vi "設定項目.vi"() -> (15 "品番・品名クラスタ_設定 _表示器":T3)   [LabVIEW 2021]
uses:
  <vilib>/Utility/config.llb/Read Key (String).vi
  <vilib>/Utility/config.llb/Read Key (U32).vi
  <vilib>/Utility/config.llb/Read Key (I32).vi
  <vilib>/Utility/config.llb/Read Key (Boolean).vi
  <vilib>/Utility/config.llb/Read Key (Path).vi
  <vilib>/Utility/config.llb/Write Key (String).vi
  <vilib>/Utility/config.llb/Write Key (Double).vi
  <vilib>/Utility/config.llb/Write Key (U32).vi
  <vilib>/Utility/config.llb/Write Key (Boolean).vi
  <vilib>/Utility/config.llb/Write Key (Path).vi
  <vilib>/Utility/config.llb/NI_LVConfig.lvlib
panel:
  out "ゲージ確認ボタンBOOL":bool
  in  "書込周期/ms":dbl
  in  "CSV項目名_リセット用":T1
  in  "CSV保存名_リセット用":string
  in  "② CSV保存名":string
  out "値転記用配列":T2[](array[typedef]) {"測定モード" items=["単発測定モード", "連続測定モード", "多点測定モード"]}
  out "G_メイン測定キャンセルボタン":bool
  in  "ゲージ確認ボタン":bool
  in  "測定ゲージ数":dbl
  in  "測定周期/ms":dbl
  in  "iniRエラーin 2":errorcluster caption="エラー入力（エラーなし）"
  out "iniエラーout":errorcluster caption="エラー入力（エラーなし）"
  in  "error in (no error)":errorcluster caption="エラー入力（エラーなし）"
  out "iniフォルダパス取得":path
  out "キューのエラー":errorcluster caption="エラー出力"
  in  "設定クラスタ_リセット":T4 {"測定モード" items=["単発測定モード", "連続測定モード"]}
  in  "CSV保存先フォルダ_リセット用":path
  in  "CSV保存先フォルダ":path
  in  "品番・品名_リセット用":T3
  in  "品番・品名クラスタ_設定":T3
  in  "使用ON/OFFボタン_リセット用":T5
  in  "初期化ボタン":bool
  in  "キャンセルして戻るボタン":bool
  in  "登録ボタン":bool
  out "iniRエラーout 2":errorcluster caption="エラー入力（エラーなし）"
  in  "CSV項目名 12":T1
  in  "CSV項目名 11":T1
  in  "CSV項目名 10":T1
  in  "CSV項目名 9":T1
  in  "CSV項目名 8":T1
  in  "CSV項目名 7":T1
  in  "CSV項目名 6":T1
  in  "CSV項目名 5":T1
  in  "CSV項目名 4":T1
  in  "CSV項目名 3":T1
  in  "CSV項目名 2":T1
  in  "CSV項目名 1":T1
  in  "設定クラスタ_設定 12":T2 {"測定モード" items=["単発測定モード", "連続測定モード", "多点測定モード"]}
  in  "使用ON/OFFボタン_設定 12":T5
  in  "キャンセルボタン 12":T6
  in  "No設定クラスタ_設定 12":T7
  in  "設定クラスタ_設定 11":T2 {"測定モード" items=["単発測定モード", "連続測定モード", "多点測定モード"]}
  in  "使用ON/OFFボタン_設定 11":T5
  in  "キャンセルボタン 11":T6
  in  "No設定クラスタ_設定 11":T7
  in  "設定クラスタ_設定 10":T2 {"測定モード" items=["単発測定モード", "連続測定モード", "多点測定モード"]}
  in  "使用ON/OFFボタン_設定 10":T5
  in  "キャンセルボタン 10":T6
  in  "No設定クラスタ_設定 10":T7
  in  "設定クラスタ_設定 9":T2 {"測定モード" items=["単発測定モード", "連続測定モード", "多点測定モード"]}
  in  "使用ON/OFFボタン_設定 9":T5
  in  "キャンセルボタン 9":T6
  in  "No設定クラスタ_設定 9":T7
  in  "設定クラスタ_設定 8":T2 {"測定モード" items=["単発測定モード", "連続測定モード", "多点測定モード"]}
  in  "使用ON/OFFボタン_設定 8":T5
  in  "キャンセルボタン 8":T6
  in  "No設定クラスタ_設定 8":T7
  in  "設定クラスタ_設定 7":T2 {"測定モード" items=["単発測定モード", "連続測定モード", "多点測定モード"]}
  in  "使用ON/OFFボタン_設定 7":T5
  in  "キャンセルボタン 7":T6
  in  "No設定クラスタ_設定 7":T7
  in  "設定クラスタ_設定 6":T2 {"測定モード" items=["単発測定モード", "連続測定モード", "多点測定モード"]}
  in  "使用ON/OFFボタン_設定 6":T5
  in  "キャンセルボタン 6":T6
  in  "No設定クラスタ_設定 6":T7
  in  "設定クラスタ_設定 5":T2 {"測定モード" items=["単発測定モード", "連続測定モード", "多点測定モード"]}
  in  "使用ON/OFFボタン_設定 5":T5
  in  "キャンセルボタン 5":T6
  in  "No設定クラスタ_設定 5":T7
  in  "設定クラスタ_設定 4":T2 {"測定モード" items=["単発測定モード", "連続測定モード", "多点測定モード"]}
  in  "使用ON/OFFボタン_設定 4":T5
  in  "キャンセルボタン 4":T6
  in  "No設定クラスタ_設定 4":T7
  in  "設定クラスタ_設定 3":T2 {"測定モード" items=["単発測定モード", "連続測定モード", "多点測定モード"]}
  in  "使用ON/OFFボタン_設定 3":T5
  in  "キャンセルボタン 3":T6
  in  "No設定クラスタ_設定 3":T7
  in  "設定クラスタ_設定 2":T2 {"測定モード" items=["単発測定モード", "連続測定モード", "多点測定モード"]}
  in  "使用ON/OFFボタン_設定 2":T5
  in  "キャンセルボタン 2":T6
  in  "No設定クラスタ_設定 2":T7
  in  "設定クラスタ_設定1":T2 {"測定モード" items=["単発測定モード", "連続測定モード", "多点測定モード"]}
  in  "キャンセルボタン1":T6
  in  "使用ON/OFFボタン_設定1":T5
  in  "No設定クラスタ_設定1":T7
  # "設定項目画面"
  # "データ収集タイミング"
  # "※全入力クリアボタンでリセットしない仕様です。"
  # "①"
  # "⑬\n測定画面\nON/OFF"
  # "⑦規格"
  # "⑨上限"
  # "⑪同時測定\nゲージNO."
  # "⑭ゲージ\nポートNo."
  # "入力\nクリア"
  # "⑮測定\nON/OFF"
  # "⑯CSVヘッダー名"
  # "⑤No."
  # "⑥品質チェック項目"
  # "⑫測定モード"
  # "値"
  # "⑧単位"
  # "⑩下限"
  # "-"
  # "品番"
  # "品名"
  # "-"
  # "品番"
  # "品名"
  # "-"
  # "品番"
  # "品名"
  # "③"
  # "④"
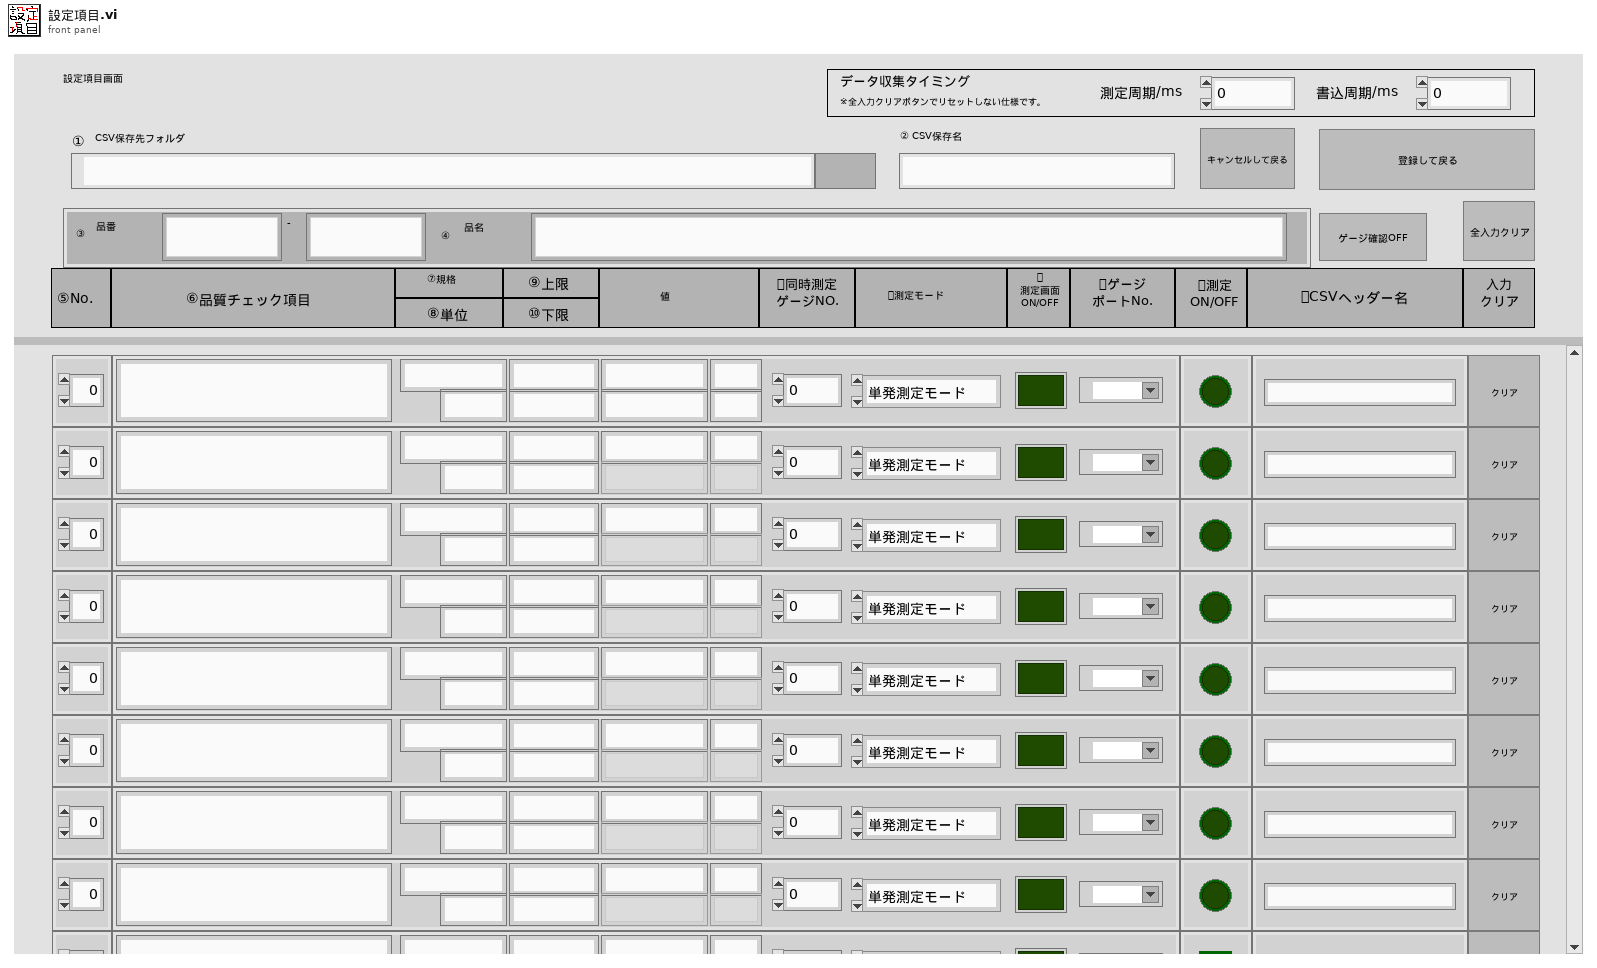
[diagram p1: front panel]
types:
  T1 = typedef "CSV項目名入力.ctl" = cluster{"CSV項目名":string}
  T2 = typedef "設定全項目制御器.ctl" = cluster{"規格":string, "規格上限":string, "規格下限":string, "ポートNo.":dbl, "測定モード":u16, "規格単位":string, "品質チェック項目":string, "測定周期":dbl, "実測値MAX":string, "実測値MIN":string, "実測値(MAX)":string, "実測値(MIN)":string, "測定画面表示ボタン":bool, "ゲージポートNo":refnum<visa-resource-name>}
  T3 = typedef "品番・品名選択用.ctl" = cluster{"品名":string, "品番前":string, "品番後":string}
  T4 = cluster{"規格":string, "規格上限":string, "規格下限":string, "ポートNo.":dbl, "測定モード":u16, "規格単位":string, "品質チェック項目":string, "測定周期":dbl, "実測値MAX":string, "実測値MIN":string, "実測値(MAX)":string, "実測値(MIN)":string, "測定画面表示ボタン":bool, "ゲージポートNo":refnum<visa-resource-name>}
  T5 = typedef "ONOFFボタン制御器.ctl" = cluster{"使用ON/OFF":bool}
  T6 = typedef "キャンセルボタン制御器.ctl" = bool
  T7 = typedef "CH設定表示器.ctl" = cluster{"No. ":dbl}
  T8 = enum8{"Enabled", "Disabled", "Disabled and Grayed Out"}
  T9 = typedef "NI_LVConfig.lvlib/Config Data RefNum.ctl" = refnum<k1>
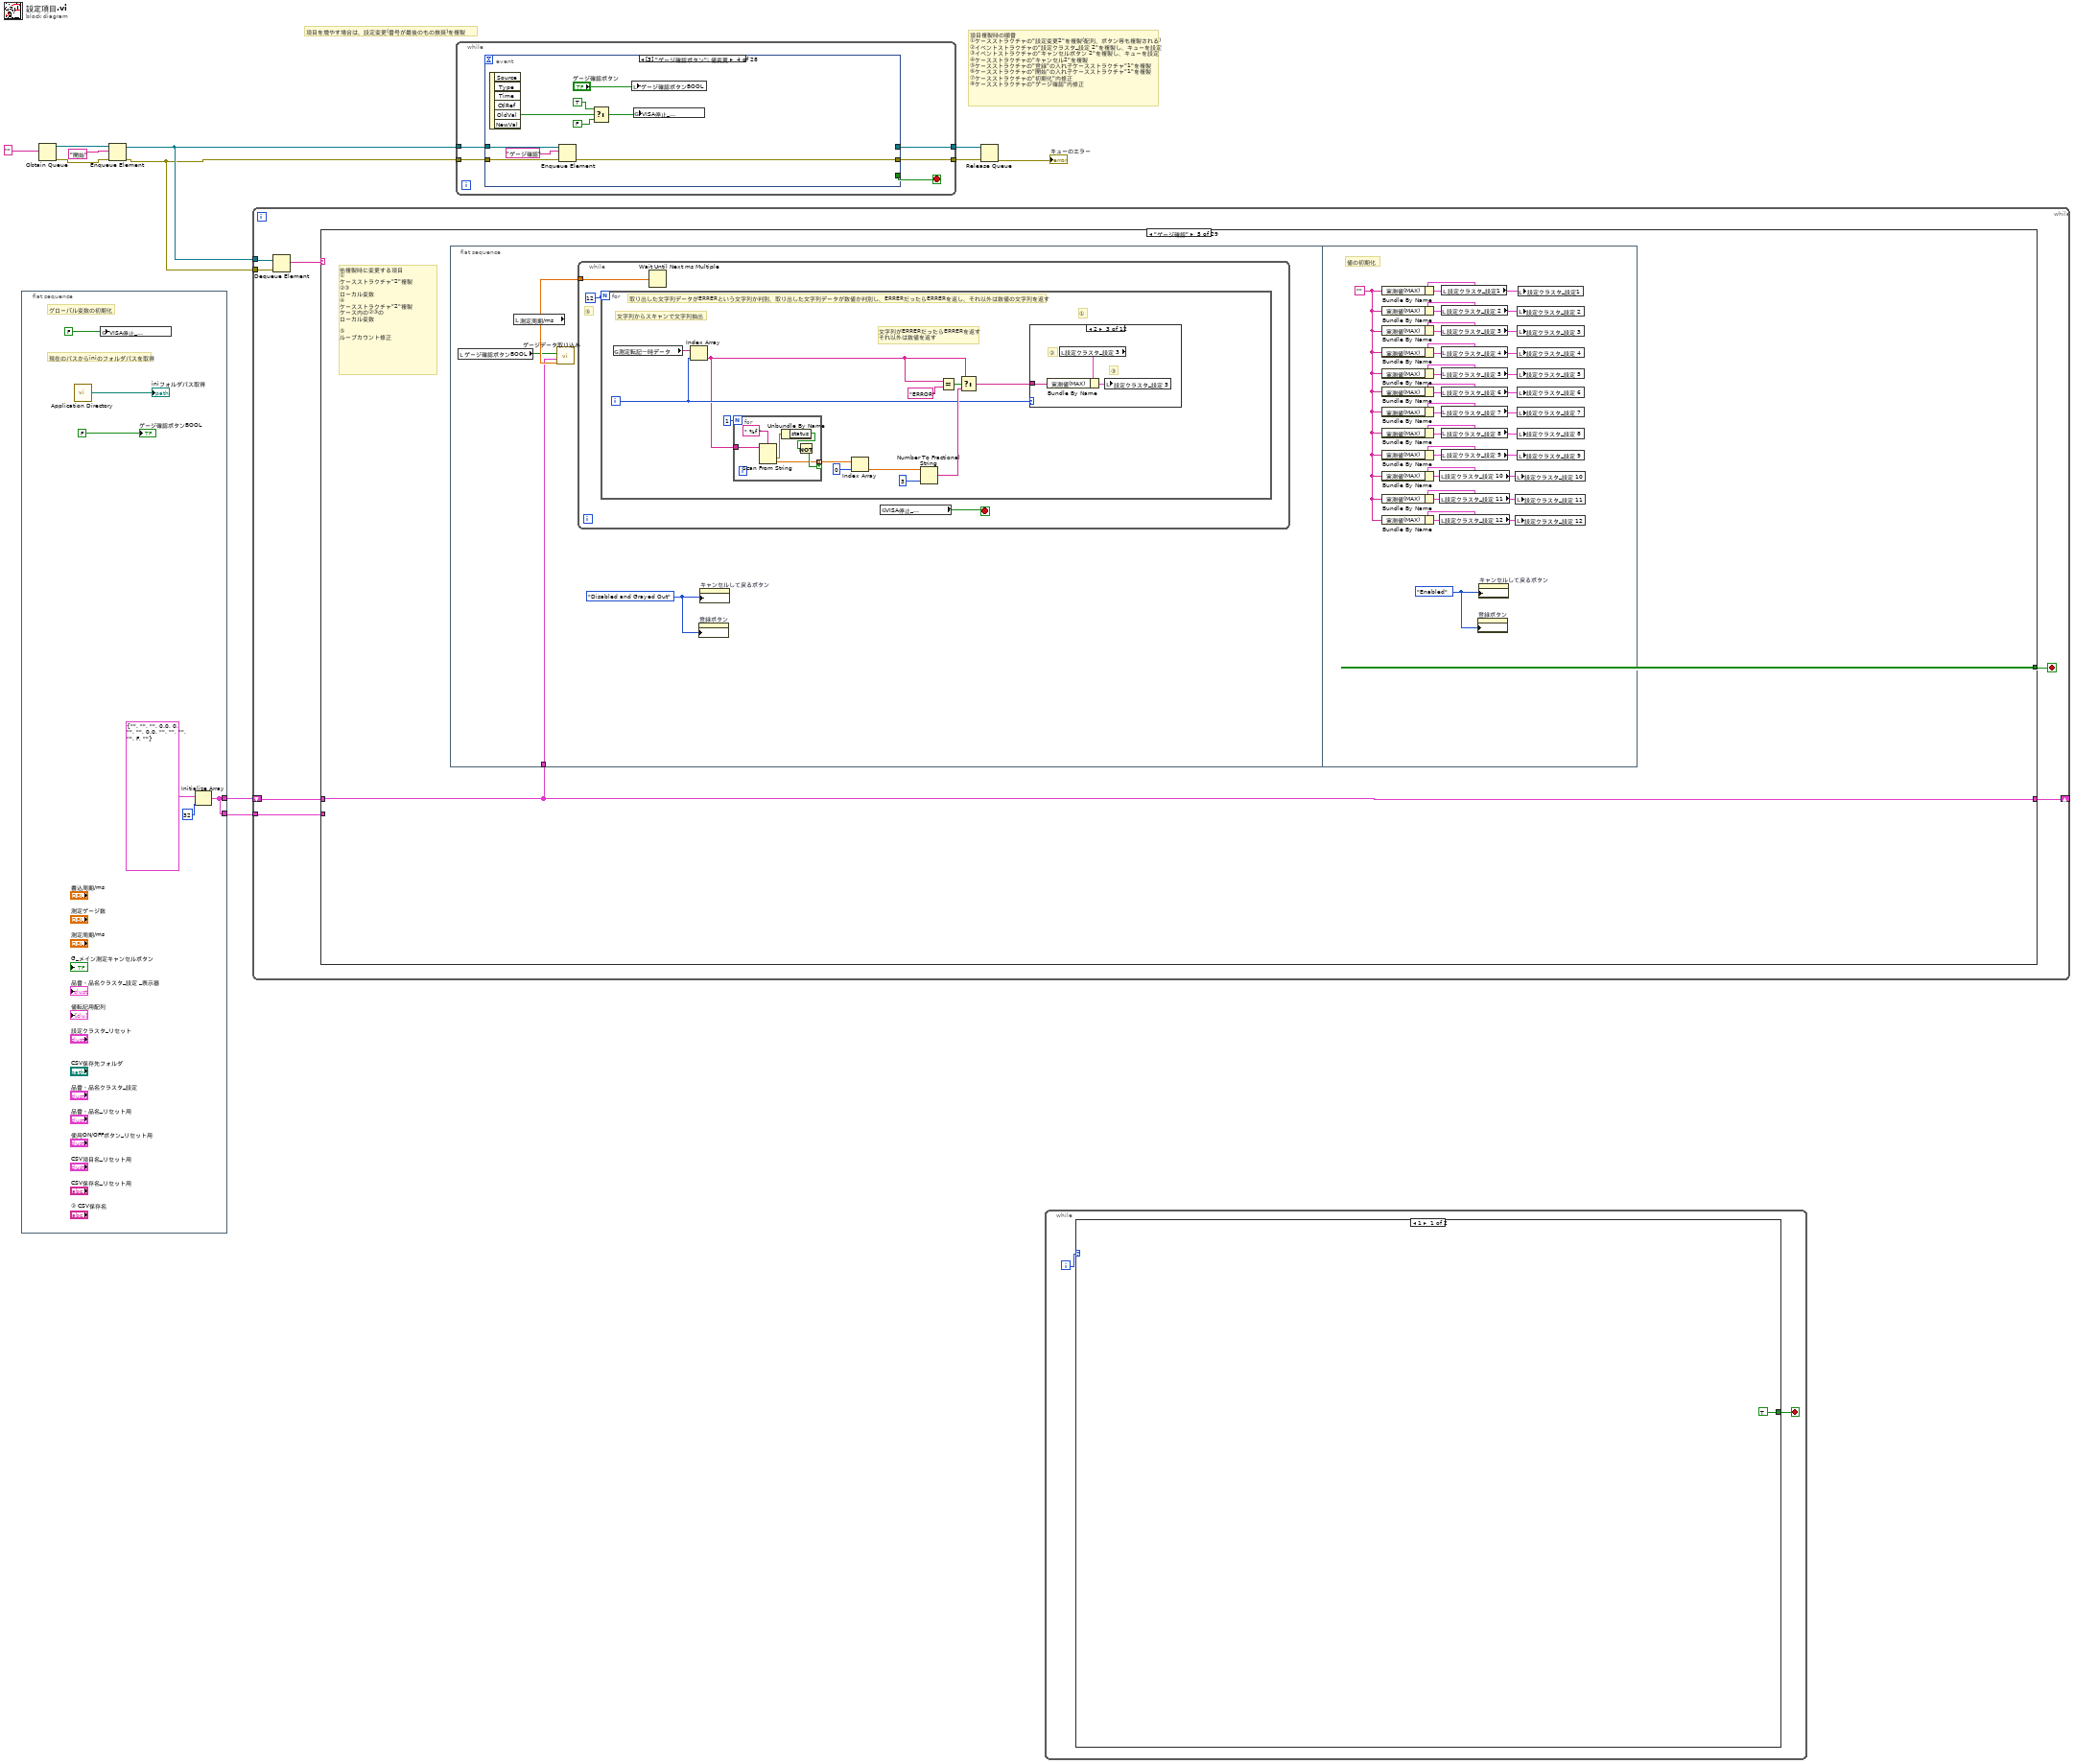
[diagram p0: block diagram]
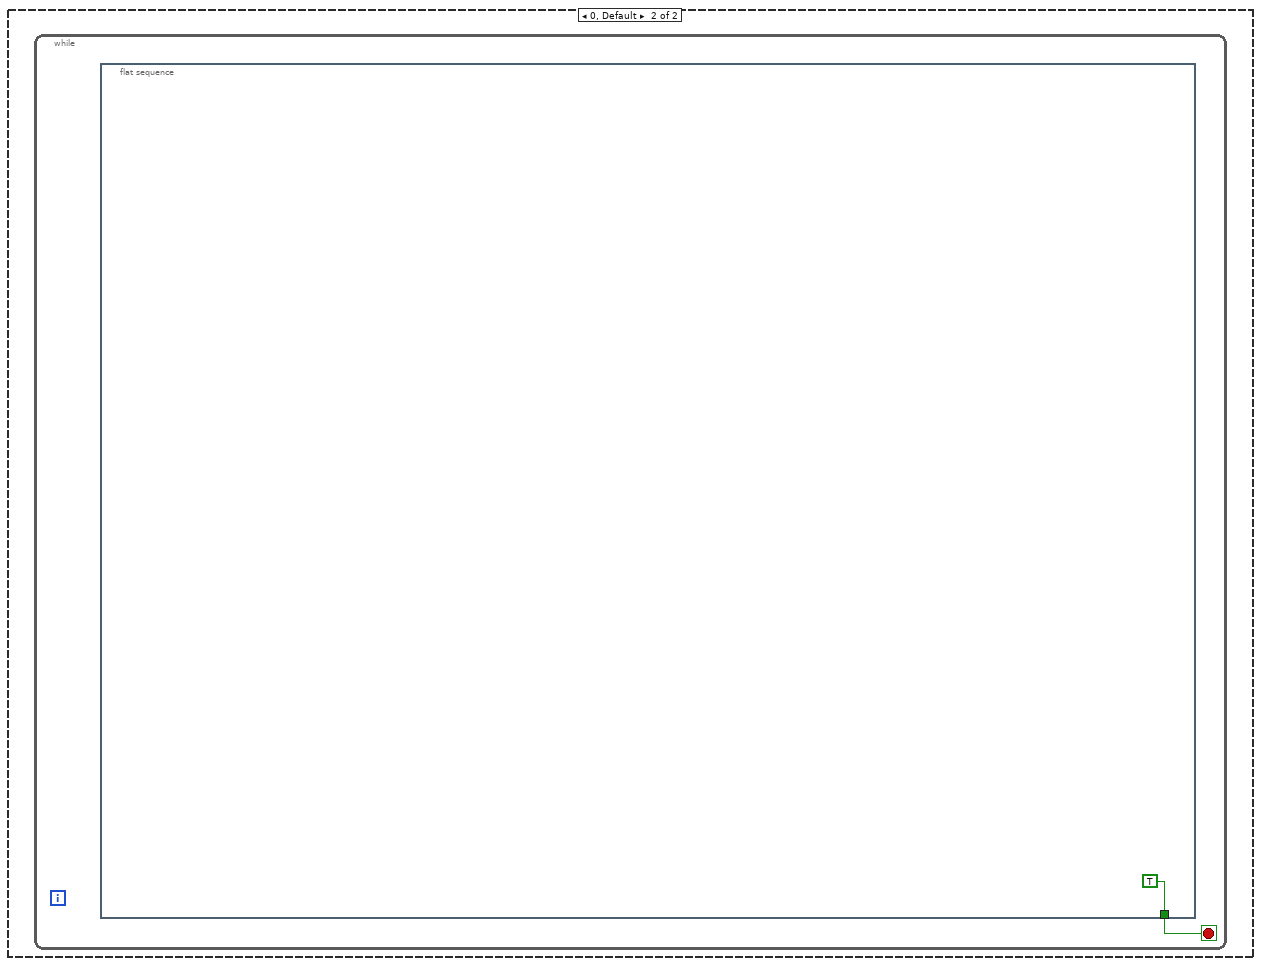
[diagram p2: hidden frame]
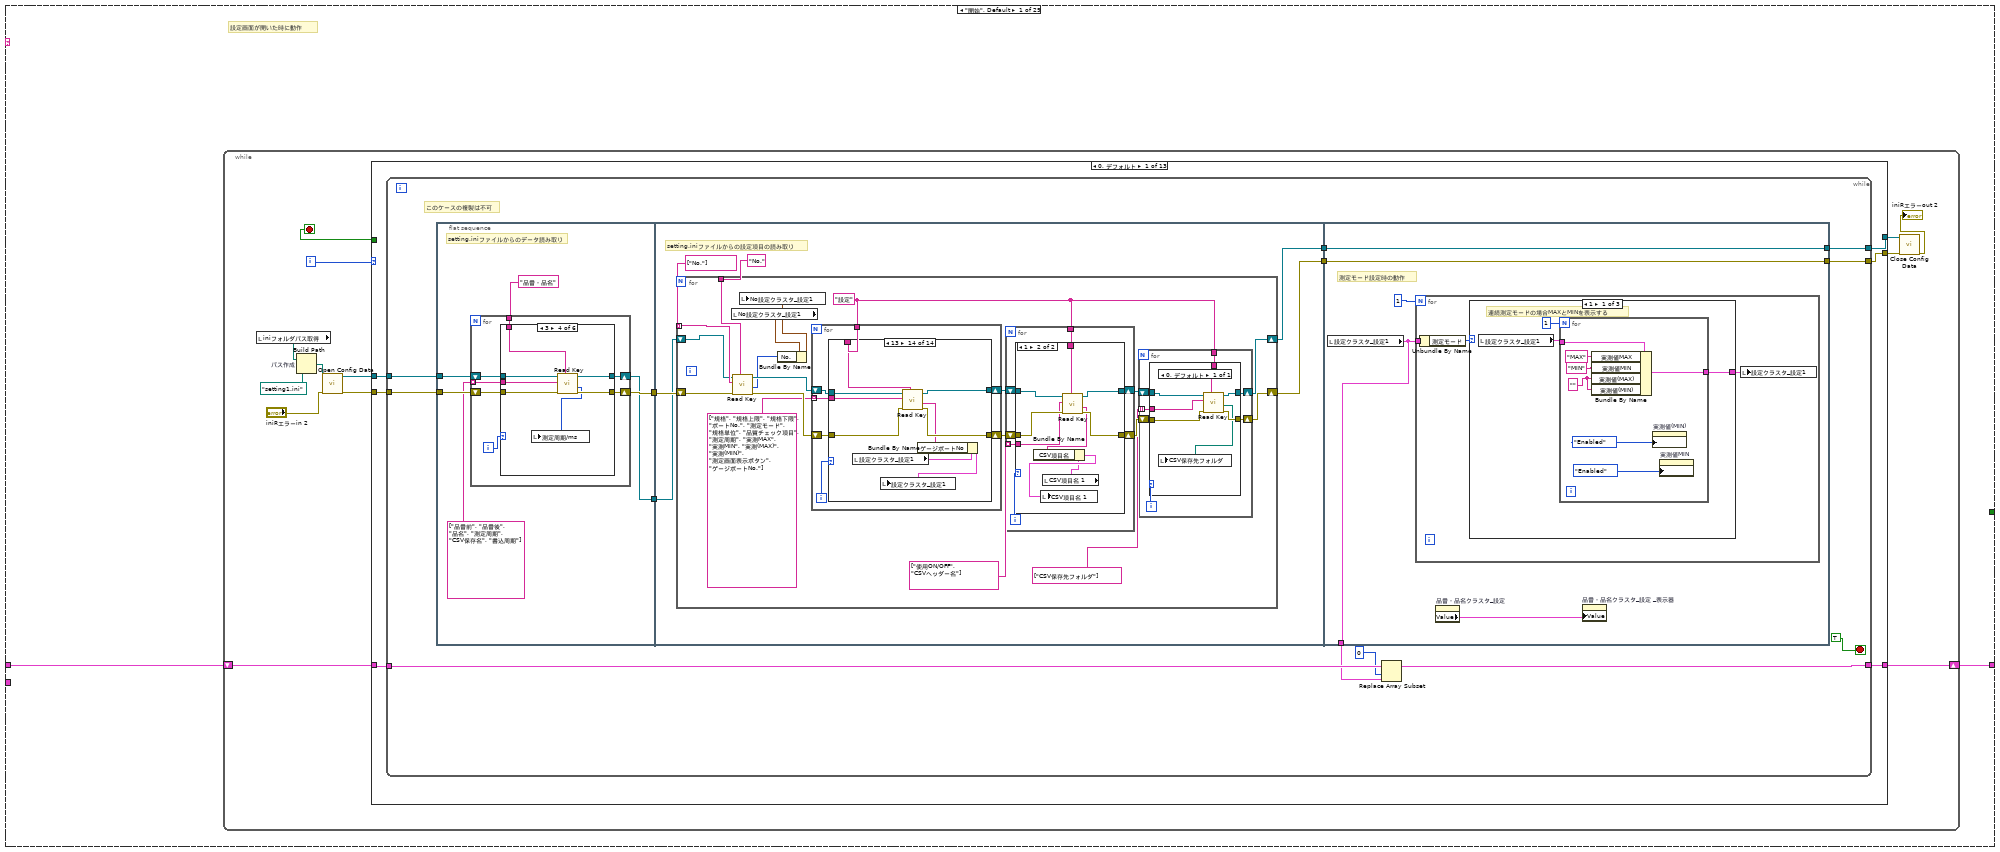
[diagram p3: hidden frame]
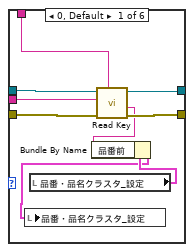
[diagram p4: hidden frame]
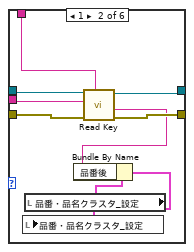
[diagram p5: hidden frame]
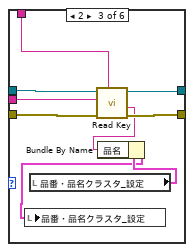
[diagram p6: hidden frame]
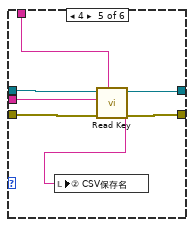
[diagram p7: hidden frame]
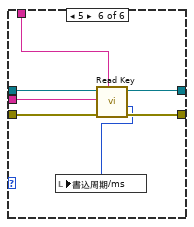
[diagram p8: hidden frame]
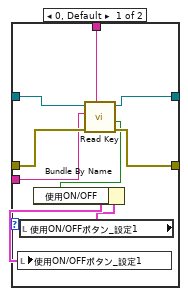
[diagram p9: hidden frame]
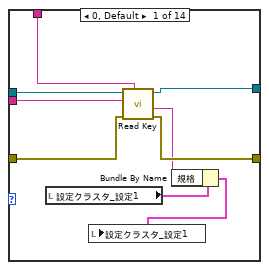
[diagram p10: hidden frame]
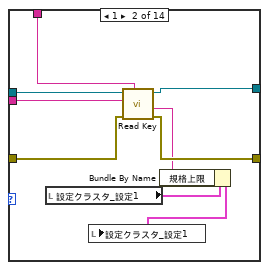
[diagram p11: hidden frame]
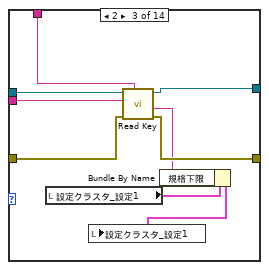
[diagram p12: hidden frame]
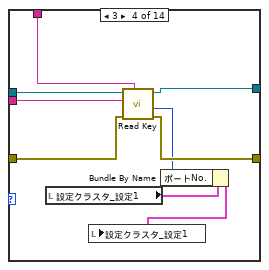
[diagram p13: hidden frame]
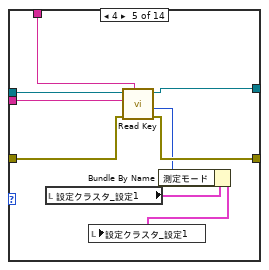
[diagram p14: hidden frame]
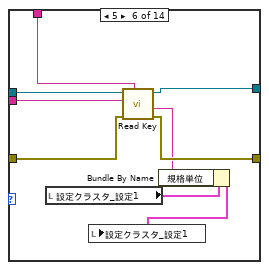
[diagram p15: hidden frame]
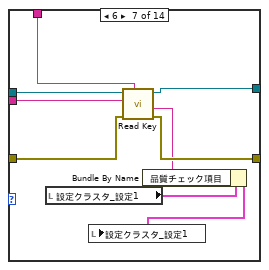
[diagram p16: hidden frame]
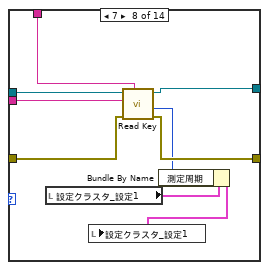
[diagram p17: hidden frame]
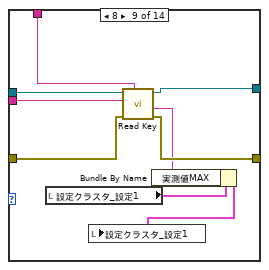
[diagram p18: hidden frame]
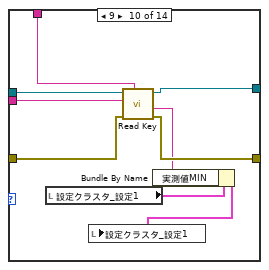
[diagram p19: hidden frame]
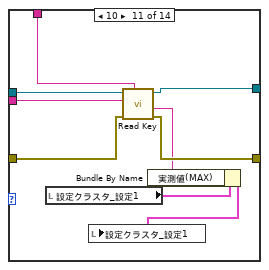
[diagram p20: hidden frame]
diagram:
  # "項目複製時の順番\n①ケースストラクチャの\"設定変更2\"を複製(配列、ボタン等も複製される)\n②イベントストラクチャの\"設定クラスタ_設定 2\"を複製し、キューを設定\n③イベントストラクチャの\"キャンセルボタン 2\"を複製し、キューを設定\n④ケースストラクチャの\"キャンセル2\"を複製\n⑤ケースストラクチャの\"登録\"の入れ子ケースストラクチャ\"1\"を複製\n⑥ケースストラクチャの\"開始\"の入れ子ケースストラクチャ\"1\"を複製\n⑦ケースストラクチャの\"初期化\"内修正\n⑧ケースストラクチャの\"ゲージ確認\"内修正"
  # "項目を増やす場合は、設定変更(番号が最後のもの推奨)を複製"
  n1 = flat-sequence {
    tunnel: [w14] -> w8
    tunnel: [w14] -> w7
    frame #0 {
      # "グローバル変数の初期化"
      # "現在のパスからiniのフォルダパスを取得"
      n2 = call <vilib>:"Application Directory.vi"() -> ("Application Directory"=→"iniフォルダパス取得":path)
      n3 = global write "VISA停止_G.vi" "VISA停止_\nグローバル"(FALSE) -> ()
      n4 = Initialize Array(T2 {"規格"="", "規格上限"="", "規格下限"="", "ポートNo."=0.0, "測定モード"=0, "規格単位"="", "品質チェック項目"="", "測定周期"=0.0, "実測値MAX"="", "実測値MIN"="", "実測値(MAX)"="", "実測値(MIN)"="", "測定画面表示ボタン"=FALSE, "ゲージポートNo"=""} ("メイン設定_設定"), 32) -> (w14:T2[])
      "ゲージ確認ボタンBOOL" <- FALSE
    }
  }
  n5 = Obtain Queue(element data type="") -> (queue out=w3:refnum<queue>, error out=w1:errorcluster)  [unwired: 4 in, 1 out]
  n6 = Enqueue Element(queue=w3, element="開始", error in (no error)=w1) -> (queue out=w6:refnum<queue>, error out=w5:errorcluster)  [unwired: 1 in, 1 out]
  n7 = while {
    tunnel: w6 -> [w23]
    tunnel: w5 -> [w21]
    shift-right: [w19] -> _
    shift-left: w8 -> [w20]
    tunnel: w7 -> [w18]
    stop <- w22 stop-if-true
    n8 = Dequeue Element(queue=w23, error in (no error)=w21) -> (element=w24:string)  [unwired: 1 in, 3 out]
    n9 = case shown="\"ゲージ確認\"" w24 {
      tunnel: [_ TRUE TRUE _ _ _ _ _ _ _ _ _ _ _ _ _ _ _ _ _ _ _ _ _ _ _ _ _ _] -> w22
      tunnel: w20 -> [w26 w2548 _ _ w3041 w3133 w3139 w3145 w3151 w3157 w3163 w3169 w3175 w3181 w3187 w3193 w3199 w3204 w3245 w3285 w3325 w3365 w3405 w3445 w3485 w3525 w3565 w3605 w3645]
      tunnel: [w25 w2547 _ w3038 w3041 w3132 w3138 w3144 w3150 w3156 w3162 w3168 w3174 w3180 w3186 w3192 w3198 w3201 w3242 w3282 w3322 w3362 w3402 w3442 w3482 w3522 w3562 w3602 w3642] -> w19
      tunnel: w18 -> [_ _ _ w3038 _ _ _ _ _ _ _ _ _ _ _ _ _ _ _ _ _ _ _ _ _ _ _ _ _]
      frame "開始", Default {
        # "設定画面が開いた時に動作"
        n10 = while {
          shift-right: [w28] -> w25
          shift-left: w26 -> [w29]
          i -> [w39]
          stop <- w27 stop-if-true
          n11 = local read "iniフォルダパス取得"() -> (w38:path)
          n12 = Build Path "パス作成"(base path=w38, name or relative path=path "setting1.ini") -> (appended path=w37:path)
          n13 = call <vilib>:"Open Config Data.vi"("error in (no error)"="iniRエラーin 2", "configuration file path"=w37) -> ("error out"=w34:errorcluster, "refnum"=w33:T9)  [unwired: 1 in, 7 out]
          n14 = case shown="0, デフォルト" w39 {
            tunnel: w34 -> [w42 w365 w564 w763 w962 w1161 w1360 w1559 w1758 w1957 w2156 w2355 _]
            tunnel: w33 -> [w43 w364 w563 w762 w961 w1160 w1359 w1558 w1757 w1956 w2155 w2354 _]
            tunnel: [w44 w363 w562 w761 w960 w1159 w1358 w1557 w1756 w1955 w2154 w2353 _] -> w32
            tunnel: [w45 w362 w561 w760 w959 w1158 w1357 w1556 w1755 w1954 w2153 w2352 _] -> w31
            tunnel: w29 -> [w40 w360 w559 w758 w957 w1156 w1355 w1554 w1753 w1952 w2151 w2350 w2545]
            tunnel: [w41 w361 w560 w759 w958 w1157 w1356 w1555 w1754 w1953 w2152 w2351 w2545] -> w28
            tunnel: [_ _ _ _ _ _ _ _ _ _ _ _ TRUE] -> w27
            frame 0, Default {
              n15 = while {
                tunnel: [w57] -> w45
                tunnel: [w56] -> w44
                tunnel: w43 -> [w55]
                tunnel: w42 -> [w54]
                tunnel: [w53] -> w41
                tunnel: w40 -> [w52]
                stop <- TRUE stop-if-true
                # "このケースの複製は不可"
                n16 = flat-sequence {
                  tunnel: [w63] -> w51
                  tunnel: [w62] -> w50
                  tunnel: w55 -> [w61]
                  tunnel: w54 -> [w60]
                  tunnel: w51 -> [w123]
                  tunnel: w50 -> [w122]
                  tunnel: [w121] -> w49
                  tunnel: [w120] -> w48
                  tunnel: w49 -> [w320]
                  tunnel: [w320] -> w57
                  tunnel: w48 -> [w319]
                  tunnel: [w319] -> w56
                  tunnel: [w317] -> w47
                  frame #0 {
                    # "setting.iniファイルからのデータ読み取り"
                    n17 = for {
                      tunnel: string[] ["品番前", "品番後", "品名", "測定周期", "CSV保存名", "書込周期"] -> [w70] mode=indexing
                      shift-right: [w69] -> w62
                      shift-left: w61 -> [w68]
                      tunnel: "品番・品名" -> [w67]
                      shift-right: [w65] -> w63
                      shift-left: w60 -> [w66]
                      i -> [w71]
                      n18 = case shown="3" w71 {
                        tunnel: w70 -> [w80 w89 w98 w105 w112 w119]
                        tunnel: [w79 w87 w97 w104 w111 w118] -> w69
                        tunnel: w68 -> [w78 w88 w96 w103 w110 w117]
                        tunnel: w67 -> [w77 w86 w95 w102 w109 w116]
                        tunnel: w66 -> [w76 w85 w94 w101 w108 w115]
                        tunnel: [w75 w84 w93 w100 w107 w114] -> w65
                        frame 0, Default {
                          n19 = local read "品番・品名クラスタ_設定"() -> (w73:T3)
                          n20 = call-poly <vilib>:"Read Key.vi"("section"=w77, "error in (no error)"=w76, "key"=w80, "refnum"=w78) -> ("error out"=w75:errorcluster, "value"=w74:string, "refnum out"=w79:T9)  [unwired: 4 in, 1 out]
                          n21 = Bundle By Name(cluster=w73, "品番前"=w74) -> (w72:T3)
                          n22 = local write "品番・品名クラスタ_設定"(w72) -> ()
                        }
                        frame 1 {
                          n23 = local read "品番・品名クラスタ_設定"() -> (w82:T3)
                          n24 = call-poly <vilib>:"Read Key.vi"("section"=w86, "error in (no error)"=w85, "key"=w89, "refnum"=w88) -> ("error out"=w84:errorcluster, "value"=w83:string, "refnum out"=w87:T9)  [unwired: 4 in, 1 out]
                          n25 = Bundle By Name(cluster=w82, "品番後"=w83) -> (w81:T3)
                          n26 = local write "品番・品名クラスタ_設定"(w81) -> ()
                        }
                        frame 2 {
                          n27 = local read "品番・品名クラスタ_設定"() -> (w91:T3)
                          n28 = call-poly <vilib>:"Read Key.vi"("section"=w95, "error in (no error)"=w94, "key"=w98, "refnum"=w96) -> ("error out"=w93:errorcluster, "value"=w92:string, "refnum out"=w97:T9)  [unwired: 4 in, 1 out]
                          n29 = Bundle By Name(cluster=w91, "品名"=w92) -> (w90:T3)
                          n30 = local write "品番・品名クラスタ_設定"(w90) -> ()
                        }
                        frame 3 {
                          n31 = call-poly <vilib>:"Read Key.vi"("section"=w102, "error in (no error)"=w101, "key"=w105, "refnum"=w103) -> ("error out"=w100:errorcluster, "value"=w99:u32, "refnum out"=w104:T9)  [unwired: 4 in, 1 out]
                          n32 = local write "測定周期/ms"(w99) -> ()
                        }
                        frame 4 {
                          n33 = call-poly <vilib>:"Read Key.vi"("section"=w109, "error in (no error)"=w108, "key"=w112, "refnum"=w110) -> ("error out"=w107:errorcluster, "value"=w106:string, "refnum out"=w111:T9)  [unwired: 4 in, 1 out]
                          n34 = local write "② CSV保存名"(w106) -> ()
                        }
                        frame 5 {
                          n35 = call-poly <vilib>:"Read Key.vi"("section"=w116, "error in (no error)"=w115, "key"=w119, "refnum"=w117) -> ("error out"=w114:errorcluster, "value"=w113:u32, "refnum out"=w118:T9)  [unwired: 4 in, 1 out]
                          n36 = local write "書込周期/ms"(w113) -> ()
                        }
                      }
                    }
                  }
                  frame #1 {
                    # "setting.iniファイルからの設定項目の読み取り"
                    n37 = for {
                      shift-right: [w141] -> w121
                      shift-left: w122 -> [w142]
                      tunnel: string[] ["No."] -> [w144] mode=indexing
                      tunnel: "No." -> [w143]
                      shift-right: [w139] -> w120
                      shift-left: w123 -> [w140]
                      w128 = "設定"
                      n38 = local read "No設定クラスタ_設定1"() -> (w132:T7)
                      n39 = call-poly <vilib>:"Read Key.vi"("section"=w143, "error in (no error)"=w140, "key"=w144, "refnum"=w142) -> ("error out"=w136:errorcluster, "value"=w133:i32, "refnum out"=w138:T9)  [unwired: 4 in, 1 out]
                      n40 = Bundle By Name(cluster=w132, "No."=w133) -> (w134:T7)
                      n41 = local write "No設定クラスタ_設定1"(w134) -> ()
                      n42 = for {
                        shift-right: [w188] -> w137
                        shift-left: w138 -> [w190]
                        tunnel: w128 -> [w189]
                        shift-right: [w185] -> w135
                        shift-left: w136 -> [w186]
                        tunnel: string[] ["規格", "規格上限", "規格下限", "ポートNo.", "測定モード", "規格単位", "品質チェック項目", "測定周期", "実測MAX", "実測MIN", "実測(MAX)", "実測(MIN)", "測定画面表示ボタン", "ゲージポートNo."] -> [w184] mode=indexing
                        i -> [w187]
                        n43 = case shown="13" w187 {
                          tunnel: w190 -> [w199 w208 w217 w226 w235 w244 w253 w262 w271 w280 w289 w298 w307 w316]
                          tunnel: [w198 w207 w216 w225 w234 w243 w252 w261 w270 w279 w288 w297 w306 w315] -> w188
                          tunnel: w189 -> [w197 w206 w215 w224 w233 w242 w251 w260 w269 w278 w287 w296 w305 w314]
                          tunnel: w186 -> [w196 w205 w214 w223 w232 w241 w250 w259 w268 w277 w286 w295 w304 w313]
                          tunnel: [w195 w204 w213 w222 w231 w240 w249 w258 w267 w276 w285 w294 w303 w312] -> w185
                          tunnel: w184 -> [w191 w200 w209 w218 w227 w236 w245 w254 w263 w272 w281 w290 w299 w308]
                          frame 0, Default {
                            n44 = local read "設定クラスタ_設定1"() -> (w193:T2)
                            n45 = call-poly <vilib>:"Read Key.vi"("section"=w197, "error in (no error)"=w196, "key"=w191, "refnum"=w199) -> ("error out"=w195:errorcluster, "value"=w194:string, "refnum out"=w198:T9)  [unwired: 4 in, 1 out]
                            n46 = Bundle By Name(cluster=w193, "規格"=w194) -> (w192:T2)
                            n47 = local write "設定クラスタ_設定1"(w192) -> ()
                          }
                          frame 1 {
                            n48 = local read "設定クラスタ_設定1"() -> (w202:T2)
                            n49 = call-poly <vilib>:"Read Key.vi"("section"=w206, "error in (no error)"=w205, "key"=w200, "refnum"=w208) -> ("error out"=w204:errorcluster, "value"=w203:string, "refnum out"=w207:T9)  [unwired: 4 in, 1 out]
                            n50 = Bundle By Name(cluster=w202, "規格上限"=w203) -> (w201:T2)
                            n51 = local write "設定クラスタ_設定1"(w201) -> ()
                          }
                          frame 2 {
                            n52 = local read "設定クラスタ_設定1"() -> (w211:T2)
                            n53 = call-poly <vilib>:"Read Key.vi"("section"=w215, "error in (no error)"=w214, "key"=w209, "refnum"=w217) -> ("error out"=w213:errorcluster, "value"=w212:string, "refnum out"=w216:T9)  [unwired: 4 in, 1 out]
                            n54 = Bundle By Name(cluster=w211, "規格下限"=w212) -> (w210:T2)
                            n55 = local write "設定クラスタ_設定1"(w210) -> ()
                          }
                          frame 3 {
                            n56 = local read "設定クラスタ_設定1"() -> (w220:T2)
                            n57 = call-poly <vilib>:"Read Key.vi"("section"=w224, "error in (no error)"=w223, "key"=w218, "refnum"=w226) -> ("error out"=w222:errorcluster, "value"=w221:i32, "refnum out"=w225:T9)  [unwired: 4 in, 1 out]
                            n58 = Bundle By Name(cluster=w220, "ポートNo."=w221) -> (w219:T2)
                            n59 = local write "設定クラスタ_設定1"(w219) -> ()
                          }
                          frame 4 {
                            n60 = local read "設定クラスタ_設定1"() -> (w229:T2)
                            n61 = call-poly <vilib>:"Read Key.vi"("section"=w233, "error in (no error)"=w232, "key"=w227, "refnum"=w235) -> ("error out"=w231:errorcluster, "value"=w230:i32, "refnum out"=w234:T9)  [unwired: 4 in, 1 out]
                            n62 = Bundle By Name(cluster=w229, "測定モード"=w230) -> (w228:T2)
                            n63 = local write "設定クラスタ_設定1"(w228) -> ()
                          }
                          frame 5 {
                            n64 = local read "設定クラスタ_設定1"() -> (w238:T2)
                            n65 = call-poly <vilib>:"Read Key.vi"("section"=w242, "error in (no error)"=w241, "key"=w236, "refnum"=w244) -> ("error out"=w240:errorcluster, "value"=w239:string, "refnum out"=w243:T9)  [unwired: 4 in, 1 out]
                            n66 = Bundle By Name(cluster=w238, "規格単位"=w239) -> (w237:T2)
                            n67 = local write "設定クラスタ_設定1"(w237) -> ()
                          }
                          frame 6 {
                            n68 = local read "設定クラスタ_設定1"() -> (w247:T2)
                            n69 = call-poly <vilib>:"Read Key.vi"("section"=w251, "error in (no error)"=w250, "key"=w245, "refnum"=w253) -> ("error out"=w249:errorcluster, "value"=w248:string, "refnum out"=w252:T9)  [unwired: 4 in, 1 out]
                            n70 = Bundle By Name(cluster=w247, "品質チェック項目"=w248) -> (w246:T2)
                            n71 = local write "設定クラスタ_設定1"(w246) -> ()
                          }
                          frame 7 {
                            n72 = local read "設定クラスタ_設定1"() -> (w256:T2)
                            n73 = call-poly <vilib>:"Read Key.vi"("section"=w260, "error in (no error)"=w259, "key"=w254, "refnum"=w262) -> ("error out"=w258:errorcluster, "value"=w257:i32, "refnum out"=w261:T9)  [unwired: 4 in, 1 out]
                            n74 = Bundle By Name(cluster=w256, "測定周期"=w257) -> (w255:T2)
                            n75 = local write "設定クラスタ_設定1"(w255) -> ()
                          }
                          frame 8 {
                            n76 = local read "設定クラスタ_設定1"() -> (w265:T2)
                            n77 = call-poly <vilib>:"Read Key.vi"("section"=w269, "error in (no error)"=w268, "key"=w263, "refnum"=w271) -> ("error out"=w267:errorcluster, "value"=w266:string, "refnum out"=w270:T9)  [unwired: 4 in, 1 out]
                            n78 = Bundle By Name(cluster=w265, "実測値MAX"=w266) -> (w264:T2)
                            n79 = local write "設定クラスタ_設定1"(w264) -> ()
                          }
                          frame 9 {
                            n80 = local read "設定クラスタ_設定1"() -> (w274:T2)
                            n81 = call-poly <vilib>:"Read Key.vi"("section"=w278, "error in (no error)"=w277, "key"=w272, "refnum"=w280) -> ("error out"=w276:errorcluster, "value"=w275:string, "refnum out"=w279:T9)  [unwired: 4 in, 1 out]
                            n82 = Bundle By Name(cluster=w274, "実測値MIN"=w275) -> (w273:T2)
                            n83 = local write "設定クラスタ_設定1"(w273) -> ()
                          }
                          frame 10 {
                            n84 = local read "設定クラスタ_設定1"() -> (w283:T2)
                            n85 = call-poly <vilib>:"Read Key.vi"("section"=w287, "error in (no error)"=w286, "key"=w281, "refnum"=w289) -> ("error out"=w285:errorcluster, "value"=w284:string, "refnum out"=w288:T9)  [unwired: 4 in, 1 out]
                            n86 = Bundle By Name(cluster=w283, "実測値(MAX)"=w284) -> (w282:T2)
                            n87 = local write "設定クラスタ_設定1"(w282) -> ()
                          }
                          frame 11 {
                            n88 = local read "設定クラスタ_設定1"() -> (w292:T2)
                            n89 = call-poly <vilib>:"Read Key.vi"("section"=w296, "error in (no error)"=w295, "key"=w290, "refnum"=w298) -> ("error out"=w294:errorcluster, "value"=w293:string, "refnum out"=w297:T9)  [unwired: 4 in, 1 out]
                            n90 = Bundle By Name(cluster=w292, "実測値(MIN)"=w293) -> (w291:T2)
                            n91 = local write "設定クラスタ_設定1"(w291) -> ()
                          }
                          frame 12 {
                            n92 = local read "設定クラスタ_設定1"() -> (w301:T2)
                            n93 = call-poly <vilib>:"Read Key.vi"("section"=w305, "error in (no error)"=w304, "key"=w299, "refnum"=w307) -> ("error out"=w303:errorcluster, "value"=w302:bool, "refnum out"=w306:T9)  [unwired: 4 in, 1 out]
                            n94 = Bundle By Name(cluster=w301, "測定画面表示ボタン"=w302) -> (w300:T2)
                            n95 = local write "設定クラスタ_設定1"(w300) -> ()
                          }
                          frame 13 {
                            n96 = local read "設定クラスタ_設定1"() -> (w310:T2)
                            n97 = call-poly <vilib>:"Read Key.vi"("section"=w314, "error in (no error)"=w313, "key"=w308, "refnum"=w316) -> ("error out"=w312:errorcluster, "value"=w311:string, "refnum out"=w315:T9)  [unwired: 4 in, 1 out]
                            n98 = Bundle By Name(cluster=w310, "ゲージポートNo"=w311) -> (w309:T2)
                            n99 = local write "設定クラスタ_設定1"(w309) -> ()
                          }
                        }
                      }
                      n100 = for {
                        shift-right: [w165] -> w130
                        shift-left: w137 -> [w163]
                        tunnel: w128 -> [w162]
                        shift-right: [w160] -> w129
                        shift-left: w135 -> [w161]
                        tunnel: string[] ["使用ON/OFF", "CSVヘッダー名"] -> [w159] mode=indexing
                        i -> [w164]
                        n101 = case shown="1" w164 {
                          tunnel: [w174 w183] -> w165
                          tunnel: w163 -> [w173 w182]
                          tunnel: w162 -> [w172 w181]
                          tunnel: w161 -> [w171 w180]
                          tunnel: [w170 w179] -> w160
                          tunnel: w159 -> [w166 w175]
                          frame 0, Default {
                            n102 = local read "使用ON/OFFボタン_設定1"() -> (w167:T5)
                            n103 = call-poly <vilib>:"Read Key.vi"("section"=w172, "error in (no error)"=w171, "key"=w166, "refnum"=w173) -> ("error out"=w170:errorcluster, "value"=w169:bool, "refnum out"=w174:T9)  [unwired: 4 in, 1 out]
                            n104 = Bundle By Name(cluster=w167, "使用ON/OFF"=w169) -> (w168:T5)
                            n105 = local write "使用ON/OFFボタン_設定1"(w168) -> ()
                          }
                          frame 1 {
                            n106 = local read "CSV項目名 1"() -> (w176:T1)
                            n107 = call-poly <vilib>:"Read Key.vi"("section"=w181, "error in (no error)"=w180, "key"=w175, "refnum"=w182) -> ("error out"=w179:errorcluster, "value"=w178:string, "refnum out"=w183:T9)  [unwired: 4 in, 1 out]
                            n108 = Bundle By Name(cluster=w176, "CSV項目名"=w178) -> (w177:T1)
                            n109 = local write "CSV項目名 1"(w177) -> ()
                          }
                        }
                      }
                      n110 = for {
                        tunnel: string[] ["CSV保存先フォルダ"] -> [w150] mode=indexing
                        shift-right: [w147] -> w141
                        shift-left: w130 -> [w148]
                        tunnel: w128 -> [w149]
                        shift-right: [w146] -> w139
                        shift-left: w129 -> [w145]
                        i -> [w151]
                        n111 = case shown="0, デフォルト" w151 {
                          tunnel: w150 -> [w154]
                          tunnel: w149 -> [w158]
                          tunnel: w148 -> [w155]
                          tunnel: [w157] -> w147
                          tunnel: [w156] -> w146
                          tunnel: w145 -> [w153]
                          frame 0, Default {
                            n112 = call-poly <vilib>:"Read Key.vi"("section"=w158, "error in (no error)"=w153, "key"=w154, "refnum"=w155) -> ("error out"=w156:errorcluster, "value"=w152:path, "refnum out"=w157:T9)  [unwired: 4 in, 1 out]
                            n113 = local write "CSV保存先フォルダ"(w152) -> ()
                          }
                        }
                      }
                    }
                  }
                  frame #2 {
                    # "測定モード設定時の動作"
                    n114 = local read "設定クラスタ_設定1"() -> (w317:T2)
                    n115 = for {
                      N: 1 -> [_]
                      tunnel: w317 -> [w324]
                      n116 = Unbundle By Name(w324) -> ("測定モード"=w323:u16)
                      n117 = case shown="1" w323 {
                        tunnel: [w325 w335 w345] -> w322
                        frame 1 {
                          # "連続測定モードの場合MAXとMINを表示する"
                          n118 = local read "設定クラスタ_設定1"() -> (w327:T2)
                          n119 = for {
                            N: 1 -> [_]
                            tunnel: w327 -> [w334]
                            tunnel: [w328] -> w325
                            w331 = ""
                            n120 = Bundle By Name(cluster=w334, "実測値MAX"="MAX", "実測値MIN"="MIN", "実測値(MAX)"=w331, "実測値(MIN)"=w331) -> (w328:T2)
                            n121 = property on="実測値(MIN)" class="Str"("DisabledEnum"=T8."Enabled" ("無効")) -> ()  [unwired: 2 in, 2 out]
                            n122 = property on="実測値MIN" class="Str"("DisabledEnum"=T8."Enabled" ("無効")) -> ()  [unwired: 2 in, 2 out]
                          }
                        }
                        frame 2 {
                          # "多点測定モードの場合MAXとMINを表示する"
                          n123 = local read "設定クラスタ_設定1"() -> (w337:T2)
                          n124 = for {
                            N: 1 -> [_]
                            tunnel: w337 -> [w344]
                            tunnel: [w338] -> w335
                            w341 = ""
                            n125 = Bundle By Name(cluster=w344, "実測値MAX"="MAX", "実測値MIN"="MIN", "実測値(MAX)"=w341, "実測値(MIN)"=w341) -> (w338:T2)
                            n126 = property on="実測値(MIN)" class="Str"("DisabledEnum"=T8."Enabled" ("無効")) -> ()  [unwired: 2 in, 2 out]
                            n127 = property on="実測値MIN" class="Str"("DisabledEnum"=T8."Enabled" ("無効")) -> ()  [unwired: 2 in, 2 out]
                          }
                        }
                        frame 0, Default {
                          n128 = local read "設定クラスタ_設定1"() -> (w347:T2)
                          n129 = for {
                            N: 1 -> [_]
                            tunnel: w347 -> [w355]
                            tunnel: [w348] -> w345
                            n130 = Bundle By Name(cluster=w355, "実測値(MAX)"="", "実測値MAX"="値", "実測値(MIN)"="", "実測値MIN"="") -> (w348:T2)
                            n131 = property on="実測値(MIN)" class="Str"("DisabledEnum"=T8."Disabled and Grayed Out" ("無効")) -> ()  [unwired: 2 in, 2 out]
                            n132 = property on="実測値MIN" class="Str"("DisabledEnum"=T8."Disabled and Grayed Out" ("無効")) -> ()  [unwired: 2 in, 2 out]
                          }
                        }
                      }
                      n133 = local write "設定クラスタ_設定1"(w322) -> ()
                    }
                    n134 = property on="品番・品名クラスタ_設定" class="Clust (指定)"() -> ("Value"=w318:T3)  [unwired: 2 in, 2 out]
                    n135 = property on="品番・品名クラスタ_設定 _表示器" class="Clust (指定)"("Value"=w318) -> ()  [unwired: 2 in, 2 out]
                  }
                }
                n136 = Replace Array Subset(array=w52, new element=w47, index=0) -> (w53:T2[])
              }
            }
            frame 1 {
              # "⑯"
              # "⑪"
              n137 = flat-sequence {
                tunnel: w365 -> [w381]
                tunnel: w364 -> [w382]
                tunnel: [w367] -> w359
                tunnel: [w368] -> w358
                tunnel: [w532] -> w363
                tunnel: [w531] -> w362
                tunnel: [w530] -> w357
                tunnel: w359 -> [w531]
                tunnel: w358 -> [w532]
                frame #0 {
                  w366 = "設定2"
                  # "⑧"
                  # "⑦"
                  # "⑬"
                  # "⑫"
                  # "⑥"
                  # "⑤"
                  # "②"
                  # "①"
                  # "複製した時に変更する項目\n①②③④⑤⑥⑦⑧⑨⑩\nローカル変数\n⑪\n指標値\n⑫⑬\nセレクション\n⑭⑮\nプロパティノード設定直し\n⑯\n複製したケースのTrue定数を削除"
                  # "setting.iniファイルからの設定項目の読み取り"
                  n138 = local read "No設定クラスタ_設定 2"() -> (w384:T7)
                  n139 = call-poly <vilib>:"Read Key.vi"("section"="No2.", "error in (no error)"=w381, "key"="No.", "refnum"=w382) -> ("error out"=w388:errorcluster, "value"=w380:i32, "refnum out"=w390:T9)  [unwired: 4 in, 1 out]
                  n140 = Bundle By Name(cluster=w384, "No."=w380) -> (w383:T7)
                  n141 = local write "No設定クラスタ_設定 2"(w383) -> ()
                  n142 = for {
                    shift-right: [w398] -> w389
                    shift-left: w390 -> [w399]
                    shift-right: [w395] -> w387
                    shift-left: w388 -> [w396]
                    tunnel: string[] ["規格", "規格上限", "規格下限", "ポートNo.", "測定モード", "規格単位", "品質チェック項目", "測定周期", "実測MAX", "実測MIN", "実測(MAX)", "実測(MIN)", "測定画面表示ボタン", "ゲージポートNo."] -> [w394] mode=indexing
                    tunnel: w366 -> [w393]
                    i -> [w397]
                    # "④"
                    # "③"
                    n143 = local read "設定クラスタ_設定 2"() -> (w392:T2)
                    n144 = case shown="0, デフォルト" w397 {
                      tunnel: w399 -> [w408 w417 w426 w435 w444 w453 w462 w471 w480 w489 w498 w507 w516 w525]
                      tunnel: [w407 w416 w425 w434 w443 w452 w461 w470 w479 w488 w497 w506 w515 w524] -> w398
                      tunnel: w393 -> [w406 w415 w424 w433 w442 w451 w460 w469 w478 w487 w496 w505 w514 w523]
                      tunnel: w396 -> [w405 w414 w423 w432 w441 w450 w459 w468 w477 w486 w495 w504 w513 w522]
                      tunnel: [w404 w413 w422 w431 w440 w449 w458 w467 w476 w485 w494 w503 w512 w521] -> w395
                      tunnel: w394 -> [w402 w411 w420 w429 w438 w447 w456 w465 w474 w483 w492 w501 w510 w519]
                      tunnel: [w401 w409 w418 w427 w436 w445 w454 w463 w472 w481 w490 w499 w508 w517] -> w391
                      tunnel: w392 -> [w400 w410 w419 w428 w437 w446 w455 w464 w473 w482 w491 w500 w509 w518]
                      frame 0, Default {
                        n145 = call-poly <vilib>:"Read Key.vi"("section"=w406, "error in (no error)"=w405, "key"=w402, "refnum"=w408) -> ("error out"=w404:errorcluster, "value"=w403:string, "refnum out"=w407:T9)  [unwired: 4 in, 1 out]
                        n146 = Bundle By Name(cluster=w400, "規格"=w403) -> (w401:T2)
                      }
                      frame 1 {
                        n147 = call-poly <vilib>:"Read Key.vi"("section"=w415, "error in (no error)"=w414, "key"=w411, "refnum"=w417) -> ("error out"=w413:errorcluster, "value"=w412:string, "refnum out"=w416:T9)  [unwired: 4 in, 1 out]
                        n148 = Bundle By Name(cluster=w410, "規格上限"=w412) -> (w409:T2)
                      }
                      frame 2 {
                        n149 = call-poly <vilib>:"Read Key.vi"("section"=w424, "error in (no error)"=w423, "key"=w420, "refnum"=w426) -> ("error out"=w422:errorcluster, "value"=w421:string, "refnum out"=w425:T9)  [unwired: 4 in, 1 out]
                        n150 = Bundle By Name(cluster=w419, "規格下限"=w421) -> (w418:T2)
                      }
                      frame 3 {
                        n151 = call-poly <vilib>:"Read Key.vi"("section"=w433, "error in (no error)"=w432, "key"=w429, "refnum"=w435) -> ("error out"=w431:errorcluster, "value"=w430:i32, "refnum out"=w434:T9)  [unwired: 4 in, 1 out]
                        n152 = Bundle By Name(cluster=w428, "ポートNo."=w430) -> (w427:T2)
                      }
                      frame 4 {
                        n153 = call-poly <vilib>:"Read Key.vi"("section"=w442, "error in (no error)"=w441, "key"=w438, "refnum"=w444) -> ("error out"=w440:errorcluster, "value"=w439:i32, "refnum out"=w443:T9)  [unwired: 4 in, 1 out]
                        n154 = Bundle By Name(cluster=w437, "測定モード"=w439) -> (w436:T2)
                      }
                      frame 5 {
                        n155 = call-poly <vilib>:"Read Key.vi"("section"=w451, "error in (no error)"=w450, "key"=w447, "refnum"=w453) -> ("error out"=w449:errorcluster, "value"=w448:string, "refnum out"=w452:T9)  [unwired: 4 in, 1 out]
                        n156 = Bundle By Name(cluster=w446, "規格単位"=w448) -> (w445:T2)
                      }
                      frame 6 {
                        n157 = call-poly <vilib>:"Read Key.vi"("section"=w460, "error in (no error)"=w459, "key"=w456, "refnum"=w462) -> ("error out"=w458:errorcluster, "value"=w457:string, "refnum out"=w461:T9)  [unwired: 4 in, 1 out]
                        n158 = Bundle By Name(cluster=w455, "品質チェック項目"=w457) -> (w454:T2)
                      }
                      frame 7 {
                        n159 = call-poly <vilib>:"Read Key.vi"("section"=w469, "error in (no error)"=w468, "key"=w465, "refnum"=w471) -> ("error out"=w467:errorcluster, "value"=w466:i32, "refnum out"=w470:T9)  [unwired: 4 in, 1 out]
                        n160 = Bundle By Name(cluster=w464, "測定周期"=w466) -> (w463:T2)
                      }
                      frame 8 {
                        n161 = call-poly <vilib>:"Read Key.vi"("section"=w478, "error in (no error)"=w477, "key"=w474, "refnum"=w480) -> ("error out"=w476:errorcluster, "value"=w475:string, "refnum out"=w479:T9)  [unwired: 4 in, 1 out]
                        n162 = Bundle By Name(cluster=w473, "実測値MAX"=w475) -> (w472:T2)
                      }
                      frame 9 {
                        n163 = call-poly <vilib>:"Read Key.vi"("section"=w487, "error in (no error)"=w486, "key"=w483, "refnum"=w489) -> ("error out"=w485:errorcluster, "value"=w484:string, "refnum out"=w488:T9)  [unwired: 4 in, 1 out]
                        n164 = Bundle By Name(cluster=w482, "実測値MIN"=w484) -> (w481:T2)
                      }
                      frame 10 {
                        n165 = call-poly <vilib>:"Read Key.vi"("section"=w496, "error in (no error)"=w495, "key"=w492, "refnum"=w498) -> ("error out"=w494:errorcluster, "value"=w493:string, "refnum out"=w497:T9)  [unwired: 4 in, 1 out]
                        n166 = Bundle By Name(cluster=w491, "実測値(MAX)"=w493) -> (w490:T2)
                      }
                      frame 11 {
                        n167 = call-poly <vilib>:"Read Key.vi"("section"=w505, "error in (no error)"=w504, "key"=w501, "refnum"=w507) -> ("error out"=w503:errorcluster, "value"=w502:string, "refnum out"=w506:T9)  [unwired: 4 in, 1 out]
                        n168 = Bundle By Name(cluster=w500, "実測値(MIN)"=w502) -> (w499:T2)
                      }
                      frame 12 {
                        n169 = call-poly <vilib>:"Read Key.vi"("section"=w514, "error in (no error)"=w513, "key"=w510, "refnum"=w516) -> ("error out"=w512:errorcluster, "value"=w511:bool, "refnum out"=w515:T9)  [unwired: 4 in, 1 out]
                        n170 = Bundle By Name(cluster=w509, "測定画面表示ボタン"=w511) -> (w508:T2)
                      }
                      frame 13 {
                        n171 = call-poly <vilib>:"Read Key.vi"("section"=w523, "error in (no error)"=w522, "key"=w519, "refnum"=w525) -> ("error out"=w521:errorcluster, "value"=w520:string, "refnum out"=w524:T9)  [unwired: 4 in, 1 out]
                        n172 = Bundle By Name(cluster=w518, "ゲージポートNo"=w520) -> (w517:T2)
                      }
                    }
                    n173 = local write "設定クラスタ_設定 2"(w391) -> ()
                  }
                  n174 = local read "使用ON/OFFボタン_設定 2"() -> (w376:T5)
                  n175 = call-poly <vilib>:"Read Key.vi"("section"=w366, "error in (no error)"=w387, "key"="使用ON/OFF", "refnum"=w389) -> ("error out"=w369:errorcluster, "value"=w378:bool, "refnum out"=w370:T9)  [unwired: 4 in, 1 out]
                  n176 = Bundle By Name(cluster=w376, "使用ON/OFF"=w378) -> (w375:T5)
                  n177 = local write "使用ON/OFFボタン_設定 2"(w375) -> ()
                  n178 = local read "CSV項目名 2"() -> (w373:T1)
                  n179 = call-poly <vilib>:"Read Key.vi"("section"=w366, "error in (no error)"=w369, "key"="CSVヘッダー名", "refnum"=w370) -> ("error out"=w368:errorcluster, "value"=w371:string, "refnum out"=w367:T9)  [unwired: 4 in, 1 out]
                  n180 = Bundle By Name(cluster=w373, "CSV項目名"=w371) -> (w374:T1)
                  n181 = local write "CSV項目名 2"(w374) -> ()
                }
                frame #1 {
                  # "⑮"
                  # "⑭"
                  # "⑩"
                  # "⑨"
                  # "測定モード設定時の動作"
                  n182 = local read "設定クラスタ_設定 2"() -> (w530:T2)
                  n183 = Unbundle By Name(w530) -> ("測定モード"=w529:u16)
                  n184 = case shown="0, デフォルト" w529 {
                    tunnel: w530 -> [w539 w546 w554]
                    tunnel: [w538 w545 w553] -> w528
                    tunnel: [T8."Enabled" ("無効") T8."Enabled" ("無効") T8."Disabled and Grayed Out" ("無効")] -> w527
                    tunnel: [T8."Enabled" ("無効") T8."Enabled" ("無効") T8."Disabled and Grayed Out" ("無効")] -> w526
                    frame 1 {
                      w535 = ""
                      # "連続測定モードの場合MAXとMINを表示する"
                      n185 = Bundle By Name(cluster=w539, "実測値MAX"="MAX", "実測値MIN"="MIN", "実測値(MAX)"=w535, "実測値(MIN)"=w535) -> (w538:T2)
                    }
                    frame 2 {
                      w542 = ""
                      # "多点測定モードの場合MAXとMINを表示する"
                      n186 = Bundle By Name(cluster=w546, "実測値MAX"="MAX", "実測値MIN"="MIN", "実測値(MAX)"=w542, "実測値(MIN)"=w542) -> (w545:T2)
                    }
                    frame 0, Default {
                      n187 = Bundle By Name(cluster=w554, "実測値(MAX)"="", "実測値MAX"="値", "実測値(MIN)"="", "実測値MIN"="") -> (w553:T2)
                    }
                  }
                  n188 = local write "設定クラスタ_設定 2"(w528) -> ()
                  n189 = property on="実測値MIN" class="Str"("DisabledEnum"=w527) -> ()  [unwired: 2 in, 2 out]
                  n190 = property on="実測値(MIN)" class="Str"("DisabledEnum"=w526) -> ()  [unwired: 2 in, 2 out]
                }
              }
              n191 = Replace Array Subset(array=w360, new element=w357, index=1) -> (w361:T2[])
            }
            frame 2 {
              # "⑯"
              # "⑪"
              n192 = flat-sequence {
                tunnel: w564 -> [w580]
                tunnel: w563 -> [w581]
                tunnel: [w566] -> w558
                tunnel: [w567] -> w557
                tunnel: [w731] -> w562
                tunnel: [w730] -> w561
                tunnel: [w729] -> w556
                tunnel: w558 -> [w730]
                tunnel: w557 -> [w731]
                frame #0 {
                  w565 = "設定3"
                  # "⑧"
                  # "⑦"
                  # "⑬"
                  # "⑫"
                  # "⑥"
                  # "⑤"
                  # "②"
                  # "①"
                  # "複製した時に変更する項目\n①②③④⑤⑥⑦⑧⑨⑩\nローカル変数\n⑪\n指標値\n⑫⑬\nセレクション\n⑭⑮\nプロパティノード設定直し\n⑯\n複製したケースのTrue定数を削除"
                  # "setting.iniファイルからの設定項目の読み取り"
                  n193 = local read "No設定クラスタ_設定 3"() -> (w583:T7)
                  n194 = call-poly <vilib>:"Read Key.vi"("section"="No3.", "error in (no error)"=w580, "key"="No.", "refnum"=w581) -> ("error out"=w587:errorcluster, "value"=w579:i32, "refnum out"=w589:T9)  [unwired: 4 in, 1 out]
                  n195 = Bundle By Name(cluster=w583, "No."=w579) -> (w582:T7)
                  n196 = local write "No設定クラスタ_設定 3"(w582) -> ()
                  n197 = for {
                    shift-right: [w597] -> w588
                    shift-left: w589 -> [w598]
                    shift-right: [w594] -> w586
                    shift-left: w587 -> [w595]
                    tunnel: string[] ["規格", "規格上限", "規格下限", "ポートNo.", "測定モード", "規格単位", "品質チェック項目", "測定周期", "実測MAX", "実測MIN", "実測(MAX)", "実測(MIN)", "測定画面表示ボタン", "ゲージポートNo."] -> [w593] mode=indexing
                    tunnel: w565 -> [w592]
                    i -> [w596]
                    # "④"
                    # "③"
                    n198 = local read "設定クラスタ_設定 3"() -> (w591:T2)
                    n199 = case shown="0, デフォルト" w596 {
                      tunnel: w598 -> [w607 w616 w625 w634 w643 w652 w661 w670 w679 w688 w697 w706 w715 w724]
                      tunnel: [w606 w615 w624 w633 w642 w651 w660 w669 w678 w687 w696 w705 w714 w723] -> w597
                      tunnel: w592 -> [w605 w614 w623 w632 w641 w650 w659 w668 w677 w686 w695 w704 w713 w722]
                      tunnel: w595 -> [w604 w613 w622 w631 w640 w649 w658 w667 w676 w685 w694 w703 w712 w721]
                      tunnel: [w603 w612 w621 w630 w639 w648 w657 w666 w675 w684 w693 w702 w711 w720] -> w594
                      tunnel: w593 -> [w601 w610 w619 w628 w637 w646 w655 w664 w673 w682 w691 w700 w709 w718]
                      tunnel: [w600 w608 w617 w626 w635 w644 w653 w662 w671 w680 w689 w698 w707 w716] -> w590
                      tunnel: w591 -> [w599 w609 w618 w627 w636 w645 w654 w663 w672 w681 w690 w699 w708 w717]
                      frame 0, Default {
                        n200 = call-poly <vilib>:"Read Key.vi"("section"=w605, "error in (no error)"=w604, "key"=w601, "refnum"=w607) -> ("error out"=w603:errorcluster, "value"=w602:string, "refnum out"=w606:T9)  [unwired: 4 in, 1 out]
                        n201 = Bundle By Name(cluster=w599, "規格"=w602) -> (w600:T2)
                      }
                      frame 1 {
                        n202 = call-poly <vilib>:"Read Key.vi"("section"=w614, "error in (no error)"=w613, "key"=w610, "refnum"=w616) -> ("error out"=w612:errorcluster, "value"=w611:string, "refnum out"=w615:T9)  [unwired: 4 in, 1 out]
                        n203 = Bundle By Name(cluster=w609, "規格上限"=w611) -> (w608:T2)
                      }
                      frame 2 {
                        n204 = call-poly <vilib>:"Read Key.vi"("section"=w623, "error in (no error)"=w622, "key"=w619, "refnum"=w625) -> ("error out"=w621:errorcluster, "value"=w620:string, "refnum out"=w624:T9)  [unwired: 4 in, 1 out]
                        n205 = Bundle By Name(cluster=w618, "規格下限"=w620) -> (w617:T2)
                      }
                      frame 3 {
                        n206 = call-poly <vilib>:"Read Key.vi"("section"=w632, "error in (no error)"=w631, "key"=w628, "refnum"=w634) -> ("error out"=w630:errorcluster, "value"=w629:i32, "refnum out"=w633:T9)  [unwired: 4 in, 1 out]
                        n207 = Bundle By Name(cluster=w627, "ポートNo."=w629) -> (w626:T2)
                      }
                      frame 4 {
                        n208 = call-poly <vilib>:"Read Key.vi"("section"=w641, "error in (no error)"=w640, "key"=w637, "refnum"=w643) -> ("error out"=w639:errorcluster, "value"=w638:i32, "refnum out"=w642:T9)  [unwired: 4 in, 1 out]
                        n209 = Bundle By Name(cluster=w636, "測定モード"=w638) -> (w635:T2)
                      }
                      frame 5 {
                        n210 = call-poly <vilib>:"Read Key.vi"("section"=w650, "error in (no error)"=w649, "key"=w646, "refnum"=w652) -> ("error out"=w648:errorcluster, "value"=w647:string, "refnum out"=w651:T9)  [unwired: 4 in, 1 out]
                        n211 = Bundle By Name(cluster=w645, "規格単位"=w647) -> (w644:T2)
                      }
                      frame 6 {
                        n212 = call-poly <vilib>:"Read Key.vi"("section"=w659, "error in (no error)"=w658, "key"=w655, "refnum"=w661) -> ("error out"=w657:errorcluster, "value"=w656:string, "refnum out"=w660:T9)  [unwired: 4 in, 1 out]
                        n213 = Bundle By Name(cluster=w654, "品質チェック項目"=w656) -> (w653:T2)
                      }
                      frame 7 {
                        n214 = call-poly <vilib>:"Read Key.vi"("section"=w668, "error in (no error)"=w667, "key"=w664, "refnum"=w670) -> ("error out"=w666:errorcluster, "value"=w665:i32, "refnum out"=w669:T9)  [unwired: 4 in, 1 out]
                        n215 = Bundle By Name(cluster=w663, "測定周期"=w665) -> (w662:T2)
                      }
                      frame 8 {
                        n216 = call-poly <vilib>:"Read Key.vi"("section"=w677, "error in (no error)"=w676, "key"=w673, "refnum"=w679) -> ("error out"=w675:errorcluster, "value"=w674:string, "refnum out"=w678:T9)  [unwired: 4 in, 1 out]
                        n217 = Bundle By Name(cluster=w672, "実測値MAX"=w674) -> (w671:T2)
                      }
                      frame 9 {
                        n218 = call-poly <vilib>:"Read Key.vi"("section"=w686, "error in (no error)"=w685, "key"=w682, "refnum"=w688) -> ("error out"=w684:errorcluster, "value"=w683:string, "refnum out"=w687:T9)  [unwired: 4 in, 1 out]
                        n219 = Bundle By Name(cluster=w681, "実測値MIN"=w683) -> (w680:T2)
                      }
                      frame 10 {
                        n220 = call-poly <vilib>:"Read Key.vi"("section"=w695, "error in (no error)"=w694, "key"=w691, "refnum"=w697) -> ("error out"=w693:errorcluster, "value"=w692:string, "refnum out"=w696:T9)  [unwired: 4 in, 1 out]
                        n221 = Bundle By Name(cluster=w690, "実測値(MAX)"=w692) -> (w689:T2)
                      }
                      frame 11 {
                        n222 = call-poly <vilib>:"Read Key.vi"("section"=w704, "error in (no error)"=w703, "key"=w700, "refnum"=w706) -> ("error out"=w702:errorcluster, "value"=w701:string, "refnum out"=w705:T9)  [unwired: 4 in, 1 out]
                        n223 = Bundle By Name(cluster=w699, "実測値(MIN)"=w701) -> (w698:T2)
                      }
                      frame 12 {
                        n224 = call-poly <vilib>:"Read Key.vi"("section"=w713, "error in (no error)"=w712, "key"=w709, "refnum"=w715) -> ("error out"=w711:errorcluster, "value"=w710:bool, "refnum out"=w714:T9)  [unwired: 4 in, 1 out]
                        n225 = Bundle By Name(cluster=w708, "測定画面表示ボタン"=w710) -> (w707:T2)
                      }
                      frame 13 {
                        n226 = call-poly <vilib>:"Read Key.vi"("section"=w722, "error in (no error)"=w721, "key"=w718, "refnum"=w724) -> ("error out"=w720:errorcluster, "value"=w719:string, "refnum out"=w723:T9)  [unwired: 4 in, 1 out]
                        n227 = Bundle By Name(cluster=w717, "ゲージポートNo"=w719) -> (w716:T2)
                      }
                    }
                    n228 = local write "設定クラスタ_設定 3"(w590) -> ()
                  }
                  n229 = local read "使用ON/OFFボタン_設定 3"() -> (w575:T5)
                  n230 = call-poly <vilib>:"Read Key.vi"("section"=w565, "error in (no error)"=w586, "key"="使用ON/OFF", "refnum"=w588) -> ("error out"=w568:errorcluster, "value"=w577:bool, "refnum out"=w569:T9)  [unwired: 4 in, 1 out]
                  n231 = Bundle By Name(cluster=w575, "使用ON/OFF"=w577) -> (w574:T5)
                  n232 = local write "使用ON/OFFボタン_設定 3"(w574) -> ()
                  n233 = local read "CSV項目名 3"() -> (w572:T1)
                  n234 = call-poly <vilib>:"Read Key.vi"("section"=w565, "error in (no error)"=w568, "key"="CSVヘッダー名", "refnum"=w569) -> ("error out"=w567:errorcluster, "value"=w570:string, "refnum out"=w566:T9)  [unwired: 4 in, 1 out]
                  n235 = Bundle By Name(cluster=w572, "CSV項目名"=w570) -> (w573:T1)
                  n236 = local write "CSV項目名 3"(w573) -> ()
                }
                frame #1 {
                  # "⑮"
                  # "⑭"
                  # "⑩"
                  # "⑨"
                  # "測定モード設定時の動作"
                  n237 = local read "設定クラスタ_設定 3"() -> (w729:T2)
                  n238 = Unbundle By Name(w729) -> ("測定モード"=w728:u16)
                  n239 = case shown="0, デフォルト" w728 {
                    tunnel: w729 -> [w738 w745 w753]
                    tunnel: [w737 w744 w752] -> w727
                    tunnel: [T8."Enabled" ("無効") T8."Enabled" ("無効") T8."Disabled and Grayed Out" ("無効")] -> w726
                    tunnel: [T8."Enabled" ("無効") T8."Enabled" ("無効") T8."Disabled and Grayed Out" ("無効")] -> w725
                    frame 1 {
                      w734 = ""
                      # "連続測定モードの場合MAXとMINを表示する"
                      n240 = Bundle By Name(cluster=w738, "実測値MAX"="MAX", "実測値MIN"="MIN", "実測値(MAX)"=w734, "実測値(MIN)"=w734) -> (w737:T2)
                    }
                    frame 2 {
                      w741 = ""
                      # "多点測定モードの場合MAXとMINを表示する"
                      n241 = Bundle By Name(cluster=w745, "実測値MAX"="MAX", "実測値MIN"="MIN", "実測値(MAX)"=w741, "実測値(MIN)"=w741) -> (w744:T2)
                    }
                    frame 0, Default {
                      n242 = Bundle By Name(cluster=w753, "実測値(MAX)"="", "実測値MAX"="値", "実測値(MIN)"="", "実測値MIN"="") -> (w752:T2)
                    }
                  }
                  n243 = local write "設定クラスタ_設定 3"(w727) -> ()
                  n244 = property on="実測値MIN" class="Str"("DisabledEnum"=w726) -> ()  [unwired: 2 in, 2 out]
                  n245 = property on="実測値(MIN)" class="Str"("DisabledEnum"=w725) -> ()  [unwired: 2 in, 2 out]
                }
              }
              n246 = Replace Array Subset(array=w559, new element=w556, index=2) -> (w560:T2[])
            }
            frame 3 {
              # "⑯"
              # "⑪"
              n247 = flat-sequence {
                tunnel: w763 -> [w779]
                tunnel: w762 -> [w780]
                tunnel: [w765] -> w757
                tunnel: [w766] -> w756
                tunnel: [w930] -> w761
                tunnel: [w929] -> w760
                tunnel: [w928] -> w755
                tunnel: w757 -> [w929]
                tunnel: w756 -> [w930]
                frame #0 {
                  w764 = "設定4"
                  # "⑧"
                  # "⑦"
                  # "⑬"
                  # "⑫"
                  # "⑥"
                  # "⑤"
                  # "②"
                  # "①"
                  # "複製した時に変更する項目\n①②③④⑤⑥⑦⑧⑨⑩\nローカル変数\n⑪\n指標値\n⑫⑬\nセレクション\n⑭⑮\nプロパティノード設定直し\n⑯\n複製したケースのTrue定数を削除"
                  # "setting.iniファイルからの設定項目の読み取り"
                  n248 = local read "No設定クラスタ_設定 4"() -> (w782:T7)
                  n249 = call-poly <vilib>:"Read Key.vi"("section"="No4.", "error in (no error)"=w779, "key"="No.", "refnum"=w780) -> ("error out"=w786:errorcluster, "value"=w778:i32, "refnum out"=w788:T9)  [unwired: 4 in, 1 out]
                  n250 = Bundle By Name(cluster=w782, "No."=w778) -> (w781:T7)
                  n251 = local write "No設定クラスタ_設定 4"(w781) -> ()
                  n252 = for {
                    shift-right: [w796] -> w787
                    shift-left: w788 -> [w797]
                    shift-right: [w793] -> w785
                    shift-left: w786 -> [w794]
                    tunnel: string[] ["規格", "規格上限", "規格下限", "ポートNo.", "測定モード", "規格単位", "品質チェック項目", "測定周期", "実測MAX", "実測MIN", "実測(MAX)", "実測(MIN)", "測定画面表示ボタン", "ゲージポートNo."] -> [w792] mode=indexing
                    tunnel: w764 -> [w791]
                    i -> [w795]
                    # "④"
                    # "③"
                    n253 = local read "設定クラスタ_設定 4"() -> (w790:T2)
                    n254 = case shown="0, デフォルト" w795 {
                      tunnel: w797 -> [w806 w815 w824 w833 w842 w851 w860 w869 w878 w887 w896 w905 w914 w923]
                      tunnel: [w805 w814 w823 w832 w841 w850 w859 w868 w877 w886 w895 w904 w913 w922] -> w796
                      tunnel: w791 -> [w804 w813 w822 w831 w840 w849 w858 w867 w876 w885 w894 w903 w912 w921]
                      tunnel: w794 -> [w803 w812 w821 w830 w839 w848 w857 w866 w875 w884 w893 w902 w911 w920]
                      tunnel: [w802 w811 w820 w829 w838 w847 w856 w865 w874 w883 w892 w901 w910 w919] -> w793
                      tunnel: w792 -> [w800 w809 w818 w827 w836 w845 w854 w863 w872 w881 w890 w899 w908 w917]
                      tunnel: [w799 w807 w816 w825 w834 w843 w852 w861 w870 w879 w888 w897 w906 w915] -> w789
                      tunnel: w790 -> [w798 w808 w817 w826 w835 w844 w853 w862 w871 w880 w889 w898 w907 w916]
                      frame 0, Default {
                        n255 = call-poly <vilib>:"Read Key.vi"("section"=w804, "error in (no error)"=w803, "key"=w800, "refnum"=w806) -> ("error out"=w802:errorcluster, "value"=w801:string, "refnum out"=w805:T9)  [unwired: 4 in, 1 out]
                        n256 = Bundle By Name(cluster=w798, "規格"=w801) -> (w799:T2)
                      }
                      frame 1 {
                        n257 = call-poly <vilib>:"Read Key.vi"("section"=w813, "error in (no error)"=w812, "key"=w809, "refnum"=w815) -> ("error out"=w811:errorcluster, "value"=w810:string, "refnum out"=w814:T9)  [unwired: 4 in, 1 out]
                        n258 = Bundle By Name(cluster=w808, "規格上限"=w810) -> (w807:T2)
                      }
                      frame 2 {
                        n259 = call-poly <vilib>:"Read Key.vi"("section"=w822, "error in (no error)"=w821, "key"=w818, "refnum"=w824) -> ("error out"=w820:errorcluster, "value"=w819:string, "refnum out"=w823:T9)  [unwired: 4 in, 1 out]
                        n260 = Bundle By Name(cluster=w817, "規格下限"=w819) -> (w816:T2)
                      }
                      frame 3 {
                        n261 = call-poly <vilib>:"Read Key.vi"("section"=w831, "error in (no error)"=w830, "key"=w827, "refnum"=w833) -> ("error out"=w829:errorcluster, "value"=w828:i32, "refnum out"=w832:T9)  [unwired: 4 in, 1 out]
                        n262 = Bundle By Name(cluster=w826, "ポートNo."=w828) -> (w825:T2)
                      }
                      frame 4 {
                        n263 = call-poly <vilib>:"Read Key.vi"("section"=w840, "error in (no error)"=w839, "key"=w836, "refnum"=w842) -> ("error out"=w838:errorcluster, "value"=w837:i32, "refnum out"=w841:T9)  [unwired: 4 in, 1 out]
                        n264 = Bundle By Name(cluster=w835, "測定モード"=w837) -> (w834:T2)
                      }
                      frame 5 {
                        n265 = call-poly <vilib>:"Read Key.vi"("section"=w849, "error in (no error)"=w848, "key"=w845, "refnum"=w851) -> ("error out"=w847:errorcluster, "value"=w846:string, "refnum out"=w850:T9)  [unwired: 4 in, 1 out]
                        n266 = Bundle By Name(cluster=w844, "規格単位"=w846) -> (w843:T2)
                      }
                      frame 6 {
                        n267 = call-poly <vilib>:"Read Key.vi"("section"=w858, "error in (no error)"=w857, "key"=w854, "refnum"=w860) -> ("error out"=w856:errorcluster, "value"=w855:string, "refnum out"=w859:T9)  [unwired: 4 in, 1 out]
                        n268 = Bundle By Name(cluster=w853, "品質チェック項目"=w855) -> (w852:T2)
                      }
                      frame 7 {
                        n269 = call-poly <vilib>:"Read Key.vi"("section"=w867, "error in (no error)"=w866, "key"=w863, "refnum"=w869) -> ("error out"=w865:errorcluster, "value"=w864:i32, "refnum out"=w868:T9)  [unwired: 4 in, 1 out]
                        n270 = Bundle By Name(cluster=w862, "測定周期"=w864) -> (w861:T2)
                      }
                      frame 8 {
                        n271 = call-poly <vilib>:"Read Key.vi"("section"=w876, "error in (no error)"=w875, "key"=w872, "refnum"=w878) -> ("error out"=w874:errorcluster, "value"=w873:string, "refnum out"=w877:T9)  [unwired: 4 in, 1 out]
                        n272 = Bundle By Name(cluster=w871, "実測値MAX"=w873) -> (w870:T2)
                      }
                      frame 9 {
                        n273 = call-poly <vilib>:"Read Key.vi"("section"=w885, "error in (no error)"=w884, "key"=w881, "refnum"=w887) -> ("error out"=w883:errorcluster, "value"=w882:string, "refnum out"=w886:T9)  [unwired: 4 in, 1 out]
                        n274 = Bundle By Name(cluster=w880, "実測値MIN"=w882) -> (w879:T2)
                      }
                      frame 10 {
                        n275 = call-poly <vilib>:"Read Key.vi"("section"=w894, "error in (no error)"=w893, "key"=w890, "refnum"=w896) -> ("error out"=w892:errorcluster, "value"=w891:string, "refnum out"=w895:T9)  [unwired: 4 in, 1 out]
                        n276 = Bundle By Name(cluster=w889, "実測値(MAX)"=w891) -> (w888:T2)
                      }
                      frame 11 {
                        n277 = call-poly <vilib>:"Read Key.vi"("section"=w903, "error in (no error)"=w902, "key"=w899, "refnum"=w905) -> ("error out"=w901:errorcluster, "value"=w900:string, "refnum out"=w904:T9)  [unwired: 4 in, 1 out]
                        n278 = Bundle By Name(cluster=w898, "実測値(MIN)"=w900) -> (w897:T2)
                      }
                      frame 12 {
                        n279 = call-poly <vilib>:"Read Key.vi"("section"=w912, "error in (no error)"=w911, "key"=w908, "refnum"=w914) -> ("error out"=w910:errorcluster, "value"=w909:bool, "refnum out"=w913:T9)  [unwired: 4 in, 1 out]
                        n280 = Bundle By Name(cluster=w907, "測定画面表示ボタン"=w909) -> (w906:T2)
                      }
                      frame 13 {
                        n281 = call-poly <vilib>:"Read Key.vi"("section"=w921, "error in (no error)"=w920, "key"=w917, "refnum"=w923) -> ("error out"=w919:errorcluster, "value"=w918:string, "refnum out"=w922:T9)  [unwired: 4 in, 1 out]
                        n282 = Bundle By Name(cluster=w916, "ゲージポートNo"=w918) -> (w915:T2)
                      }
                    }
                    n283 = local write "設定クラスタ_設定 4"(w789) -> ()
                  }
                  n284 = local read "使用ON/OFFボタン_設定 4"() -> (w774:T5)
                  n285 = call-poly <vilib>:"Read Key.vi"("section"=w764, "error in (no error)"=w785, "key"="使用ON/OFF", "refnum"=w787) -> ("error out"=w767:errorcluster, "value"=w776:bool, "refnum out"=w768:T9)  [unwired: 4 in, 1 out]
                  n286 = Bundle By Name(cluster=w774, "使用ON/OFF"=w776) -> (w773:T5)
                  n287 = local write "使用ON/OFFボタン_設定 4"(w773) -> ()
                  n288 = local read "CSV項目名 4"() -> (w771:T1)
                  n289 = call-poly <vilib>:"Read Key.vi"("section"=w764, "error in (no error)"=w767, "key"="CSVヘッダー名", "refnum"=w768) -> ("error out"=w766:errorcluster, "value"=w769:string, "refnum out"=w765:T9)  [unwired: 4 in, 1 out]
                  n290 = Bundle By Name(cluster=w771, "CSV項目名"=w769) -> (w772:T1)
                  n291 = local write "CSV項目名 4"(w772) -> ()
                }
                frame #1 {
                  # "⑮"
                  # "⑭"
                  # "⑩"
                  # "⑨"
                  # "測定モード設定時の動作"
                  n292 = local read "設定クラスタ_設定 4"() -> (w928:T2)
                  n293 = Unbundle By Name(w928) -> ("測定モード"=w927:u16)
                  n294 = case shown="0, デフォルト" w927 {
                    tunnel: w928 -> [w937 w944 w952]
                    tunnel: [w936 w943 w951] -> w926
                    tunnel: [T8."Enabled" ("無効") T8."Enabled" ("無効") T8."Disabled and Grayed Out" ("無効")] -> w925
                    tunnel: [T8."Enabled" ("無効") T8."Enabled" ("無効") T8."Disabled and Grayed Out" ("無効")] -> w924
                    frame 1 {
                      w933 = ""
                      # "連続測定モードの場合MAXとMINを表示する"
                      n295 = Bundle By Name(cluster=w937, "実測値MAX"="MAX", "実測値MIN"="MIN", "実測値(MAX)"=w933, "実測値(MIN)"=w933) -> (w936:T2)
                    }
                    frame 2 {
                      w940 = ""
                      # "多点測定モードの場合MAXとMINを表示する"
                      n296 = Bundle By Name(cluster=w944, "実測値MAX"="MAX", "実測値MIN"="MIN", "実測値(MAX)"=w940, "実測値(MIN)"=w940) -> (w943:T2)
                    }
                    frame 0, Default {
                      n297 = Bundle By Name(cluster=w952, "実測値(MAX)"="", "実測値MAX"="値", "実測値(MIN)"="", "実測値MIN"="") -> (w951:T2)
                    }
                  }
                  n298 = local write "設定クラスタ_設定 4"(w926) -> ()
                  n299 = property on="実測値MIN" class="Str"("DisabledEnum"=w925) -> ()  [unwired: 2 in, 2 out]
                  n300 = property on="実測値(MIN)" class="Str"("DisabledEnum"=w924) -> ()  [unwired: 2 in, 2 out]
                }
              }
              n301 = Replace Array Subset(array=w758, new element=w755, index=3) -> (w759:T2[])
            }
            frame 4 {
              # "⑯"
              # "⑪"
              n302 = flat-sequence {
                tunnel: w962 -> [w978]
                tunnel: w961 -> [w979]
                tunnel: [w964] -> w956
                tunnel: [w965] -> w955
                tunnel: [w1129] -> w960
                tunnel: [w1128] -> w959
                tunnel: [w1127] -> w954
                tunnel: w956 -> [w1128]
                tunnel: w955 -> [w1129]
                frame #0 {
                  w963 = "設定5"
                  # "⑧"
                  # "⑦"
                  # "⑬"
                  # "⑫"
                  # "⑥"
                  # "⑤"
                  # "②"
                  # "①"
                  # "複製した時に変更する項目\n①②③④⑤⑥⑦⑧⑨⑩\nローカル変数\n⑪\n指標値\n⑫⑬\nセレクション\n⑭⑮\nプロパティノード設定直し\n⑯\n複製したケースのTrue定数を削除"
                  # "setting.iniファイルからの設定項目の読み取り"
                  n303 = local read "No設定クラスタ_設定 5"() -> (w981:T7)
                  n304 = call-poly <vilib>:"Read Key.vi"("section"="No5.", "error in (no error)"=w978, "key"="No.", "refnum"=w979) -> ("error out"=w985:errorcluster, "value"=w977:i32, "refnum out"=w987:T9)  [unwired: 4 in, 1 out]
                  n305 = Bundle By Name(cluster=w981, "No."=w977) -> (w980:T7)
                  n306 = local write "No設定クラスタ_設定 5"(w980) -> ()
                  n307 = for {
                    shift-right: [w995] -> w986
                    shift-left: w987 -> [w996]
                    shift-right: [w992] -> w984
                    shift-left: w985 -> [w993]
                    tunnel: string[] ["規格", "規格上限", "規格下限", "ポートNo.", "測定モード", "規格単位", "品質チェック項目", "測定周期", "実測MAX", "実測MIN", "実測(MAX)", "実測(MIN)", "測定画面表示ボタン", "ゲージポートNo."] -> [w991] mode=indexing
                    tunnel: w963 -> [w990]
                    i -> [w994]
                    # "④"
                    # "③"
                    n308 = local read "設定クラスタ_設定 5"() -> (w989:T2)
                    n309 = case shown="0, デフォルト" w994 {
                      tunnel: w996 -> [w1005 w1014 w1023 w1032 w1041 w1050 w1059 w1068 w1077 w1086 w1095 w1104 w1113 w1122]
                      tunnel: [w1004 w1013 w1022 w1031 w1040 w1049 w1058 w1067 w1076 w1085 w1094 w1103 w1112 w1121] -> w995
                      tunnel: w990 -> [w1003 w1012 w1021 w1030 w1039 w1048 w1057 w1066 w1075 w1084 w1093 w1102 w1111 w1120]
                      tunnel: w993 -> [w1002 w1011 w1020 w1029 w1038 w1047 w1056 w1065 w1074 w1083 w1092 w1101 w1110 w1119]
                      tunnel: [w1001 w1010 w1019 w1028 w1037 w1046 w1055 w1064 w1073 w1082 w1091 w1100 w1109 w1118] -> w992
                      tunnel: w991 -> [w999 w1008 w1017 w1026 w1035 w1044 w1053 w1062 w1071 w1080 w1089 w1098 w1107 w1116]
                      tunnel: [w998 w1006 w1015 w1024 w1033 w1042 w1051 w1060 w1069 w1078 w1087 w1096 w1105 w1114] -> w988
                      tunnel: w989 -> [w997 w1007 w1016 w1025 w1034 w1043 w1052 w1061 w1070 w1079 w1088 w1097 w1106 w1115]
                      frame 0, Default {
                        n310 = call-poly <vilib>:"Read Key.vi"("section"=w1003, "error in (no error)"=w1002, "key"=w999, "refnum"=w1005) -> ("error out"=w1001:errorcluster, "value"=w1000:string, "refnum out"=w1004:T9)  [unwired: 4 in, 1 out]
                        n311 = Bundle By Name(cluster=w997, "規格"=w1000) -> (w998:T2)
                      }
                      frame 1 {
                        n312 = call-poly <vilib>:"Read Key.vi"("section"=w1012, "error in (no error)"=w1011, "key"=w1008, "refnum"=w1014) -> ("error out"=w1010:errorcluster, "value"=w1009:string, "refnum out"=w1013:T9)  [unwired: 4 in, 1 out]
                        n313 = Bundle By Name(cluster=w1007, "規格上限"=w1009) -> (w1006:T2)
                      }
                      frame 2 {
                        n314 = call-poly <vilib>:"Read Key.vi"("section"=w1021, "error in (no error)"=w1020, "key"=w1017, "refnum"=w1023) -> ("error out"=w1019:errorcluster, "value"=w1018:string, "refnum out"=w1022:T9)  [unwired: 4 in, 1 out]
                        n315 = Bundle By Name(cluster=w1016, "規格下限"=w1018) -> (w1015:T2)
                      }
                      frame 3 {
                        n316 = call-poly <vilib>:"Read Key.vi"("section"=w1030, "error in (no error)"=w1029, "key"=w1026, "refnum"=w1032) -> ("error out"=w1028:errorcluster, "value"=w1027:i32, "refnum out"=w1031:T9)  [unwired: 4 in, 1 out]
                        n317 = Bundle By Name(cluster=w1025, "ポートNo."=w1027) -> (w1024:T2)
                      }
                      frame 4 {
                        n318 = call-poly <vilib>:"Read Key.vi"("section"=w1039, "error in (no error)"=w1038, "key"=w1035, "refnum"=w1041) -> ("error out"=w1037:errorcluster, "value"=w1036:i32, "refnum out"=w1040:T9)  [unwired: 4 in, 1 out]
                        n319 = Bundle By Name(cluster=w1034, "測定モード"=w1036) -> (w1033:T2)
                      }
                      frame 5 {
                        n320 = call-poly <vilib>:"Read Key.vi"("section"=w1048, "error in (no error)"=w1047, "key"=w1044, "refnum"=w1050) -> ("error out"=w1046:errorcluster, "value"=w1045:string, "refnum out"=w1049:T9)  [unwired: 4 in, 1 out]
                        n321 = Bundle By Name(cluster=w1043, "規格単位"=w1045) -> (w1042:T2)
                      }
                      frame 6 {
                        n322 = call-poly <vilib>:"Read Key.vi"("section"=w1057, "error in (no error)"=w1056, "key"=w1053, "refnum"=w1059) -> ("error out"=w1055:errorcluster, "value"=w1054:string, "refnum out"=w1058:T9)  [unwired: 4 in, 1 out]
                        n323 = Bundle By Name(cluster=w1052, "品質チェック項目"=w1054) -> (w1051:T2)
                      }
                      frame 7 {
                        n324 = call-poly <vilib>:"Read Key.vi"("section"=w1066, "error in (no error)"=w1065, "key"=w1062, "refnum"=w1068) -> ("error out"=w1064:errorcluster, "value"=w1063:i32, "refnum out"=w1067:T9)  [unwired: 4 in, 1 out]
                        n325 = Bundle By Name(cluster=w1061, "測定周期"=w1063) -> (w1060:T2)
                      }
                      frame 8 {
                        n326 = call-poly <vilib>:"Read Key.vi"("section"=w1075, "error in (no error)"=w1074, "key"=w1071, "refnum"=w1077) -> ("error out"=w1073:errorcluster, "value"=w1072:string, "refnum out"=w1076:T9)  [unwired: 4 in, 1 out]
                        n327 = Bundle By Name(cluster=w1070, "実測値MAX"=w1072) -> (w1069:T2)
                      }
                      frame 9 {
                        n328 = call-poly <vilib>:"Read Key.vi"("section"=w1084, "error in (no error)"=w1083, "key"=w1080, "refnum"=w1086) -> ("error out"=w1082:errorcluster, "value"=w1081:string, "refnum out"=w1085:T9)  [unwired: 4 in, 1 out]
                        n329 = Bundle By Name(cluster=w1079, "実測値MIN"=w1081) -> (w1078:T2)
                      }
                      frame 10 {
                        n330 = call-poly <vilib>:"Read Key.vi"("section"=w1093, "error in (no error)"=w1092, "key"=w1089, "refnum"=w1095) -> ("error out"=w1091:errorcluster, "value"=w1090:string, "refnum out"=w1094:T9)  [unwired: 4 in, 1 out]
                        n331 = Bundle By Name(cluster=w1088, "実測値(MAX)"=w1090) -> (w1087:T2)
                      }
                      frame 11 {
                        n332 = call-poly <vilib>:"Read Key.vi"("section"=w1102, "error in (no error)"=w1101, "key"=w1098, "refnum"=w1104) -> ("error out"=w1100:errorcluster, "value"=w1099:string, "refnum out"=w1103:T9)  [unwired: 4 in, 1 out]
                        n333 = Bundle By Name(cluster=w1097, "実測値(MIN)"=w1099) -> (w1096:T2)
                      }
                      frame 12 {
                        n334 = call-poly <vilib>:"Read Key.vi"("section"=w1111, "error in (no error)"=w1110, "key"=w1107, "refnum"=w1113) -> ("error out"=w1109:errorcluster, "value"=w1108:bool, "refnum out"=w1112:T9)  [unwired: 4 in, 1 out]
                        n335 = Bundle By Name(cluster=w1106, "測定画面表示ボタン"=w1108) -> (w1105:T2)
                      }
                      frame 13 {
                        n336 = call-poly <vilib>:"Read Key.vi"("section"=w1120, "error in (no error)"=w1119, "key"=w1116, "refnum"=w1122) -> ("error out"=w1118:errorcluster, "value"=w1117:string, "refnum out"=w1121:T9)  [unwired: 4 in, 1 out]
                        n337 = Bundle By Name(cluster=w1115, "ゲージポートNo"=w1117) -> (w1114:T2)
                      }
                    }
                    n338 = local write "設定クラスタ_設定 5"(w988) -> ()
                  }
                  n339 = local read "使用ON/OFFボタン_設定 5"() -> (w973:T5)
                  n340 = call-poly <vilib>:"Read Key.vi"("section"=w963, "error in (no error)"=w984, "key"="使用ON/OFF", "refnum"=w986) -> ("error out"=w966:errorcluster, "value"=w975:bool, "refnum out"=w967:T9)  [unwired: 4 in, 1 out]
                  n341 = Bundle By Name(cluster=w973, "使用ON/OFF"=w975) -> (w972:T5)
                  n342 = local write "使用ON/OFFボタン_設定 5"(w972) -> ()
                  n343 = local read "CSV項目名 5"() -> (w970:T1)
                  n344 = call-poly <vilib>:"Read Key.vi"("section"=w963, "error in (no error)"=w966, "key"="CSVヘッダー名", "refnum"=w967) -> ("error out"=w965:errorcluster, "value"=w968:string, "refnum out"=w964:T9)  [unwired: 4 in, 1 out]
                  n345 = Bundle By Name(cluster=w970, "CSV項目名"=w968) -> (w971:T1)
                  n346 = local write "CSV項目名 5"(w971) -> ()
                }
                frame #1 {
                  # "⑮"
                  # "⑭"
                  # "⑩"
                  # "⑨"
                  # "測定モード設定時の動作"
                  n347 = local read "設定クラスタ_設定 5"() -> (w1127:T2)
                  n348 = Unbundle By Name(w1127) -> ("測定モード"=w1126:u16)
                  n349 = case shown="0, デフォルト" w1126 {
                    tunnel: w1127 -> [w1136 w1143 w1151]
                    tunnel: [w1135 w1142 w1150] -> w1125
                    tunnel: [T8."Enabled" ("無効") T8."Enabled" ("無効") T8."Disabled and Grayed Out" ("無効")] -> w1124
                    tunnel: [T8."Enabled" ("無効") T8."Enabled" ("無効") T8."Disabled and Grayed Out" ("無効")] -> w1123
                    frame 1 {
                      w1132 = ""
                      # "連続測定モードの場合MAXとMINを表示する"
                      n350 = Bundle By Name(cluster=w1136, "実測値MAX"="MAX", "実測値MIN"="MIN", "実測値(MAX)"=w1132, "実測値(MIN)"=w1132) -> (w1135:T2)
                    }
                    frame 2 {
                      w1139 = ""
                      # "多点測定モードの場合MAXとMINを表示する"
                      n351 = Bundle By Name(cluster=w1143, "実測値MAX"="MAX", "実測値MIN"="MIN", "実測値(MAX)"=w1139, "実測値(MIN)"=w1139) -> (w1142:T2)
                    }
                    frame 0, Default {
                      n352 = Bundle By Name(cluster=w1151, "実測値(MAX)"="", "実測値MAX"="値", "実測値(MIN)"="", "実測値MIN"="") -> (w1150:T2)
                    }
                  }
                  n353 = local write "設定クラスタ_設定 5"(w1125) -> ()
                  n354 = property on="実測値MIN" class="Str"("DisabledEnum"=w1124) -> ()  [unwired: 2 in, 2 out]
                  n355 = property on="実測値(MIN)" class="Str"("DisabledEnum"=w1123) -> ()  [unwired: 2 in, 2 out]
                }
              }
              n356 = Replace Array Subset(array=w957, new element=w954, index=4) -> (w958:T2[])
            }
            frame 5 {
              # "⑯"
              # "⑪"
              n357 = flat-sequence {
                tunnel: w1161 -> [w1177]
                tunnel: w1160 -> [w1178]
                tunnel: [w1163] -> w1155
                tunnel: [w1164] -> w1154
                tunnel: [w1328] -> w1159
                tunnel: [w1327] -> w1158
                tunnel: [w1326] -> w1153
                tunnel: w1155 -> [w1327]
                tunnel: w1154 -> [w1328]
                frame #0 {
                  w1162 = "設定6"
                  # "⑧"
                  # "⑦"
                  # "⑬"
                  # "⑫"
                  # "⑥"
                  # "⑤"
                  # "②"
                  # "①"
                  # "複製した時に変更する項目\n①②③④⑤⑥⑦⑧⑨⑩\nローカル変数\n⑪\n指標値\n⑫⑬\nセレクション\n⑭⑮\nプロパティノード設定直し\n⑯\n複製したケースのTrue定数を削除"
                  # "setting.iniファイルからの設定項目の読み取り"
                  n358 = local read "No設定クラスタ_設定 6"() -> (w1180:T7)
                  n359 = call-poly <vilib>:"Read Key.vi"("section"="No6.", "error in (no error)"=w1177, "key"="No.", "refnum"=w1178) -> ("error out"=w1184:errorcluster, "value"=w1176:i32, "refnum out"=w1186:T9)  [unwired: 4 in, 1 out]
                  n360 = Bundle By Name(cluster=w1180, "No."=w1176) -> (w1179:T7)
                  n361 = local write "No設定クラスタ_設定 6"(w1179) -> ()
                  n362 = for {
                    shift-right: [w1194] -> w1185
                    shift-left: w1186 -> [w1195]
                    shift-right: [w1191] -> w1183
                    shift-left: w1184 -> [w1192]
                    tunnel: string[] ["規格", "規格上限", "規格下限", "ポートNo.", "測定モード", "規格単位", "品質チェック項目", "測定周期", "実測MAX", "実測MIN", "実測(MAX)", "実測(MIN)", "測定画面表示ボタン", "ゲージポートNo."] -> [w1190] mode=indexing
                    tunnel: w1162 -> [w1189]
                    i -> [w1193]
                    # "④"
                    # "③"
                    n363 = local read "設定クラスタ_設定 6"() -> (w1188:T2)
                    n364 = case shown="0, デフォルト" w1193 {
                      tunnel: w1195 -> [w1204 w1213 w1222 w1231 w1240 w1249 w1258 w1267 w1276 w1285 w1294 w1303 w1312 w1321]
                      tunnel: [w1203 w1212 w1221 w1230 w1239 w1248 w1257 w1266 w1275 w1284 w1293 w1302 w1311 w1320] -> w1194
                      tunnel: w1189 -> [w1202 w1211 w1220 w1229 w1238 w1247 w1256 w1265 w1274 w1283 w1292 w1301 w1310 w1319]
                      tunnel: w1192 -> [w1201 w1210 w1219 w1228 w1237 w1246 w1255 w1264 w1273 w1282 w1291 w1300 w1309 w1318]
                      tunnel: [w1200 w1209 w1218 w1227 w1236 w1245 w1254 w1263 w1272 w1281 w1290 w1299 w1308 w1317] -> w1191
                      tunnel: w1190 -> [w1198 w1207 w1216 w1225 w1234 w1243 w1252 w1261 w1270 w1279 w1288 w1297 w1306 w1315]
                      tunnel: [w1197 w1205 w1214 w1223 w1232 w1241 w1250 w1259 w1268 w1277 w1286 w1295 w1304 w1313] -> w1187
                      tunnel: w1188 -> [w1196 w1206 w1215 w1224 w1233 w1242 w1251 w1260 w1269 w1278 w1287 w1296 w1305 w1314]
                      frame 0, Default {
                        n365 = call-poly <vilib>:"Read Key.vi"("section"=w1202, "error in (no error)"=w1201, "key"=w1198, "refnum"=w1204) -> ("error out"=w1200:errorcluster, "value"=w1199:string, "refnum out"=w1203:T9)  [unwired: 4 in, 1 out]
                        n366 = Bundle By Name(cluster=w1196, "規格"=w1199) -> (w1197:T2)
                      }
                      frame 1 {
                        n367 = call-poly <vilib>:"Read Key.vi"("section"=w1211, "error in (no error)"=w1210, "key"=w1207, "refnum"=w1213) -> ("error out"=w1209:errorcluster, "value"=w1208:string, "refnum out"=w1212:T9)  [unwired: 4 in, 1 out]
                        n368 = Bundle By Name(cluster=w1206, "規格上限"=w1208) -> (w1205:T2)
                      }
                      frame 2 {
                        n369 = call-poly <vilib>:"Read Key.vi"("section"=w1220, "error in (no error)"=w1219, "key"=w1216, "refnum"=w1222) -> ("error out"=w1218:errorcluster, "value"=w1217:string, "refnum out"=w1221:T9)  [unwired: 4 in, 1 out]
                        n370 = Bundle By Name(cluster=w1215, "規格下限"=w1217) -> (w1214:T2)
                      }
                      frame 3 {
                        n371 = call-poly <vilib>:"Read Key.vi"("section"=w1229, "error in (no error)"=w1228, "key"=w1225, "refnum"=w1231) -> ("error out"=w1227:errorcluster, "value"=w1226:i32, "refnum out"=w1230:T9)  [unwired: 4 in, 1 out]
                        n372 = Bundle By Name(cluster=w1224, "ポートNo."=w1226) -> (w1223:T2)
                      }
                      frame 4 {
                        n373 = call-poly <vilib>:"Read Key.vi"("section"=w1238, "error in (no error)"=w1237, "key"=w1234, "refnum"=w1240) -> ("error out"=w1236:errorcluster, "value"=w1235:i32, "refnum out"=w1239:T9)  [unwired: 4 in, 1 out]
                        n374 = Bundle By Name(cluster=w1233, "測定モード"=w1235) -> (w1232:T2)
                      }
                      frame 5 {
                        n375 = call-poly <vilib>:"Read Key.vi"("section"=w1247, "error in (no error)"=w1246, "key"=w1243, "refnum"=w1249) -> ("error out"=w1245:errorcluster, "value"=w1244:string, "refnum out"=w1248:T9)  [unwired: 4 in, 1 out]
                        n376 = Bundle By Name(cluster=w1242, "規格単位"=w1244) -> (w1241:T2)
                      }
                      frame 6 {
                        n377 = call-poly <vilib>:"Read Key.vi"("section"=w1256, "error in (no error)"=w1255, "key"=w1252, "refnum"=w1258) -> ("error out"=w1254:errorcluster, "value"=w1253:string, "refnum out"=w1257:T9)  [unwired: 4 in, 1 out]
                        n378 = Bundle By Name(cluster=w1251, "品質チェック項目"=w1253) -> (w1250:T2)
                      }
                      frame 7 {
                        n379 = call-poly <vilib>:"Read Key.vi"("section"=w1265, "error in (no error)"=w1264, "key"=w1261, "refnum"=w1267) -> ("error out"=w1263:errorcluster, "value"=w1262:i32, "refnum out"=w1266:T9)  [unwired: 4 in, 1 out]
                        n380 = Bundle By Name(cluster=w1260, "測定周期"=w1262) -> (w1259:T2)
                      }
                      frame 8 {
                        n381 = call-poly <vilib>:"Read Key.vi"("section"=w1274, "error in (no error)"=w1273, "key"=w1270, "refnum"=w1276) -> ("error out"=w1272:errorcluster, "value"=w1271:string, "refnum out"=w1275:T9)  [unwired: 4 in, 1 out]
                        n382 = Bundle By Name(cluster=w1269, "実測値MAX"=w1271) -> (w1268:T2)
                      }
                      frame 9 {
                        n383 = call-poly <vilib>:"Read Key.vi"("section"=w1283, "error in (no error)"=w1282, "key"=w1279, "refnum"=w1285) -> ("error out"=w1281:errorcluster, "value"=w1280:string, "refnum out"=w1284:T9)  [unwired: 4 in, 1 out]
                        n384 = Bundle By Name(cluster=w1278, "実測値MIN"=w1280) -> (w1277:T2)
                      }
                      frame 10 {
                        n385 = call-poly <vilib>:"Read Key.vi"("section"=w1292, "error in (no error)"=w1291, "key"=w1288, "refnum"=w1294) -> ("error out"=w1290:errorcluster, "value"=w1289:string, "refnum out"=w1293:T9)  [unwired: 4 in, 1 out]
                        n386 = Bundle By Name(cluster=w1287, "実測値(MAX)"=w1289) -> (w1286:T2)
                      }
                      frame 11 {
                        n387 = call-poly <vilib>:"Read Key.vi"("section"=w1301, "error in (no error)"=w1300, "key"=w1297, "refnum"=w1303) -> ("error out"=w1299:errorcluster, "value"=w1298:string, "refnum out"=w1302:T9)  [unwired: 4 in, 1 out]
                        n388 = Bundle By Name(cluster=w1296, "実測値(MIN)"=w1298) -> (w1295:T2)
                      }
                      frame 12 {
                        n389 = call-poly <vilib>:"Read Key.vi"("section"=w1310, "error in (no error)"=w1309, "key"=w1306, "refnum"=w1312) -> ("error out"=w1308:errorcluster, "value"=w1307:bool, "refnum out"=w1311:T9)  [unwired: 4 in, 1 out]
                        n390 = Bundle By Name(cluster=w1305, "測定画面表示ボタン"=w1307) -> (w1304:T2)
                      }
                      frame 13 {
                        n391 = call-poly <vilib>:"Read Key.vi"("section"=w1319, "error in (no error)"=w1318, "key"=w1315, "refnum"=w1321) -> ("error out"=w1317:errorcluster, "value"=w1316:string, "refnum out"=w1320:T9)  [unwired: 4 in, 1 out]
                        n392 = Bundle By Name(cluster=w1314, "ゲージポートNo"=w1316) -> (w1313:T2)
                      }
                    }
                    n393 = local write "設定クラスタ_設定 6"(w1187) -> ()
                  }
                  n394 = local read "使用ON/OFFボタン_設定 6"() -> (w1172:T5)
                  n395 = call-poly <vilib>:"Read Key.vi"("section"=w1162, "error in (no error)"=w1183, "key"="使用ON/OFF", "refnum"=w1185) -> ("error out"=w1165:errorcluster, "value"=w1174:bool, "refnum out"=w1166:T9)  [unwired: 4 in, 1 out]
                  n396 = Bundle By Name(cluster=w1172, "使用ON/OFF"=w1174) -> (w1171:T5)
                  n397 = local write "使用ON/OFFボタン_設定 6"(w1171) -> ()
                  n398 = local read "CSV項目名 6"() -> (w1169:T1)
                  n399 = call-poly <vilib>:"Read Key.vi"("section"=w1162, "error in (no error)"=w1165, "key"="CSVヘッダー名", "refnum"=w1166) -> ("error out"=w1164:errorcluster, "value"=w1167:string, "refnum out"=w1163:T9)  [unwired: 4 in, 1 out]
                  n400 = Bundle By Name(cluster=w1169, "CSV項目名"=w1167) -> (w1170:T1)
                  n401 = local write "CSV項目名 6"(w1170) -> ()
                }
                frame #1 {
                  # "⑮"
                  # "⑭"
                  # "⑩"
                  # "⑨"
                  # "測定モード設定時の動作"
                  n402 = local read "設定クラスタ_設定 6"() -> (w1326:T2)
                  n403 = Unbundle By Name(w1326) -> ("測定モード"=w1325:u16)
                  n404 = case shown="0, デフォルト" w1325 {
                    tunnel: w1326 -> [w1335 w1342 w1350]
                    tunnel: [w1334 w1341 w1349] -> w1324
                    tunnel: [T8."Enabled" ("無効") T8."Enabled" ("無効") T8."Disabled and Grayed Out" ("無効")] -> w1323
                    tunnel: [T8."Enabled" ("無効") T8."Enabled" ("無効") T8."Disabled and Grayed Out" ("無効")] -> w1322
                    frame 1 {
                      w1331 = ""
                      # "連続測定モードの場合MAXとMINを表示する"
                      n405 = Bundle By Name(cluster=w1335, "実測値MAX"="MAX", "実測値MIN"="MIN", "実測値(MAX)"=w1331, "実測値(MIN)"=w1331) -> (w1334:T2)
                    }
                    frame 2 {
                      w1338 = ""
                      # "多点測定モードの場合MAXとMINを表示する"
                      n406 = Bundle By Name(cluster=w1342, "実測値MAX"="MAX", "実測値MIN"="MIN", "実測値(MAX)"=w1338, "実測値(MIN)"=w1338) -> (w1341:T2)
                    }
                    frame 0, Default {
                      n407 = Bundle By Name(cluster=w1350, "実測値(MAX)"="", "実測値MAX"="値", "実測値(MIN)"="", "実測値MIN"="") -> (w1349:T2)
                    }
                  }
                  n408 = local write "設定クラスタ_設定 6"(w1324) -> ()
                  n409 = property on="実測値MIN" class="Str"("DisabledEnum"=w1323) -> ()  [unwired: 2 in, 2 out]
                  n410 = property on="実測値(MIN)" class="Str"("DisabledEnum"=w1322) -> ()  [unwired: 2 in, 2 out]
                }
              }
              n411 = Replace Array Subset(array=w1156, new element=w1153, index=5) -> (w1157:T2[])
            }
            frame 6 {
              # "⑯"
              # "⑪"
              n412 = flat-sequence {
                tunnel: w1360 -> [w1376]
                tunnel: w1359 -> [w1377]
                tunnel: [w1362] -> w1354
                tunnel: [w1363] -> w1353
                tunnel: [w1527] -> w1358
                tunnel: [w1526] -> w1357
                tunnel: [w1525] -> w1352
                tunnel: w1354 -> [w1526]
                tunnel: w1353 -> [w1527]
                frame #0 {
                  w1361 = "設定7"
                  # "⑧"
                  # "⑦"
                  # "⑬"
                  # "⑫"
                  # "⑥"
                  # "⑤"
                  # "②"
                  # "①"
                  # "複製した時に変更する項目\n①②③④⑤⑥⑦⑧⑨⑩\nローカル変数\n⑪\n指標値\n⑫⑬\nセレクション\n⑭⑮\nプロパティノード設定直し\n⑯\n複製したケースのTrue定数を削除"
                  # "setting.iniファイルからの設定項目の読み取り"
                  n413 = local read "No設定クラスタ_設定 7"() -> (w1379:T7)
                  n414 = call-poly <vilib>:"Read Key.vi"("section"="No7.", "error in (no error)"=w1376, "key"="No.", "refnum"=w1377) -> ("error out"=w1383:errorcluster, "value"=w1375:i32, "refnum out"=w1385:T9)  [unwired: 4 in, 1 out]
                  n415 = Bundle By Name(cluster=w1379, "No."=w1375) -> (w1378:T7)
                  n416 = local write "No設定クラスタ_設定 7"(w1378) -> ()
                  n417 = for {
                    shift-right: [w1393] -> w1384
                    shift-left: w1385 -> [w1394]
                    shift-right: [w1390] -> w1382
                    shift-left: w1383 -> [w1391]
                    tunnel: string[] ["規格", "規格上限", "規格下限", "ポートNo.", "測定モード", "規格単位", "品質チェック項目", "測定周期", "実測MAX", "実測MIN", "実測(MAX)", "実測(MIN)", "測定画面表示ボタン", "ゲージポートNo."] -> [w1389] mode=indexing
                    tunnel: w1361 -> [w1388]
                    i -> [w1392]
                    # "④"
                    # "③"
                    n418 = local read "設定クラスタ_設定 7"() -> (w1387:T2)
                    n419 = case shown="0, デフォルト" w1392 {
                      tunnel: w1394 -> [w1403 w1412 w1421 w1430 w1439 w1448 w1457 w1466 w1475 w1484 w1493 w1502 w1511 w1520]
                      tunnel: [w1402 w1411 w1420 w1429 w1438 w1447 w1456 w1465 w1474 w1483 w1492 w1501 w1510 w1519] -> w1393
                      tunnel: w1388 -> [w1401 w1410 w1419 w1428 w1437 w1446 w1455 w1464 w1473 w1482 w1491 w1500 w1509 w1518]
                      tunnel: w1391 -> [w1400 w1409 w1418 w1427 w1436 w1445 w1454 w1463 w1472 w1481 w1490 w1499 w1508 w1517]
                      tunnel: [w1399 w1408 w1417 w1426 w1435 w1444 w1453 w1462 w1471 w1480 w1489 w1498 w1507 w1516] -> w1390
                      tunnel: w1389 -> [w1397 w1406 w1415 w1424 w1433 w1442 w1451 w1460 w1469 w1478 w1487 w1496 w1505 w1514]
                      tunnel: [w1396 w1404 w1413 w1422 w1431 w1440 w1449 w1458 w1467 w1476 w1485 w1494 w1503 w1512] -> w1386
                      tunnel: w1387 -> [w1395 w1405 w1414 w1423 w1432 w1441 w1450 w1459 w1468 w1477 w1486 w1495 w1504 w1513]
                      frame 0, Default {
                        n420 = call-poly <vilib>:"Read Key.vi"("section"=w1401, "error in (no error)"=w1400, "key"=w1397, "refnum"=w1403) -> ("error out"=w1399:errorcluster, "value"=w1398:string, "refnum out"=w1402:T9)  [unwired: 4 in, 1 out]
                        n421 = Bundle By Name(cluster=w1395, "規格"=w1398) -> (w1396:T2)
                      }
                      frame 1 {
                        n422 = call-poly <vilib>:"Read Key.vi"("section"=w1410, "error in (no error)"=w1409, "key"=w1406, "refnum"=w1412) -> ("error out"=w1408:errorcluster, "value"=w1407:string, "refnum out"=w1411:T9)  [unwired: 4 in, 1 out]
                        n423 = Bundle By Name(cluster=w1405, "規格上限"=w1407) -> (w1404:T2)
                      }
                      frame 2 {
                        n424 = call-poly <vilib>:"Read Key.vi"("section"=w1419, "error in (no error)"=w1418, "key"=w1415, "refnum"=w1421) -> ("error out"=w1417:errorcluster, "value"=w1416:string, "refnum out"=w1420:T9)  [unwired: 4 in, 1 out]
                        n425 = Bundle By Name(cluster=w1414, "規格下限"=w1416) -> (w1413:T2)
                      }
                      frame 3 {
                        n426 = call-poly <vilib>:"Read Key.vi"("section"=w1428, "error in (no error)"=w1427, "key"=w1424, "refnum"=w1430) -> ("error out"=w1426:errorcluster, "value"=w1425:i32, "refnum out"=w1429:T9)  [unwired: 4 in, 1 out]
                        n427 = Bundle By Name(cluster=w1423, "ポートNo."=w1425) -> (w1422:T2)
                      }
                      frame 4 {
                        n428 = call-poly <vilib>:"Read Key.vi"("section"=w1437, "error in (no error)"=w1436, "key"=w1433, "refnum"=w1439) -> ("error out"=w1435:errorcluster, "value"=w1434:i32, "refnum out"=w1438:T9)  [unwired: 4 in, 1 out]
                        n429 = Bundle By Name(cluster=w1432, "測定モード"=w1434) -> (w1431:T2)
                      }
                      frame 5 {
                        n430 = call-poly <vilib>:"Read Key.vi"("section"=w1446, "error in (no error)"=w1445, "key"=w1442, "refnum"=w1448) -> ("error out"=w1444:errorcluster, "value"=w1443:string, "refnum out"=w1447:T9)  [unwired: 4 in, 1 out]
                        n431 = Bundle By Name(cluster=w1441, "規格単位"=w1443) -> (w1440:T2)
                      }
                      frame 6 {
                        n432 = call-poly <vilib>:"Read Key.vi"("section"=w1455, "error in (no error)"=w1454, "key"=w1451, "refnum"=w1457) -> ("error out"=w1453:errorcluster, "value"=w1452:string, "refnum out"=w1456:T9)  [unwired: 4 in, 1 out]
                        n433 = Bundle By Name(cluster=w1450, "品質チェック項目"=w1452) -> (w1449:T2)
                      }
                      frame 7 {
                        n434 = call-poly <vilib>:"Read Key.vi"("section"=w1464, "error in (no error)"=w1463, "key"=w1460, "refnum"=w1466) -> ("error out"=w1462:errorcluster, "value"=w1461:i32, "refnum out"=w1465:T9)  [unwired: 4 in, 1 out]
                        n435 = Bundle By Name(cluster=w1459, "測定周期"=w1461) -> (w1458:T2)
                      }
                      frame 8 {
                        n436 = call-poly <vilib>:"Read Key.vi"("section"=w1473, "error in (no error)"=w1472, "key"=w1469, "refnum"=w1475) -> ("error out"=w1471:errorcluster, "value"=w1470:string, "refnum out"=w1474:T9)  [unwired: 4 in, 1 out]
                        n437 = Bundle By Name(cluster=w1468, "実測値MAX"=w1470) -> (w1467:T2)
                      }
                      frame 9 {
                        n438 = call-poly <vilib>:"Read Key.vi"("section"=w1482, "error in (no error)"=w1481, "key"=w1478, "refnum"=w1484) -> ("error out"=w1480:errorcluster, "value"=w1479:string, "refnum out"=w1483:T9)  [unwired: 4 in, 1 out]
                        n439 = Bundle By Name(cluster=w1477, "実測値MIN"=w1479) -> (w1476:T2)
                      }
                      frame 10 {
                        n440 = call-poly <vilib>:"Read Key.vi"("section"=w1491, "error in (no error)"=w1490, "key"=w1487, "refnum"=w1493) -> ("error out"=w1489:errorcluster, "value"=w1488:string, "refnum out"=w1492:T9)  [unwired: 4 in, 1 out]
                        n441 = Bundle By Name(cluster=w1486, "実測値(MAX)"=w1488) -> (w1485:T2)
                      }
                      frame 11 {
                        n442 = call-poly <vilib>:"Read Key.vi"("section"=w1500, "error in (no error)"=w1499, "key"=w1496, "refnum"=w1502) -> ("error out"=w1498:errorcluster, "value"=w1497:string, "refnum out"=w1501:T9)  [unwired: 4 in, 1 out]
                        n443 = Bundle By Name(cluster=w1495, "実測値(MIN)"=w1497) -> (w1494:T2)
                      }
                      frame 12 {
                        n444 = call-poly <vilib>:"Read Key.vi"("section"=w1509, "error in (no error)"=w1508, "key"=w1505, "refnum"=w1511) -> ("error out"=w1507:errorcluster, "value"=w1506:bool, "refnum out"=w1510:T9)  [unwired: 4 in, 1 out]
                        n445 = Bundle By Name(cluster=w1504, "測定画面表示ボタン"=w1506) -> (w1503:T2)
                      }
                      frame 13 {
                        n446 = call-poly <vilib>:"Read Key.vi"("section"=w1518, "error in (no error)"=w1517, "key"=w1514, "refnum"=w1520) -> ("error out"=w1516:errorcluster, "value"=w1515:string, "refnum out"=w1519:T9)  [unwired: 4 in, 1 out]
                        n447 = Bundle By Name(cluster=w1513, "ゲージポートNo"=w1515) -> (w1512:T2)
                      }
                    }
                    n448 = local write "設定クラスタ_設定 7"(w1386) -> ()
                  }
                  n449 = local read "使用ON/OFFボタン_設定 7"() -> (w1371:T5)
                  n450 = call-poly <vilib>:"Read Key.vi"("section"=w1361, "error in (no error)"=w1382, "key"="使用ON/OFF", "refnum"=w1384) -> ("error out"=w1364:errorcluster, "value"=w1373:bool, "refnum out"=w1365:T9)  [unwired: 4 in, 1 out]
                  n451 = Bundle By Name(cluster=w1371, "使用ON/OFF"=w1373) -> (w1370:T5)
                  n452 = local write "使用ON/OFFボタン_設定 7"(w1370) -> ()
                  n453 = local read "CSV項目名 7"() -> (w1368:T1)
                  n454 = call-poly <vilib>:"Read Key.vi"("section"=w1361, "error in (no error)"=w1364, "key"="CSVヘッダー名", "refnum"=w1365) -> ("error out"=w1363:errorcluster, "value"=w1366:string, "refnum out"=w1362:T9)  [unwired: 4 in, 1 out]
                  n455 = Bundle By Name(cluster=w1368, "CSV項目名"=w1366) -> (w1369:T1)
                  n456 = local write "CSV項目名 7"(w1369) -> ()
                }
                frame #1 {
                  # "⑮"
                  # "⑭"
                  # "⑩"
                  # "⑨"
                  # "測定モード設定時の動作"
                  n457 = local read "設定クラスタ_設定 7"() -> (w1525:T2)
                  n458 = Unbundle By Name(w1525) -> ("測定モード"=w1524:u16)
                  n459 = case shown="0, デフォルト" w1524 {
                    tunnel: w1525 -> [w1534 w1541 w1549]
                    tunnel: [w1533 w1540 w1548] -> w1523
                    tunnel: [T8."Enabled" ("無効") T8."Enabled" ("無効") T8."Disabled and Grayed Out" ("無効")] -> w1522
                    tunnel: [T8."Enabled" ("無効") T8."Enabled" ("無効") T8."Disabled and Grayed Out" ("無効")] -> w1521
                    frame 1 {
                      w1530 = ""
                      # "連続測定モードの場合MAXとMINを表示する"
                      n460 = Bundle By Name(cluster=w1534, "実測値MAX"="MAX", "実測値MIN"="MIN", "実測値(MAX)"=w1530, "実測値(MIN)"=w1530) -> (w1533:T2)
                    }
                    frame 2 {
                      w1537 = ""
                      # "多点測定モードの場合MAXとMINを表示する"
                      n461 = Bundle By Name(cluster=w1541, "実測値MAX"="MAX", "実測値MIN"="MIN", "実測値(MAX)"=w1537, "実測値(MIN)"=w1537) -> (w1540:T2)
                    }
                    frame 0, Default {
                      n462 = Bundle By Name(cluster=w1549, "実測値(MAX)"="", "実測値MAX"="値", "実測値(MIN)"="", "実測値MIN"="") -> (w1548:T2)
                    }
                  }
                  n463 = local write "設定クラスタ_設定 7"(w1523) -> ()
                  n464 = property on="実測値MIN" class="Str"("DisabledEnum"=w1522) -> ()  [unwired: 2 in, 2 out]
                  n465 = property on="実測値(MIN)" class="Str"("DisabledEnum"=w1521) -> ()  [unwired: 2 in, 2 out]
                }
              }
              n466 = Replace Array Subset(array=w1355, new element=w1352, index=6) -> (w1356:T2[])
            }
            frame 7 {
              # "⑯"
              # "⑪"
              n467 = flat-sequence {
                tunnel: w1559 -> [w1575]
                tunnel: w1558 -> [w1576]
                tunnel: [w1561] -> w1553
                tunnel: [w1562] -> w1552
                tunnel: [w1726] -> w1557
                tunnel: [w1725] -> w1556
                tunnel: [w1724] -> w1551
                tunnel: w1553 -> [w1725]
                tunnel: w1552 -> [w1726]
                frame #0 {
                  w1560 = "設定8"
                  # "⑧"
                  # "⑦"
                  # "⑬"
                  # "⑫"
                  # "⑥"
                  # "⑤"
                  # "②"
                  # "①"
                  # "複製した時に変更する項目\n①②③④⑤⑥⑦⑧⑨⑩\nローカル変数\n⑪\n指標値\n⑫⑬\nセレクション\n⑭⑮\nプロパティノード設定直し\n⑯\n複製したケースのTrue定数を削除"
                  # "setting.iniファイルからの設定項目の読み取り"
                  n468 = local read "No設定クラスタ_設定 8"() -> (w1578:T7)
                  n469 = call-poly <vilib>:"Read Key.vi"("section"="No8.", "error in (no error)"=w1575, "key"="No.", "refnum"=w1576) -> ("error out"=w1582:errorcluster, "value"=w1574:i32, "refnum out"=w1584:T9)  [unwired: 4 in, 1 out]
                  n470 = Bundle By Name(cluster=w1578, "No."=w1574) -> (w1577:T7)
                  n471 = local write "No設定クラスタ_設定 8"(w1577) -> ()
                  n472 = for {
                    shift-right: [w1592] -> w1583
                    shift-left: w1584 -> [w1593]
                    shift-right: [w1589] -> w1581
                    shift-left: w1582 -> [w1590]
                    tunnel: string[] ["規格", "規格上限", "規格下限", "ポートNo.", "測定モード", "規格単位", "品質チェック項目", "測定周期", "実測MAX", "実測MIN", "実測(MAX)", "実測(MIN)", "測定画面表示ボタン", "ゲージポートNo."] -> [w1588] mode=indexing
                    tunnel: w1560 -> [w1587]
                    i -> [w1591]
                    # "④"
                    # "③"
                    n473 = local read "設定クラスタ_設定 8"() -> (w1586:T2)
                    n474 = case shown="0, デフォルト" w1591 {
                      tunnel: w1593 -> [w1602 w1611 w1620 w1629 w1638 w1647 w1656 w1665 w1674 w1683 w1692 w1701 w1710 w1719]
                      tunnel: [w1601 w1610 w1619 w1628 w1637 w1646 w1655 w1664 w1673 w1682 w1691 w1700 w1709 w1718] -> w1592
                      tunnel: w1587 -> [w1600 w1609 w1618 w1627 w1636 w1645 w1654 w1663 w1672 w1681 w1690 w1699 w1708 w1717]
                      tunnel: w1590 -> [w1599 w1608 w1617 w1626 w1635 w1644 w1653 w1662 w1671 w1680 w1689 w1698 w1707 w1716]
                      tunnel: [w1598 w1607 w1616 w1625 w1634 w1643 w1652 w1661 w1670 w1679 w1688 w1697 w1706 w1715] -> w1589
                      tunnel: w1588 -> [w1596 w1605 w1614 w1623 w1632 w1641 w1650 w1659 w1668 w1677 w1686 w1695 w1704 w1713]
                      tunnel: [w1595 w1603 w1612 w1621 w1630 w1639 w1648 w1657 w1666 w1675 w1684 w1693 w1702 w1711] -> w1585
                      tunnel: w1586 -> [w1594 w1604 w1613 w1622 w1631 w1640 w1649 w1658 w1667 w1676 w1685 w1694 w1703 w1712]
                      frame 0, Default {
                        n475 = call-poly <vilib>:"Read Key.vi"("section"=w1600, "error in (no error)"=w1599, "key"=w1596, "refnum"=w1602) -> ("error out"=w1598:errorcluster, "value"=w1597:string, "refnum out"=w1601:T9)  [unwired: 4 in, 1 out]
                        n476 = Bundle By Name(cluster=w1594, "規格"=w1597) -> (w1595:T2)
                      }
                      frame 1 {
                        n477 = call-poly <vilib>:"Read Key.vi"("section"=w1609, "error in (no error)"=w1608, "key"=w1605, "refnum"=w1611) -> ("error out"=w1607:errorcluster, "value"=w1606:string, "refnum out"=w1610:T9)  [unwired: 4 in, 1 out]
                        n478 = Bundle By Name(cluster=w1604, "規格上限"=w1606) -> (w1603:T2)
                      }
                      frame 2 {
                        n479 = call-poly <vilib>:"Read Key.vi"("section"=w1618, "error in (no error)"=w1617, "key"=w1614, "refnum"=w1620) -> ("error out"=w1616:errorcluster, "value"=w1615:string, "refnum out"=w1619:T9)  [unwired: 4 in, 1 out]
                        n480 = Bundle By Name(cluster=w1613, "規格下限"=w1615) -> (w1612:T2)
                      }
                      frame 3 {
                        n481 = call-poly <vilib>:"Read Key.vi"("section"=w1627, "error in (no error)"=w1626, "key"=w1623, "refnum"=w1629) -> ("error out"=w1625:errorcluster, "value"=w1624:i32, "refnum out"=w1628:T9)  [unwired: 4 in, 1 out]
                        n482 = Bundle By Name(cluster=w1622, "ポートNo."=w1624) -> (w1621:T2)
                      }
                      frame 4 {
                        n483 = call-poly <vilib>:"Read Key.vi"("section"=w1636, "error in (no error)"=w1635, "key"=w1632, "refnum"=w1638) -> ("error out"=w1634:errorcluster, "value"=w1633:i32, "refnum out"=w1637:T9)  [unwired: 4 in, 1 out]
                        n484 = Bundle By Name(cluster=w1631, "測定モード"=w1633) -> (w1630:T2)
                      }
                      frame 5 {
                        n485 = call-poly <vilib>:"Read Key.vi"("section"=w1645, "error in (no error)"=w1644, "key"=w1641, "refnum"=w1647) -> ("error out"=w1643:errorcluster, "value"=w1642:string, "refnum out"=w1646:T9)  [unwired: 4 in, 1 out]
                        n486 = Bundle By Name(cluster=w1640, "規格単位"=w1642) -> (w1639:T2)
                      }
                      frame 6 {
                        n487 = call-poly <vilib>:"Read Key.vi"("section"=w1654, "error in (no error)"=w1653, "key"=w1650, "refnum"=w1656) -> ("error out"=w1652:errorcluster, "value"=w1651:string, "refnum out"=w1655:T9)  [unwired: 4 in, 1 out]
                        n488 = Bundle By Name(cluster=w1649, "品質チェック項目"=w1651) -> (w1648:T2)
                      }
                      frame 7 {
                        n489 = call-poly <vilib>:"Read Key.vi"("section"=w1663, "error in (no error)"=w1662, "key"=w1659, "refnum"=w1665) -> ("error out"=w1661:errorcluster, "value"=w1660:i32, "refnum out"=w1664:T9)  [unwired: 4 in, 1 out]
                        n490 = Bundle By Name(cluster=w1658, "測定周期"=w1660) -> (w1657:T2)
                      }
                      frame 8 {
                        n491 = call-poly <vilib>:"Read Key.vi"("section"=w1672, "error in (no error)"=w1671, "key"=w1668, "refnum"=w1674) -> ("error out"=w1670:errorcluster, "value"=w1669:string, "refnum out"=w1673:T9)  [unwired: 4 in, 1 out]
                        n492 = Bundle By Name(cluster=w1667, "実測値MAX"=w1669) -> (w1666:T2)
                      }
                      frame 9 {
                        n493 = call-poly <vilib>:"Read Key.vi"("section"=w1681, "error in (no error)"=w1680, "key"=w1677, "refnum"=w1683) -> ("error out"=w1679:errorcluster, "value"=w1678:string, "refnum out"=w1682:T9)  [unwired: 4 in, 1 out]
                        n494 = Bundle By Name(cluster=w1676, "実測値MIN"=w1678) -> (w1675:T2)
                      }
                      frame 10 {
                        n495 = call-poly <vilib>:"Read Key.vi"("section"=w1690, "error in (no error)"=w1689, "key"=w1686, "refnum"=w1692) -> ("error out"=w1688:errorcluster, "value"=w1687:string, "refnum out"=w1691:T9)  [unwired: 4 in, 1 out]
                        n496 = Bundle By Name(cluster=w1685, "実測値(MAX)"=w1687) -> (w1684:T2)
                      }
                      frame 11 {
                        n497 = call-poly <vilib>:"Read Key.vi"("section"=w1699, "error in (no error)"=w1698, "key"=w1695, "refnum"=w1701) -> ("error out"=w1697:errorcluster, "value"=w1696:string, "refnum out"=w1700:T9)  [unwired: 4 in, 1 out]
                        n498 = Bundle By Name(cluster=w1694, "実測値(MIN)"=w1696) -> (w1693:T2)
                      }
                      frame 12 {
                        n499 = call-poly <vilib>:"Read Key.vi"("section"=w1708, "error in (no error)"=w1707, "key"=w1704, "refnum"=w1710) -> ("error out"=w1706:errorcluster, "value"=w1705:bool, "refnum out"=w1709:T9)  [unwired: 4 in, 1 out]
                        n500 = Bundle By Name(cluster=w1703, "測定画面表示ボタン"=w1705) -> (w1702:T2)
                      }
                      frame 13 {
                        n501 = call-poly <vilib>:"Read Key.vi"("section"=w1717, "error in (no error)"=w1716, "key"=w1713, "refnum"=w1719) -> ("error out"=w1715:errorcluster, "value"=w1714:string, "refnum out"=w1718:T9)  [unwired: 4 in, 1 out]
                        n502 = Bundle By Name(cluster=w1712, "ゲージポートNo"=w1714) -> (w1711:T2)
                      }
                    }
                    n503 = local write "設定クラスタ_設定 8"(w1585) -> ()
                  }
                  n504 = local read "使用ON/OFFボタン_設定 8"() -> (w1570:T5)
                  n505 = call-poly <vilib>:"Read Key.vi"("section"=w1560, "error in (no error)"=w1581, "key"="使用ON/OFF", "refnum"=w1583) -> ("error out"=w1563:errorcluster, "value"=w1572:bool, "refnum out"=w1564:T9)  [unwired: 4 in, 1 out]
                  n506 = Bundle By Name(cluster=w1570, "使用ON/OFF"=w1572) -> (w1569:T5)
                  n507 = local write "使用ON/OFFボタン_設定 8"(w1569) -> ()
                  n508 = local read "CSV項目名 8"() -> (w1567:T1)
                  n509 = call-poly <vilib>:"Read Key.vi"("section"=w1560, "error in (no error)"=w1563, "key"="CSVヘッダー名", "refnum"=w1564) -> ("error out"=w1562:errorcluster, "value"=w1565:string, "refnum out"=w1561:T9)  [unwired: 4 in, 1 out]
                  n510 = Bundle By Name(cluster=w1567, "CSV項目名"=w1565) -> (w1568:T1)
                  n511 = local write "CSV項目名 8"(w1568) -> ()
                }
                frame #1 {
                  # "⑮"
                  # "⑭"
                  # "⑩"
                  # "⑨"
                  # "測定モード設定時の動作"
                  n512 = local read "設定クラスタ_設定 8"() -> (w1724:T2)
                  n513 = Unbundle By Name(w1724) -> ("測定モード"=w1723:u16)
                  n514 = case shown="0, デフォルト" w1723 {
                    tunnel: w1724 -> [w1733 w1740 w1748]
                    tunnel: [w1732 w1739 w1747] -> w1722
                    tunnel: [T8."Enabled" ("無効") T8."Enabled" ("無効") T8."Disabled and Grayed Out" ("無効")] -> w1721
                    tunnel: [T8."Enabled" ("無効") T8."Enabled" ("無効") T8."Disabled and Grayed Out" ("無効")] -> w1720
                    frame 1 {
                      w1729 = ""
                      # "連続測定モードの場合MAXとMINを表示する"
                      n515 = Bundle By Name(cluster=w1733, "実測値MAX"="MAX", "実測値MIN"="MIN", "実測値(MAX)"=w1729, "実測値(MIN)"=w1729) -> (w1732:T2)
                    }
                    frame 2 {
                      w1736 = ""
                      # "多点測定モードの場合MAXとMINを表示する"
                      n516 = Bundle By Name(cluster=w1740, "実測値MAX"="MAX", "実測値MIN"="MIN", "実測値(MAX)"=w1736, "実測値(MIN)"=w1736) -> (w1739:T2)
                    }
                    frame 0, Default {
                      n517 = Bundle By Name(cluster=w1748, "実測値(MAX)"="", "実測値MAX"="値", "実測値(MIN)"="", "実測値MIN"="") -> (w1747:T2)
                    }
                  }
                  n518 = local write "設定クラスタ_設定 8"(w1722) -> ()
                  n519 = property on="実測値MIN" class="Str"("DisabledEnum"=w1721) -> ()  [unwired: 2 in, 2 out]
                  n520 = property on="実測値(MIN)" class="Str"("DisabledEnum"=w1720) -> ()  [unwired: 2 in, 2 out]
                }
              }
              n521 = Replace Array Subset(array=w1554, new element=w1551, index=7) -> (w1555:T2[])
            }
            frame 8 {
              # "⑯"
              # "⑪"
              n522 = flat-sequence {
                tunnel: w1758 -> [w1774]
                tunnel: w1757 -> [w1775]
                tunnel: [w1760] -> w1752
                tunnel: [w1761] -> w1751
                tunnel: [w1925] -> w1756
                tunnel: [w1924] -> w1755
                tunnel: [w1923] -> w1750
                tunnel: w1752 -> [w1924]
                tunnel: w1751 -> [w1925]
                frame #0 {
                  w1759 = "設定9"
                  # "⑧"
                  # "⑦"
                  # "⑬"
                  # "⑫"
                  # "⑥"
                  # "⑤"
                  # "②"
                  # "①"
                  # "複製した時に変更する項目\n①②③④⑤⑥⑦⑧⑨⑩\nローカル変数\n⑪\n指標値\n⑫⑬\nセレクション\n⑭⑮\nプロパティノード設定直し\n⑯\n複製したケースのTrue定数を削除"
                  # "setting.iniファイルからの設定項目の読み取り"
                  n523 = local read "No設定クラスタ_設定 9"() -> (w1777:T7)
                  n524 = call-poly <vilib>:"Read Key.vi"("section"="No9.", "error in (no error)"=w1774, "key"="No.", "refnum"=w1775) -> ("error out"=w1781:errorcluster, "value"=w1773:i32, "refnum out"=w1783:T9)  [unwired: 4 in, 1 out]
                  n525 = Bundle By Name(cluster=w1777, "No."=w1773) -> (w1776:T7)
                  n526 = local write "No設定クラスタ_設定 9"(w1776) -> ()
                  n527 = for {
                    shift-right: [w1791] -> w1782
                    shift-left: w1783 -> [w1792]
                    shift-right: [w1788] -> w1780
                    shift-left: w1781 -> [w1789]
                    tunnel: string[] ["規格", "規格上限", "規格下限", "ポートNo.", "測定モード", "規格単位", "品質チェック項目", "測定周期", "実測MAX", "実測MIN", "実測(MAX)", "実測(MIN)", "測定画面表示ボタン", "ゲージポートNo."] -> [w1787] mode=indexing
                    tunnel: w1759 -> [w1786]
                    i -> [w1790]
                    # "④"
                    # "③"
                    n528 = local read "設定クラスタ_設定 9"() -> (w1785:T2)
                    n529 = case shown="0, デフォルト" w1790 {
                      tunnel: w1792 -> [w1801 w1810 w1819 w1828 w1837 w1846 w1855 w1864 w1873 w1882 w1891 w1900 w1909 w1918]
                      tunnel: [w1800 w1809 w1818 w1827 w1836 w1845 w1854 w1863 w1872 w1881 w1890 w1899 w1908 w1917] -> w1791
                      tunnel: w1786 -> [w1799 w1808 w1817 w1826 w1835 w1844 w1853 w1862 w1871 w1880 w1889 w1898 w1907 w1916]
                      tunnel: w1789 -> [w1798 w1807 w1816 w1825 w1834 w1843 w1852 w1861 w1870 w1879 w1888 w1897 w1906 w1915]
                      tunnel: [w1797 w1806 w1815 w1824 w1833 w1842 w1851 w1860 w1869 w1878 w1887 w1896 w1905 w1914] -> w1788
                      tunnel: w1787 -> [w1795 w1804 w1813 w1822 w1831 w1840 w1849 w1858 w1867 w1876 w1885 w1894 w1903 w1912]
                      tunnel: [w1794 w1802 w1811 w1820 w1829 w1838 w1847 w1856 w1865 w1874 w1883 w1892 w1901 w1910] -> w1784
                      tunnel: w1785 -> [w1793 w1803 w1812 w1821 w1830 w1839 w1848 w1857 w1866 w1875 w1884 w1893 w1902 w1911]
                      frame 0, Default {
                        n530 = call-poly <vilib>:"Read Key.vi"("section"=w1799, "error in (no error)"=w1798, "key"=w1795, "refnum"=w1801) -> ("error out"=w1797:errorcluster, "value"=w1796:string, "refnum out"=w1800:T9)  [unwired: 4 in, 1 out]
                        n531 = Bundle By Name(cluster=w1793, "規格"=w1796) -> (w1794:T2)
                      }
                      frame 1 {
                        n532 = call-poly <vilib>:"Read Key.vi"("section"=w1808, "error in (no error)"=w1807, "key"=w1804, "refnum"=w1810) -> ("error out"=w1806:errorcluster, "value"=w1805:string, "refnum out"=w1809:T9)  [unwired: 4 in, 1 out]
                        n533 = Bundle By Name(cluster=w1803, "規格上限"=w1805) -> (w1802:T2)
                      }
                      frame 2 {
                        n534 = call-poly <vilib>:"Read Key.vi"("section"=w1817, "error in (no error)"=w1816, "key"=w1813, "refnum"=w1819) -> ("error out"=w1815:errorcluster, "value"=w1814:string, "refnum out"=w1818:T9)  [unwired: 4 in, 1 out]
                        n535 = Bundle By Name(cluster=w1812, "規格下限"=w1814) -> (w1811:T2)
                      }
                      frame 3 {
                        n536 = call-poly <vilib>:"Read Key.vi"("section"=w1826, "error in (no error)"=w1825, "key"=w1822, "refnum"=w1828) -> ("error out"=w1824:errorcluster, "value"=w1823:i32, "refnum out"=w1827:T9)  [unwired: 4 in, 1 out]
                        n537 = Bundle By Name(cluster=w1821, "ポートNo."=w1823) -> (w1820:T2)
                      }
                      frame 4 {
                        n538 = call-poly <vilib>:"Read Key.vi"("section"=w1835, "error in (no error)"=w1834, "key"=w1831, "refnum"=w1837) -> ("error out"=w1833:errorcluster, "value"=w1832:i32, "refnum out"=w1836:T9)  [unwired: 4 in, 1 out]
                        n539 = Bundle By Name(cluster=w1830, "測定モード"=w1832) -> (w1829:T2)
                      }
                      frame 5 {
                        n540 = call-poly <vilib>:"Read Key.vi"("section"=w1844, "error in (no error)"=w1843, "key"=w1840, "refnum"=w1846) -> ("error out"=w1842:errorcluster, "value"=w1841:string, "refnum out"=w1845:T9)  [unwired: 4 in, 1 out]
                        n541 = Bundle By Name(cluster=w1839, "規格単位"=w1841) -> (w1838:T2)
                      }
                      frame 6 {
                        n542 = call-poly <vilib>:"Read Key.vi"("section"=w1853, "error in (no error)"=w1852, "key"=w1849, "refnum"=w1855) -> ("error out"=w1851:errorcluster, "value"=w1850:string, "refnum out"=w1854:T9)  [unwired: 4 in, 1 out]
                        n543 = Bundle By Name(cluster=w1848, "品質チェック項目"=w1850) -> (w1847:T2)
                      }
                      frame 7 {
                        n544 = call-poly <vilib>:"Read Key.vi"("section"=w1862, "error in (no error)"=w1861, "key"=w1858, "refnum"=w1864) -> ("error out"=w1860:errorcluster, "value"=w1859:i32, "refnum out"=w1863:T9)  [unwired: 4 in, 1 out]
                        n545 = Bundle By Name(cluster=w1857, "測定周期"=w1859) -> (w1856:T2)
                      }
                      frame 8 {
                        n546 = call-poly <vilib>:"Read Key.vi"("section"=w1871, "error in (no error)"=w1870, "key"=w1867, "refnum"=w1873) -> ("error out"=w1869:errorcluster, "value"=w1868:string, "refnum out"=w1872:T9)  [unwired: 4 in, 1 out]
                        n547 = Bundle By Name(cluster=w1866, "実測値MAX"=w1868) -> (w1865:T2)
                      }
                      frame 9 {
                        n548 = call-poly <vilib>:"Read Key.vi"("section"=w1880, "error in (no error)"=w1879, "key"=w1876, "refnum"=w1882) -> ("error out"=w1878:errorcluster, "value"=w1877:string, "refnum out"=w1881:T9)  [unwired: 4 in, 1 out]
                        n549 = Bundle By Name(cluster=w1875, "実測値MIN"=w1877) -> (w1874:T2)
                      }
                      frame 10 {
                        n550 = call-poly <vilib>:"Read Key.vi"("section"=w1889, "error in (no error)"=w1888, "key"=w1885, "refnum"=w1891) -> ("error out"=w1887:errorcluster, "value"=w1886:string, "refnum out"=w1890:T9)  [unwired: 4 in, 1 out]
                        n551 = Bundle By Name(cluster=w1884, "実測値(MAX)"=w1886) -> (w1883:T2)
                      }
                      frame 11 {
                        n552 = call-poly <vilib>:"Read Key.vi"("section"=w1898, "error in (no error)"=w1897, "key"=w1894, "refnum"=w1900) -> ("error out"=w1896:errorcluster, "value"=w1895:string, "refnum out"=w1899:T9)  [unwired: 4 in, 1 out]
                        n553 = Bundle By Name(cluster=w1893, "実測値(MIN)"=w1895) -> (w1892:T2)
                      }
                      frame 12 {
                        n554 = call-poly <vilib>:"Read Key.vi"("section"=w1907, "error in (no error)"=w1906, "key"=w1903, "refnum"=w1909) -> ("error out"=w1905:errorcluster, "value"=w1904:bool, "refnum out"=w1908:T9)  [unwired: 4 in, 1 out]
                        n555 = Bundle By Name(cluster=w1902, "測定画面表示ボタン"=w1904) -> (w1901:T2)
                      }
                      frame 13 {
                        n556 = call-poly <vilib>:"Read Key.vi"("section"=w1916, "error in (no error)"=w1915, "key"=w1912, "refnum"=w1918) -> ("error out"=w1914:errorcluster, "value"=w1913:string, "refnum out"=w1917:T9)  [unwired: 4 in, 1 out]
                        n557 = Bundle By Name(cluster=w1911, "ゲージポートNo"=w1913) -> (w1910:T2)
                      }
                    }
                    n558 = local write "設定クラスタ_設定 9"(w1784) -> ()
                  }
                  n559 = local read "使用ON/OFFボタン_設定 9"() -> (w1769:T5)
                  n560 = call-poly <vilib>:"Read Key.vi"("section"=w1759, "error in (no error)"=w1780, "key"="使用ON/OFF", "refnum"=w1782) -> ("error out"=w1762:errorcluster, "value"=w1771:bool, "refnum out"=w1763:T9)  [unwired: 4 in, 1 out]
                  n561 = Bundle By Name(cluster=w1769, "使用ON/OFF"=w1771) -> (w1768:T5)
                  n562 = local write "使用ON/OFFボタン_設定 9"(w1768) -> ()
                  n563 = local read "CSV項目名 9"() -> (w1766:T1)
                  n564 = call-poly <vilib>:"Read Key.vi"("section"=w1759, "error in (no error)"=w1762, "key"="CSVヘッダー名", "refnum"=w1763) -> ("error out"=w1761:errorcluster, "value"=w1764:string, "refnum out"=w1760:T9)  [unwired: 4 in, 1 out]
                  n565 = Bundle By Name(cluster=w1766, "CSV項目名"=w1764) -> (w1767:T1)
                  n566 = local write "CSV項目名 9"(w1767) -> ()
                }
                frame #1 {
                  # "⑮"
                  # "⑭"
                  # "⑩"
                  # "⑨"
                  # "測定モード設定時の動作"
                  n567 = local read "設定クラスタ_設定 9"() -> (w1923:T2)
                  n568 = Unbundle By Name(w1923) -> ("測定モード"=w1922:u16)
                  n569 = case shown="0, デフォルト" w1922 {
                    tunnel: w1923 -> [w1932 w1939 w1947]
                    tunnel: [w1931 w1938 w1946] -> w1921
                    tunnel: [T8."Enabled" ("無効") T8."Enabled" ("無効") T8."Disabled and Grayed Out" ("無効")] -> w1920
                    tunnel: [T8."Enabled" ("無効") T8."Enabled" ("無効") T8."Disabled and Grayed Out" ("無効")] -> w1919
                    frame 1 {
                      w1928 = ""
                      # "連続測定モードの場合MAXとMINを表示する"
                      n570 = Bundle By Name(cluster=w1932, "実測値MAX"="MAX", "実測値MIN"="MIN", "実測値(MAX)"=w1928, "実測値(MIN)"=w1928) -> (w1931:T2)
                    }
                    frame 2 {
                      w1935 = ""
                      # "多点測定モードの場合MAXとMINを表示する"
                      n571 = Bundle By Name(cluster=w1939, "実測値MAX"="MAX", "実測値MIN"="MIN", "実測値(MAX)"=w1935, "実測値(MIN)"=w1935) -> (w1938:T2)
                    }
                    frame 0, Default {
                      n572 = Bundle By Name(cluster=w1947, "実測値(MAX)"="", "実測値MAX"="値", "実測値(MIN)"="", "実測値MIN"="") -> (w1946:T2)
                    }
                  }
                  n573 = local write "設定クラスタ_設定 9"(w1921) -> ()
                  n574 = property on="実測値MIN" class="Str"("DisabledEnum"=w1920) -> ()  [unwired: 2 in, 2 out]
                  n575 = property on="実測値(MIN)" class="Str"("DisabledEnum"=w1919) -> ()  [unwired: 2 in, 2 out]
                }
              }
              n576 = Replace Array Subset(array=w1753, new element=w1750, index=8) -> (w1754:T2[])
            }
            frame 9 {
              # "⑯"
              # "⑪"
              n577 = flat-sequence {
                tunnel: w1957 -> [w1973]
                tunnel: w1956 -> [w1974]
                tunnel: [w1959] -> w1951
                tunnel: [w1960] -> w1950
                tunnel: [w2124] -> w1955
                tunnel: [w2123] -> w1954
                tunnel: [w2122] -> w1949
                tunnel: w1951 -> [w2123]
                tunnel: w1950 -> [w2124]
                frame #0 {
                  w1958 = "設定10"
                  # "⑧"
                  # "⑦"
                  # "⑬"
                  # "⑫"
                  # "⑥"
                  # "⑤"
                  # "②"
                  # "①"
                  # "複製した時に変更する項目\n①②③④⑤⑥⑦⑧⑨⑩\nローカル変数\n⑪\n指標値\n⑫⑬\nセレクション\n⑭⑮\nプロパティノード設定直し\n⑯\n複製したケースのTrue定数を削除"
                  # "setting.iniファイルからの設定項目の読み取り"
                  n578 = local read "No設定クラスタ_設定 10"() -> (w1976:T7)
                  n579 = call-poly <vilib>:"Read Key.vi"("section"="No10.", "error in (no error)"=w1973, "key"="No.", "refnum"=w1974) -> ("error out"=w1980:errorcluster, "value"=w1972:i32, "refnum out"=w1982:T9)  [unwired: 4 in, 1 out]
                  n580 = Bundle By Name(cluster=w1976, "No."=w1972) -> (w1975:T7)
                  n581 = local write "No設定クラスタ_設定 10"(w1975) -> ()
                  n582 = for {
                    shift-right: [w1990] -> w1981
                    shift-left: w1982 -> [w1991]
                    shift-right: [w1987] -> w1979
                    shift-left: w1980 -> [w1988]
                    tunnel: string[] ["規格", "規格上限", "規格下限", "ポートNo.", "測定モード", "規格単位", "品質チェック項目", "測定周期", "実測MAX", "実測MIN", "実測(MAX)", "実測(MIN)", "測定画面表示ボタン", "ゲージポートNo."] -> [w1986] mode=indexing
                    tunnel: w1958 -> [w1985]
                    i -> [w1989]
                    # "④"
                    # "③"
                    n583 = local read "設定クラスタ_設定 10"() -> (w1984:T2)
                    n584 = case shown="0, デフォルト" w1989 {
                      tunnel: w1991 -> [w2000 w2009 w2018 w2027 w2036 w2045 w2054 w2063 w2072 w2081 w2090 w2099 w2108 w2117]
                      tunnel: [w1999 w2008 w2017 w2026 w2035 w2044 w2053 w2062 w2071 w2080 w2089 w2098 w2107 w2116] -> w1990
                      tunnel: w1985 -> [w1998 w2007 w2016 w2025 w2034 w2043 w2052 w2061 w2070 w2079 w2088 w2097 w2106 w2115]
                      tunnel: w1988 -> [w1997 w2006 w2015 w2024 w2033 w2042 w2051 w2060 w2069 w2078 w2087 w2096 w2105 w2114]
                      tunnel: [w1996 w2005 w2014 w2023 w2032 w2041 w2050 w2059 w2068 w2077 w2086 w2095 w2104 w2113] -> w1987
                      tunnel: w1986 -> [w1994 w2003 w2012 w2021 w2030 w2039 w2048 w2057 w2066 w2075 w2084 w2093 w2102 w2111]
                      tunnel: [w1993 w2001 w2010 w2019 w2028 w2037 w2046 w2055 w2064 w2073 w2082 w2091 w2100 w2109] -> w1983
                      tunnel: w1984 -> [w1992 w2002 w2011 w2020 w2029 w2038 w2047 w2056 w2065 w2074 w2083 w2092 w2101 w2110]
                      frame 0, Default {
                        n585 = call-poly <vilib>:"Read Key.vi"("section"=w1998, "error in (no error)"=w1997, "key"=w1994, "refnum"=w2000) -> ("error out"=w1996:errorcluster, "value"=w1995:string, "refnum out"=w1999:T9)  [unwired: 4 in, 1 out]
                        n586 = Bundle By Name(cluster=w1992, "規格"=w1995) -> (w1993:T2)
                      }
                      frame 1 {
                        n587 = call-poly <vilib>:"Read Key.vi"("section"=w2007, "error in (no error)"=w2006, "key"=w2003, "refnum"=w2009) -> ("error out"=w2005:errorcluster, "value"=w2004:string, "refnum out"=w2008:T9)  [unwired: 4 in, 1 out]
                        n588 = Bundle By Name(cluster=w2002, "規格上限"=w2004) -> (w2001:T2)
                      }
                      frame 2 {
                        n589 = call-poly <vilib>:"Read Key.vi"("section"=w2016, "error in (no error)"=w2015, "key"=w2012, "refnum"=w2018) -> ("error out"=w2014:errorcluster, "value"=w2013:string, "refnum out"=w2017:T9)  [unwired: 4 in, 1 out]
                        n590 = Bundle By Name(cluster=w2011, "規格下限"=w2013) -> (w2010:T2)
                      }
                      frame 3 {
                        n591 = call-poly <vilib>:"Read Key.vi"("section"=w2025, "error in (no error)"=w2024, "key"=w2021, "refnum"=w2027) -> ("error out"=w2023:errorcluster, "value"=w2022:i32, "refnum out"=w2026:T9)  [unwired: 4 in, 1 out]
                        n592 = Bundle By Name(cluster=w2020, "ポートNo."=w2022) -> (w2019:T2)
                      }
                      frame 4 {
                        n593 = call-poly <vilib>:"Read Key.vi"("section"=w2034, "error in (no error)"=w2033, "key"=w2030, "refnum"=w2036) -> ("error out"=w2032:errorcluster, "value"=w2031:i32, "refnum out"=w2035:T9)  [unwired: 4 in, 1 out]
                        n594 = Bundle By Name(cluster=w2029, "測定モード"=w2031) -> (w2028:T2)
                      }
                      frame 5 {
                        n595 = call-poly <vilib>:"Read Key.vi"("section"=w2043, "error in (no error)"=w2042, "key"=w2039, "refnum"=w2045) -> ("error out"=w2041:errorcluster, "value"=w2040:string, "refnum out"=w2044:T9)  [unwired: 4 in, 1 out]
                        n596 = Bundle By Name(cluster=w2038, "規格単位"=w2040) -> (w2037:T2)
                      }
                      frame 6 {
                        n597 = call-poly <vilib>:"Read Key.vi"("section"=w2052, "error in (no error)"=w2051, "key"=w2048, "refnum"=w2054) -> ("error out"=w2050:errorcluster, "value"=w2049:string, "refnum out"=w2053:T9)  [unwired: 4 in, 1 out]
                        n598 = Bundle By Name(cluster=w2047, "品質チェック項目"=w2049) -> (w2046:T2)
                      }
                      frame 7 {
                        n599 = call-poly <vilib>:"Read Key.vi"("section"=w2061, "error in (no error)"=w2060, "key"=w2057, "refnum"=w2063) -> ("error out"=w2059:errorcluster, "value"=w2058:i32, "refnum out"=w2062:T9)  [unwired: 4 in, 1 out]
                        n600 = Bundle By Name(cluster=w2056, "測定周期"=w2058) -> (w2055:T2)
                      }
                      frame 8 {
                        n601 = call-poly <vilib>:"Read Key.vi"("section"=w2070, "error in (no error)"=w2069, "key"=w2066, "refnum"=w2072) -> ("error out"=w2068:errorcluster, "value"=w2067:string, "refnum out"=w2071:T9)  [unwired: 4 in, 1 out]
                        n602 = Bundle By Name(cluster=w2065, "実測値MAX"=w2067) -> (w2064:T2)
                      }
                      frame 9 {
                        n603 = call-poly <vilib>:"Read Key.vi"("section"=w2079, "error in (no error)"=w2078, "key"=w2075, "refnum"=w2081) -> ("error out"=w2077:errorcluster, "value"=w2076:string, "refnum out"=w2080:T9)  [unwired: 4 in, 1 out]
                        n604 = Bundle By Name(cluster=w2074, "実測値MIN"=w2076) -> (w2073:T2)
                      }
                      frame 10 {
                        n605 = call-poly <vilib>:"Read Key.vi"("section"=w2088, "error in (no error)"=w2087, "key"=w2084, "refnum"=w2090) -> ("error out"=w2086:errorcluster, "value"=w2085:string, "refnum out"=w2089:T9)  [unwired: 4 in, 1 out]
                        n606 = Bundle By Name(cluster=w2083, "実測値(MAX)"=w2085) -> (w2082:T2)
                      }
                      frame 11 {
                        n607 = call-poly <vilib>:"Read Key.vi"("section"=w2097, "error in (no error)"=w2096, "key"=w2093, "refnum"=w2099) -> ("error out"=w2095:errorcluster, "value"=w2094:string, "refnum out"=w2098:T9)  [unwired: 4 in, 1 out]
                        n608 = Bundle By Name(cluster=w2092, "実測値(MIN)"=w2094) -> (w2091:T2)
                      }
                      frame 12 {
                        n609 = call-poly <vilib>:"Read Key.vi"("section"=w2106, "error in (no error)"=w2105, "key"=w2102, "refnum"=w2108) -> ("error out"=w2104:errorcluster, "value"=w2103:bool, "refnum out"=w2107:T9)  [unwired: 4 in, 1 out]
                        n610 = Bundle By Name(cluster=w2101, "測定画面表示ボタン"=w2103) -> (w2100:T2)
                      }
                      frame 13 {
                        n611 = call-poly <vilib>:"Read Key.vi"("section"=w2115, "error in (no error)"=w2114, "key"=w2111, "refnum"=w2117) -> ("error out"=w2113:errorcluster, "value"=w2112:string, "refnum out"=w2116:T9)  [unwired: 4 in, 1 out]
                        n612 = Bundle By Name(cluster=w2110, "ゲージポートNo"=w2112) -> (w2109:T2)
                      }
                    }
                    n613 = local write "設定クラスタ_設定 10"(w1983) -> ()
                  }
                  n614 = local read "使用ON/OFFボタン_設定 10"() -> (w1968:T5)
                  n615 = call-poly <vilib>:"Read Key.vi"("section"=w1958, "error in (no error)"=w1979, "key"="使用ON/OFF", "refnum"=w1981) -> ("error out"=w1961:errorcluster, "value"=w1970:bool, "refnum out"=w1962:T9)  [unwired: 4 in, 1 out]
                  n616 = Bundle By Name(cluster=w1968, "使用ON/OFF"=w1970) -> (w1967:T5)
                  n617 = local write "使用ON/OFFボタン_設定 10"(w1967) -> ()
                  n618 = local read "CSV項目名 10"() -> (w1965:T1)
                  n619 = call-poly <vilib>:"Read Key.vi"("section"=w1958, "error in (no error)"=w1961, "key"="CSVヘッダー名", "refnum"=w1962) -> ("error out"=w1960:errorcluster, "value"=w1963:string, "refnum out"=w1959:T9)  [unwired: 4 in, 1 out]
                  n620 = Bundle By Name(cluster=w1965, "CSV項目名"=w1963) -> (w1966:T1)
                  n621 = local write "CSV項目名 10"(w1966) -> ()
                }
                frame #1 {
                  # "⑮"
                  # "⑭"
                  # "⑩"
                  # "⑨"
                  # "測定モード設定時の動作"
                  n622 = local read "設定クラスタ_設定 10"() -> (w2122:T2)
                  n623 = Unbundle By Name(w2122) -> ("測定モード"=w2121:u16)
                  n624 = case shown="0, デフォルト" w2121 {
                    tunnel: w2122 -> [w2131 w2138 w2146]
                    tunnel: [w2130 w2137 w2145] -> w2120
                    tunnel: [T8."Enabled" ("無効") T8."Enabled" ("無効") T8."Disabled and Grayed Out" ("無効")] -> w2119
                    tunnel: [T8."Enabled" ("無効") T8."Enabled" ("無効") T8."Disabled and Grayed Out" ("無効")] -> w2118
                    frame 1 {
                      w2127 = ""
                      # "連続測定モードの場合MAXとMINを表示する"
                      n625 = Bundle By Name(cluster=w2131, "実測値MAX"="MAX", "実測値MIN"="MIN", "実測値(MAX)"=w2127, "実測値(MIN)"=w2127) -> (w2130:T2)
                    }
                    frame 2 {
                      w2134 = ""
                      # "多点測定モードの場合MAXとMINを表示する"
                      n626 = Bundle By Name(cluster=w2138, "実測値MAX"="MAX", "実測値MIN"="MIN", "実測値(MAX)"=w2134, "実測値(MIN)"=w2134) -> (w2137:T2)
                    }
                    frame 0, Default {
                      n627 = Bundle By Name(cluster=w2146, "実測値(MAX)"="", "実測値MAX"="値", "実測値(MIN)"="", "実測値MIN"="") -> (w2145:T2)
                    }
                  }
                  n628 = local write "設定クラスタ_設定 10"(w2120) -> ()
                  n629 = property on="実測値MIN" class="Str"("DisabledEnum"=w2119) -> ()  [unwired: 2 in, 2 out]
                  n630 = property on="実測値(MIN)" class="Str"("DisabledEnum"=w2118) -> ()  [unwired: 2 in, 2 out]
                }
              }
              n631 = Replace Array Subset(array=w1952, new element=w1949, index=9) -> (w1953:T2[])
            }
            frame 10 {
              # "⑯"
              # "⑪"
              n632 = flat-sequence {
                tunnel: w2156 -> [w2172]
                tunnel: w2155 -> [w2173]
                tunnel: [w2158] -> w2150
                tunnel: [w2159] -> w2149
                tunnel: [w2323] -> w2154
                tunnel: [w2322] -> w2153
                tunnel: [w2321] -> w2148
                tunnel: w2150 -> [w2322]
                tunnel: w2149 -> [w2323]
                frame #0 {
                  w2157 = "設定11"
                  # "⑧"
                  # "⑦"
                  # "⑬"
                  # "⑫"
                  # "⑥"
                  # "⑤"
                  # "②"
                  # "①"
                  # "複製した時に変更する項目\n①②③④⑤⑥⑦⑧⑨⑩\nローカル変数\n⑪\n指標値\n⑫⑬\nセレクション\n⑭⑮\nプロパティノード設定直し\n⑯\n複製したケースのTrue定数を削除"
                  # "setting.iniファイルからの設定項目の読み取り"
                  n633 = local read "No設定クラスタ_設定 11"() -> (w2175:T7)
                  n634 = call-poly <vilib>:"Read Key.vi"("section"="No11.", "error in (no error)"=w2172, "key"="No.", "refnum"=w2173) -> ("error out"=w2179:errorcluster, "value"=w2171:i32, "refnum out"=w2181:T9)  [unwired: 4 in, 1 out]
                  n635 = Bundle By Name(cluster=w2175, "No."=w2171) -> (w2174:T7)
                  n636 = local write "No設定クラスタ_設定 11"(w2174) -> ()
                  n637 = for {
                    shift-right: [w2189] -> w2180
                    shift-left: w2181 -> [w2190]
                    shift-right: [w2186] -> w2178
                    shift-left: w2179 -> [w2187]
                    tunnel: string[] ["規格", "規格上限", "規格下限", "ポートNo.", "測定モード", "規格単位", "品質チェック項目", "測定周期", "実測MAX", "実測MIN", "実測(MAX)", "実測(MIN)", "測定画面表示ボタン", "ゲージポートNo."] -> [w2185] mode=indexing
                    tunnel: w2157 -> [w2184]
                    i -> [w2188]
                    # "④"
                    # "③"
                    n638 = local read "設定クラスタ_設定 11"() -> (w2183:T2)
                    n639 = case shown="0, デフォルト" w2188 {
                      tunnel: w2190 -> [w2199 w2208 w2217 w2226 w2235 w2244 w2253 w2262 w2271 w2280 w2289 w2298 w2307 w2316]
                      tunnel: [w2198 w2207 w2216 w2225 w2234 w2243 w2252 w2261 w2270 w2279 w2288 w2297 w2306 w2315] -> w2189
                      tunnel: w2184 -> [w2197 w2206 w2215 w2224 w2233 w2242 w2251 w2260 w2269 w2278 w2287 w2296 w2305 w2314]
                      tunnel: w2187 -> [w2196 w2205 w2214 w2223 w2232 w2241 w2250 w2259 w2268 w2277 w2286 w2295 w2304 w2313]
                      tunnel: [w2195 w2204 w2213 w2222 w2231 w2240 w2249 w2258 w2267 w2276 w2285 w2294 w2303 w2312] -> w2186
                      tunnel: w2185 -> [w2193 w2202 w2211 w2220 w2229 w2238 w2247 w2256 w2265 w2274 w2283 w2292 w2301 w2310]
                      tunnel: [w2192 w2200 w2209 w2218 w2227 w2236 w2245 w2254 w2263 w2272 w2281 w2290 w2299 w2308] -> w2182
                      tunnel: w2183 -> [w2191 w2201 w2210 w2219 w2228 w2237 w2246 w2255 w2264 w2273 w2282 w2291 w2300 w2309]
                      frame 0, Default {
                        n640 = call-poly <vilib>:"Read Key.vi"("section"=w2197, "error in (no error)"=w2196, "key"=w2193, "refnum"=w2199) -> ("error out"=w2195:errorcluster, "value"=w2194:string, "refnum out"=w2198:T9)  [unwired: 4 in, 1 out]
                        n641 = Bundle By Name(cluster=w2191, "規格"=w2194) -> (w2192:T2)
                      }
                      frame 1 {
                        n642 = call-poly <vilib>:"Read Key.vi"("section"=w2206, "error in (no error)"=w2205, "key"=w2202, "refnum"=w2208) -> ("error out"=w2204:errorcluster, "value"=w2203:string, "refnum out"=w2207:T9)  [unwired: 4 in, 1 out]
                        n643 = Bundle By Name(cluster=w2201, "規格上限"=w2203) -> (w2200:T2)
                      }
                      frame 2 {
                        n644 = call-poly <vilib>:"Read Key.vi"("section"=w2215, "error in (no error)"=w2214, "key"=w2211, "refnum"=w2217) -> ("error out"=w2213:errorcluster, "value"=w2212:string, "refnum out"=w2216:T9)  [unwired: 4 in, 1 out]
                        n645 = Bundle By Name(cluster=w2210, "規格下限"=w2212) -> (w2209:T2)
                      }
                      frame 3 {
                        n646 = call-poly <vilib>:"Read Key.vi"("section"=w2224, "error in (no error)"=w2223, "key"=w2220, "refnum"=w2226) -> ("error out"=w2222:errorcluster, "value"=w2221:i32, "refnum out"=w2225:T9)  [unwired: 4 in, 1 out]
                        n647 = Bundle By Name(cluster=w2219, "ポートNo."=w2221) -> (w2218:T2)
                      }
                      frame 4 {
                        n648 = call-poly <vilib>:"Read Key.vi"("section"=w2233, "error in (no error)"=w2232, "key"=w2229, "refnum"=w2235) -> ("error out"=w2231:errorcluster, "value"=w2230:i32, "refnum out"=w2234:T9)  [unwired: 4 in, 1 out]
                        n649 = Bundle By Name(cluster=w2228, "測定モード"=w2230) -> (w2227:T2)
                      }
                      frame 5 {
                        n650 = call-poly <vilib>:"Read Key.vi"("section"=w2242, "error in (no error)"=w2241, "key"=w2238, "refnum"=w2244) -> ("error out"=w2240:errorcluster, "value"=w2239:string, "refnum out"=w2243:T9)  [unwired: 4 in, 1 out]
                        n651 = Bundle By Name(cluster=w2237, "規格単位"=w2239) -> (w2236:T2)
                      }
                      frame 6 {
                        n652 = call-poly <vilib>:"Read Key.vi"("section"=w2251, "error in (no error)"=w2250, "key"=w2247, "refnum"=w2253) -> ("error out"=w2249:errorcluster, "value"=w2248:string, "refnum out"=w2252:T9)  [unwired: 4 in, 1 out]
                        n653 = Bundle By Name(cluster=w2246, "品質チェック項目"=w2248) -> (w2245:T2)
                      }
                      frame 7 {
                        n654 = call-poly <vilib>:"Read Key.vi"("section"=w2260, "error in (no error)"=w2259, "key"=w2256, "refnum"=w2262) -> ("error out"=w2258:errorcluster, "value"=w2257:i32, "refnum out"=w2261:T9)  [unwired: 4 in, 1 out]
                        n655 = Bundle By Name(cluster=w2255, "測定周期"=w2257) -> (w2254:T2)
                      }
                      frame 8 {
                        n656 = call-poly <vilib>:"Read Key.vi"("section"=w2269, "error in (no error)"=w2268, "key"=w2265, "refnum"=w2271) -> ("error out"=w2267:errorcluster, "value"=w2266:string, "refnum out"=w2270:T9)  [unwired: 4 in, 1 out]
                        n657 = Bundle By Name(cluster=w2264, "実測値MAX"=w2266) -> (w2263:T2)
                      }
                      frame 9 {
                        n658 = call-poly <vilib>:"Read Key.vi"("section"=w2278, "error in (no error)"=w2277, "key"=w2274, "refnum"=w2280) -> ("error out"=w2276:errorcluster, "value"=w2275:string, "refnum out"=w2279:T9)  [unwired: 4 in, 1 out]
                        n659 = Bundle By Name(cluster=w2273, "実測値MIN"=w2275) -> (w2272:T2)
                      }
                      frame 10 {
                        n660 = call-poly <vilib>:"Read Key.vi"("section"=w2287, "error in (no error)"=w2286, "key"=w2283, "refnum"=w2289) -> ("error out"=w2285:errorcluster, "value"=w2284:string, "refnum out"=w2288:T9)  [unwired: 4 in, 1 out]
                        n661 = Bundle By Name(cluster=w2282, "実測値(MAX)"=w2284) -> (w2281:T2)
                      }
                      frame 11 {
                        n662 = call-poly <vilib>:"Read Key.vi"("section"=w2296, "error in (no error)"=w2295, "key"=w2292, "refnum"=w2298) -> ("error out"=w2294:errorcluster, "value"=w2293:string, "refnum out"=w2297:T9)  [unwired: 4 in, 1 out]
                        n663 = Bundle By Name(cluster=w2291, "実測値(MIN)"=w2293) -> (w2290:T2)
                      }
                      frame 12 {
                        n664 = call-poly <vilib>:"Read Key.vi"("section"=w2305, "error in (no error)"=w2304, "key"=w2301, "refnum"=w2307) -> ("error out"=w2303:errorcluster, "value"=w2302:bool, "refnum out"=w2306:T9)  [unwired: 4 in, 1 out]
                        n665 = Bundle By Name(cluster=w2300, "測定画面表示ボタン"=w2302) -> (w2299:T2)
                      }
                      frame 13 {
                        n666 = call-poly <vilib>:"Read Key.vi"("section"=w2314, "error in (no error)"=w2313, "key"=w2310, "refnum"=w2316) -> ("error out"=w2312:errorcluster, "value"=w2311:string, "refnum out"=w2315:T9)  [unwired: 4 in, 1 out]
                        n667 = Bundle By Name(cluster=w2309, "ゲージポートNo"=w2311) -> (w2308:T2)
                      }
                    }
                    n668 = local write "設定クラスタ_設定 11"(w2182) -> ()
                  }
                  n669 = local read "使用ON/OFFボタン_設定 11"() -> (w2167:T5)
                  n670 = call-poly <vilib>:"Read Key.vi"("section"=w2157, "error in (no error)"=w2178, "key"="使用ON/OFF", "refnum"=w2180) -> ("error out"=w2160:errorcluster, "value"=w2169:bool, "refnum out"=w2161:T9)  [unwired: 4 in, 1 out]
                  n671 = Bundle By Name(cluster=w2167, "使用ON/OFF"=w2169) -> (w2166:T5)
                  n672 = local write "使用ON/OFFボタン_設定 11"(w2166) -> ()
                  n673 = local read "CSV項目名 11"() -> (w2164:T1)
                  n674 = call-poly <vilib>:"Read Key.vi"("section"=w2157, "error in (no error)"=w2160, "key"="CSVヘッダー名", "refnum"=w2161) -> ("error out"=w2159:errorcluster, "value"=w2162:string, "refnum out"=w2158:T9)  [unwired: 4 in, 1 out]
                  n675 = Bundle By Name(cluster=w2164, "CSV項目名"=w2162) -> (w2165:T1)
                  n676 = local write "CSV項目名 11"(w2165) -> ()
                }
                frame #1 {
                  # "⑮"
                  # "⑭"
                  # "⑩"
                  # "⑨"
                  # "測定モード設定時の動作"
                  n677 = local read "設定クラスタ_設定 11"() -> (w2321:T2)
                  n678 = Unbundle By Name(w2321) -> ("測定モード"=w2320:u16)
                  n679 = case shown="0, デフォルト" w2320 {
                    tunnel: w2321 -> [w2330 w2337 w2345]
                    tunnel: [w2329 w2336 w2344] -> w2319
                    tunnel: [T8."Enabled" ("無効") T8."Enabled" ("無効") T8."Disabled and Grayed Out" ("無効")] -> w2318
                    tunnel: [T8."Enabled" ("無効") T8."Enabled" ("無効") T8."Disabled and Grayed Out" ("無効")] -> w2317
                    frame 1 {
                      w2326 = ""
                      # "連続測定モードの場合MAXとMINを表示する"
                      n680 = Bundle By Name(cluster=w2330, "実測値MAX"="MAX", "実測値MIN"="MIN", "実測値(MAX)"=w2326, "実測値(MIN)"=w2326) -> (w2329:T2)
                    }
                    frame 2 {
                      w2333 = ""
                      # "多点測定モードの場合MAXとMINを表示する"
                      n681 = Bundle By Name(cluster=w2337, "実測値MAX"="MAX", "実測値MIN"="MIN", "実測値(MAX)"=w2333, "実測値(MIN)"=w2333) -> (w2336:T2)
                    }
                    frame 0, Default {
                      n682 = Bundle By Name(cluster=w2345, "実測値(MAX)"="", "実測値MAX"="値", "実測値(MIN)"="", "実測値MIN"="") -> (w2344:T2)
                    }
                  }
                  n683 = local write "設定クラスタ_設定 11"(w2319) -> ()
                  n684 = property on="実測値MIN" class="Str"("DisabledEnum"=w2318) -> ()  [unwired: 2 in, 2 out]
                  n685 = property on="実測値(MIN)" class="Str"("DisabledEnum"=w2317) -> ()  [unwired: 2 in, 2 out]
                }
              }
              n686 = Replace Array Subset(array=w2151, new element=w2148, index=10) -> (w2152:T2[])
            }
            frame 11 {
              # "⑯"
              # "⑪"
              n687 = flat-sequence {
                tunnel: w2355 -> [w2371]
                tunnel: w2354 -> [w2372]
                tunnel: [w2357] -> w2349
                tunnel: [w2358] -> w2348
                tunnel: [w2522] -> w2353
                tunnel: [w2521] -> w2352
                tunnel: [w2520] -> w2347
                tunnel: w2349 -> [w2521]
                tunnel: w2348 -> [w2522]
                frame #0 {
                  w2356 = "設定12"
                  # "⑧"
                  # "⑦"
                  # "⑬"
                  # "⑫"
                  # "⑥"
                  # "⑤"
                  # "②"
                  # "①"
                  # "複製した時に変更する項目\n①②③④⑤⑥⑦⑧⑨⑩\nローカル変数\n⑪\n指標値\n⑫⑬\nセレクション\n⑭⑮\nプロパティノード設定直し\n⑯\n複製したケースのTrue定数を削除"
                  # "setting.iniファイルからの設定項目の読み取り"
                  n688 = local read "No設定クラスタ_設定 12"() -> (w2374:T7)
                  n689 = call-poly <vilib>:"Read Key.vi"("section"="No12.", "error in (no error)"=w2371, "key"="No.", "refnum"=w2372) -> ("error out"=w2378:errorcluster, "value"=w2370:i32, "refnum out"=w2380:T9)  [unwired: 4 in, 1 out]
                  n690 = Bundle By Name(cluster=w2374, "No."=w2370) -> (w2373:T7)
                  n691 = local write "No設定クラスタ_設定 12"(w2373) -> ()
                  n692 = for {
                    shift-right: [w2388] -> w2379
                    shift-left: w2380 -> [w2389]
                    shift-right: [w2385] -> w2377
                    shift-left: w2378 -> [w2386]
                    tunnel: string[] ["規格", "規格上限", "規格下限", "ポートNo.", "測定モード", "規格単位", "品質チェック項目", "測定周期", "実測MAX", "実測MIN", "実測(MAX)", "実測(MIN)", "測定画面表示ボタン", "ゲージポートNo."] -> [w2384] mode=indexing
                    tunnel: w2356 -> [w2383]
                    i -> [w2387]
                    # "④"
                    # "③"
                    n693 = local read "設定クラスタ_設定 12"() -> (w2382:T2)
                    n694 = case shown="0, デフォルト" w2387 {
                      tunnel: w2389 -> [w2398 w2407 w2416 w2425 w2434 w2443 w2452 w2461 w2470 w2479 w2488 w2497 w2506 w2515]
                      tunnel: [w2397 w2406 w2415 w2424 w2433 w2442 w2451 w2460 w2469 w2478 w2487 w2496 w2505 w2514] -> w2388
                      tunnel: w2383 -> [w2396 w2405 w2414 w2423 w2432 w2441 w2450 w2459 w2468 w2477 w2486 w2495 w2504 w2513]
                      tunnel: w2386 -> [w2395 w2404 w2413 w2422 w2431 w2440 w2449 w2458 w2467 w2476 w2485 w2494 w2503 w2512]
                      tunnel: [w2394 w2403 w2412 w2421 w2430 w2439 w2448 w2457 w2466 w2475 w2484 w2493 w2502 w2511] -> w2385
                      tunnel: w2384 -> [w2392 w2401 w2410 w2419 w2428 w2437 w2446 w2455 w2464 w2473 w2482 w2491 w2500 w2509]
                      tunnel: [w2391 w2399 w2408 w2417 w2426 w2435 w2444 w2453 w2462 w2471 w2480 w2489 w2498 w2507] -> w2381
                      tunnel: w2382 -> [w2390 w2400 w2409 w2418 w2427 w2436 w2445 w2454 w2463 w2472 w2481 w2490 w2499 w2508]
                      frame 0, Default {
                        n695 = call-poly <vilib>:"Read Key.vi"("section"=w2396, "error in (no error)"=w2395, "key"=w2392, "refnum"=w2398) -> ("error out"=w2394:errorcluster, "value"=w2393:string, "refnum out"=w2397:T9)  [unwired: 4 in, 1 out]
                        n696 = Bundle By Name(cluster=w2390, "規格"=w2393) -> (w2391:T2)
                      }
                      frame 1 {
                        n697 = call-poly <vilib>:"Read Key.vi"("section"=w2405, "error in (no error)"=w2404, "key"=w2401, "refnum"=w2407) -> ("error out"=w2403:errorcluster, "value"=w2402:string, "refnum out"=w2406:T9)  [unwired: 4 in, 1 out]
                        n698 = Bundle By Name(cluster=w2400, "規格上限"=w2402) -> (w2399:T2)
                      }
                      frame 2 {
                        n699 = call-poly <vilib>:"Read Key.vi"("section"=w2414, "error in (no error)"=w2413, "key"=w2410, "refnum"=w2416) -> ("error out"=w2412:errorcluster, "value"=w2411:string, "refnum out"=w2415:T9)  [unwired: 4 in, 1 out]
                        n700 = Bundle By Name(cluster=w2409, "規格下限"=w2411) -> (w2408:T2)
                      }
                      frame 3 {
                        n701 = call-poly <vilib>:"Read Key.vi"("section"=w2423, "error in (no error)"=w2422, "key"=w2419, "refnum"=w2425) -> ("error out"=w2421:errorcluster, "value"=w2420:i32, "refnum out"=w2424:T9)  [unwired: 4 in, 1 out]
                        n702 = Bundle By Name(cluster=w2418, "ポートNo."=w2420) -> (w2417:T2)
                      }
                      frame 4 {
                        n703 = call-poly <vilib>:"Read Key.vi"("section"=w2432, "error in (no error)"=w2431, "key"=w2428, "refnum"=w2434) -> ("error out"=w2430:errorcluster, "value"=w2429:i32, "refnum out"=w2433:T9)  [unwired: 4 in, 1 out]
                        n704 = Bundle By Name(cluster=w2427, "測定モード"=w2429) -> (w2426:T2)
                      }
                      frame 5 {
                        n705 = call-poly <vilib>:"Read Key.vi"("section"=w2441, "error in (no error)"=w2440, "key"=w2437, "refnum"=w2443) -> ("error out"=w2439:errorcluster, "value"=w2438:string, "refnum out"=w2442:T9)  [unwired: 4 in, 1 out]
                        n706 = Bundle By Name(cluster=w2436, "規格単位"=w2438) -> (w2435:T2)
                      }
                      frame 6 {
                        n707 = call-poly <vilib>:"Read Key.vi"("section"=w2450, "error in (no error)"=w2449, "key"=w2446, "refnum"=w2452) -> ("error out"=w2448:errorcluster, "value"=w2447:string, "refnum out"=w2451:T9)  [unwired: 4 in, 1 out]
                        n708 = Bundle By Name(cluster=w2445, "品質チェック項目"=w2447) -> (w2444:T2)
                      }
                      frame 7 {
                        n709 = call-poly <vilib>:"Read Key.vi"("section"=w2459, "error in (no error)"=w2458, "key"=w2455, "refnum"=w2461) -> ("error out"=w2457:errorcluster, "value"=w2456:i32, "refnum out"=w2460:T9)  [unwired: 4 in, 1 out]
                        n710 = Bundle By Name(cluster=w2454, "測定周期"=w2456) -> (w2453:T2)
                      }
                      frame 8 {
                        n711 = call-poly <vilib>:"Read Key.vi"("section"=w2468, "error in (no error)"=w2467, "key"=w2464, "refnum"=w2470) -> ("error out"=w2466:errorcluster, "value"=w2465:string, "refnum out"=w2469:T9)  [unwired: 4 in, 1 out]
                        n712 = Bundle By Name(cluster=w2463, "実測値MAX"=w2465) -> (w2462:T2)
                      }
                      frame 9 {
                        n713 = call-poly <vilib>:"Read Key.vi"("section"=w2477, "error in (no error)"=w2476, "key"=w2473, "refnum"=w2479) -> ("error out"=w2475:errorcluster, "value"=w2474:string, "refnum out"=w2478:T9)  [unwired: 4 in, 1 out]
                        n714 = Bundle By Name(cluster=w2472, "実測値MIN"=w2474) -> (w2471:T2)
                      }
                      frame 10 {
                        n715 = call-poly <vilib>:"Read Key.vi"("section"=w2486, "error in (no error)"=w2485, "key"=w2482, "refnum"=w2488) -> ("error out"=w2484:errorcluster, "value"=w2483:string, "refnum out"=w2487:T9)  [unwired: 4 in, 1 out]
                        n716 = Bundle By Name(cluster=w2481, "実測値(MAX)"=w2483) -> (w2480:T2)
                      }
                      frame 11 {
                        n717 = call-poly <vilib>:"Read Key.vi"("section"=w2495, "error in (no error)"=w2494, "key"=w2491, "refnum"=w2497) -> ("error out"=w2493:errorcluster, "value"=w2492:string, "refnum out"=w2496:T9)  [unwired: 4 in, 1 out]
                        n718 = Bundle By Name(cluster=w2490, "実測値(MIN)"=w2492) -> (w2489:T2)
                      }
                      frame 12 {
                        n719 = call-poly <vilib>:"Read Key.vi"("section"=w2504, "error in (no error)"=w2503, "key"=w2500, "refnum"=w2506) -> ("error out"=w2502:errorcluster, "value"=w2501:bool, "refnum out"=w2505:T9)  [unwired: 4 in, 1 out]
                        n720 = Bundle By Name(cluster=w2499, "測定画面表示ボタン"=w2501) -> (w2498:T2)
                      }
                      frame 13 {
                        n721 = call-poly <vilib>:"Read Key.vi"("section"=w2513, "error in (no error)"=w2512, "key"=w2509, "refnum"=w2515) -> ("error out"=w2511:errorcluster, "value"=w2510:string, "refnum out"=w2514:T9)  [unwired: 4 in, 1 out]
                        n722 = Bundle By Name(cluster=w2508, "ゲージポートNo"=w2510) -> (w2507:T2)
                      }
                    }
                    n723 = local write "設定クラスタ_設定 12"(w2381) -> ()
                  }
                  n724 = local read "使用ON/OFFボタン_設定 12"() -> (w2366:T5)
                  n725 = call-poly <vilib>:"Read Key.vi"("section"=w2356, "error in (no error)"=w2377, "key"="使用ON/OFF", "refnum"=w2379) -> ("error out"=w2359:errorcluster, "value"=w2368:bool, "refnum out"=w2360:T9)  [unwired: 4 in, 1 out]
                  n726 = Bundle By Name(cluster=w2366, "使用ON/OFF"=w2368) -> (w2365:T5)
                  n727 = local write "使用ON/OFFボタン_設定 12"(w2365) -> ()
                  n728 = local read "CSV項目名 12"() -> (w2363:T1)
                  n729 = call-poly <vilib>:"Read Key.vi"("section"=w2356, "error in (no error)"=w2359, "key"="CSVヘッダー名", "refnum"=w2360) -> ("error out"=w2358:errorcluster, "value"=w2361:string, "refnum out"=w2357:T9)  [unwired: 4 in, 1 out]
                  n730 = Bundle By Name(cluster=w2363, "CSV項目名"=w2361) -> (w2364:T1)
                  n731 = local write "CSV項目名 12"(w2364) -> ()
                }
                frame #1 {
                  # "⑮"
                  # "⑭"
                  # "⑩"
                  # "⑨"
                  # "測定モード設定時の動作"
                  n732 = local read "設定クラスタ_設定 12"() -> (w2520:T2)
                  n733 = Unbundle By Name(w2520) -> ("測定モード"=w2519:u16)
                  n734 = case shown="0, デフォルト" w2519 {
                    tunnel: w2520 -> [w2529 w2536 w2544]
                    tunnel: [w2528 w2535 w2543] -> w2518
                    tunnel: [T8."Enabled" ("無効") T8."Enabled" ("無効") T8."Disabled and Grayed Out" ("無効")] -> w2517
                    tunnel: [T8."Enabled" ("無効") T8."Enabled" ("無効") T8."Disabled and Grayed Out" ("無効")] -> w2516
                    frame 1 {
                      w2525 = ""
                      # "連続測定モードの場合MAXとMINを表示する"
                      n735 = Bundle By Name(cluster=w2529, "実測値MAX"="MAX", "実測値MIN"="MIN", "実測値(MAX)"=w2525, "実測値(MIN)"=w2525) -> (w2528:T2)
                    }
                    frame 2 {
                      w2532 = ""
                      # "多点測定モードの場合MAXとMINを表示する"
                      n736 = Bundle By Name(cluster=w2536, "実測値MAX"="MAX", "実測値MIN"="MIN", "実測値(MAX)"=w2532, "実測値(MIN)"=w2532) -> (w2535:T2)
                    }
                    frame 0, Default {
                      n737 = Bundle By Name(cluster=w2544, "実測値(MAX)"="", "実測値MAX"="値", "実測値(MIN)"="", "実測値MIN"="") -> (w2543:T2)
                    }
                  }
                  n738 = local write "設定クラスタ_設定 12"(w2518) -> ()
                  n739 = property on="実測値MIN" class="Str"("DisabledEnum"=w2517) -> ()  [unwired: 2 in, 2 out]
                  n740 = property on="実測値(MIN)" class="Str"("DisabledEnum"=w2516) -> ()  [unwired: 2 in, 2 out]
                }
              }
              n741 = Replace Array Subset(array=w2350, new element=w2347, index=11) -> (w2351:T2[])
            }
            frame 12 {
            }
          }
          n742 = call <vilib>:"Close Config Data.vi"("error in (no error)"=w32, "refnum"=w31) -> ("error out"=→"iniRエラーout 2":errorcluster)  [unwired: 1 in, 8 out]
        }
      }
      frame "登録" {
        n743 = while {
          tunnel: w2548 -> [w2552]
          tunnel: [w2551] -> w2547
          i -> [w2559]
          stop <- w2550 stop-if-true
          n744 = local read "iniフォルダパス取得"() -> (w2558:path)
          n745 = Build Path "パス作成"(base path=w2558, name or relative path=path "setting1.ini") -> (appended path=w2557:path)
          n746 = call <vilib>:"Open Config Data.vi"("error in (no error)"="error in (no error)", "configuration file path"=w2557) -> ("error out"=w2553:errorcluster, "refnum"=w2554:T9)  [unwired: 1 in, 7 out]
          n747 = case shown="0, デフォルト" w2559 {
            tunnel: w2554 -> [w2563 w2837 w2855 w2873 w2891 w2909 w2927 w2945 w2963 w2981 w2999 w3017 _]
            tunnel: w2553 -> [w2562 w2836 w2854 w2872 w2890 w2908 w2926 w2944 w2962 w2980 w2998 w3016 _]
            tunnel: w2552 -> [w2561 w2835 w2853 w2871 w2889 w2907 w2925 w2943 w2961 w2979 w2997 w3015 _]
            tunnel: [w2560 w2834 w2852 w2870 w2888 w2906 w2924 w2942 w2960 w2978 w2996 w3014 _] -> w2551
            tunnel: [_ _ _ _ _ _ _ _ _ _ _ _ TRUE] -> w2550
            frame 0, Default {
              n748 = while {
                tunnel: w2563 -> [w2567]
                tunnel: w2562 -> [w2566]
                tunnel: w2561 -> [w2565]
                tunnel: [w2564] -> w2560
                stop <- w2568 stop-if-true
                n749 = flat-sequence {
                  tunnel: [TRUE] -> w2568
                  tunnel: w2567 -> [w2573]
                  tunnel: w2566 -> [w2572]
                  tunnel: w2565 -> [w2570]
                  tunnel: [w2569] -> w2564
                  frame #0 {
                    # "０,デフォルトは項目以外に品番等の登録も行っている為、\n複製不可"
                    # "登録ボタンが押された時に動作"
                    n750 = flat-sequence {
                      tunnel: [w2581] -> w2576
                      tunnel: [w2580] -> w2575
                      tunnel: w2573 -> [w2579]
                      tunnel: w2572 -> [w2578]
                      tunnel: [w2577] -> w2571
                      tunnel: w2570 -> [w2577]
                      tunnel: w2576 -> [w2639]
                      tunnel: w2575 -> [w2640]
                      tunnel: w2571 -> [w2638]
                      tunnel: [w2638] -> w2569
                      frame #0 {
                        # "品番、品名、測定周期、CSV保存名のiniファイル登録"
                        n751 = local read "品番・品名クラスタ_設定"() -> (w2584:T3)
                        n752 = for {
                          tunnel: string[] ["品番前", "品番後", "品名", "測定周期", "CSV保存名", "書込周期"] -> [w2591] mode=indexing
                          tunnel: w2584 -> [w2590]
                          shift-right: [w2589] -> w2580
                          shift-left: w2579 -> [w2588]
                          tunnel: "品番・品名" -> [w2587]
                          shift-right: [w2585] -> w2581
                          shift-left: w2578 -> [w2586]
                          i -> [w2592]
                          n753 = case shown="4" w2592 {
                            tunnel: w2591 -> [w2599 w2607 w2615 w2623 w2630 w2637]
                            tunnel: w2590 -> [w2598 w2606 w2614 _ _ _]
                            tunnel: [w2597 w2605 w2612 w2621 w2628 w2635] -> w2589
                            tunnel: w2588 -> [w2596 w2604 w2613 w2622 w2629 w2636]
                            tunnel: w2587 -> [w2595 w2603 w2611 w2620 w2627 w2634]
                            tunnel: w2586 -> [w2594 w2602 w2610 w2619 w2626 w2633]
                            tunnel: [w2593 w2601 w2609 w2618 w2625 w2632] -> w2585
                            frame 0, Default {
                              n754 = Unbundle By Name(w2598) -> ("品番前"=w2600:string)
                              n755 = call-poly <vilib>:"Write Key.vi"("section"=w2595, "error in (no error)"=w2594, "value"=w2600, "key"=w2599, "refnum"=w2596) -> ("error out"=w2593:errorcluster, "refnum out"=w2597:T9)  [unwired: 1 in, 4 out]
                            }
                            frame 1 {
                              n756 = Unbundle By Name(w2606) -> ("品番後"=w2608:string)
                              n757 = call-poly <vilib>:"Write Key.vi"("section"=w2603, "error in (no error)"=w2602, "value"=w2608, "key"=w2607, "refnum"=w2604) -> ("error out"=w2601:errorcluster, "refnum out"=w2605:T9)  [unwired: 1 in, 4 out]
                            }
                            frame 2 {
                              n758 = Unbundle By Name(w2614) -> ("品名"=w2616:string)
                              n759 = call-poly <vilib>:"Write Key.vi"("section"=w2611, "error in (no error)"=w2610, "value"=w2616, "key"=w2615, "refnum"=w2613) -> ("error out"=w2609:errorcluster, "refnum out"=w2612:T9)  [unwired: 1 in, 4 out]
                            }
                            frame 3 {
                              n760 = local read "測定周期/ms"() -> (w2617:dbl)
                              n761 = call-poly <vilib>:"Write Key.vi"("section"=w2620, "error in (no error)"=w2619, "value"=w2617, "key"=w2623, "refnum"=w2622) -> ("error out"=w2618:errorcluster, "refnum out"=w2621:T9)  [unwired: 3 in, 2 out]
                            }
                            frame 4 {
                              n762 = local read "② CSV保存名"() -> (w2624:string)
                              n763 = call-poly <vilib>:"Write Key.vi"("section"=w2627, "error in (no error)"=w2626, "value"=w2624, "key"=w2630, "refnum"=w2629) -> ("error out"=w2625:errorcluster, "refnum out"=w2628:T9)  [unwired: 1 in, 4 out]
                            }
                            frame 5 {
                              n764 = local read "書込周期/ms"() -> (w2631:dbl)
                              n765 = call-poly <vilib>:"Write Key.vi"("section"=w2634, "error in (no error)"=w2633, "value"=w2631, "key"=w2637, "refnum"=w2636) -> ("error out"=w2632:errorcluster, "refnum out"=w2635:T9)  [unwired: 3 in, 2 out]
                            }
                          }
                        }
                      }
                      frame #1 {
                        n766 = for {
                          N: 1 -> [_]
                          tunnel: w2640 -> [w2646]
                          tunnel: w2639 -> [w2645]
                          n767 = local read "No設定クラスタ_設定1"() -> (w2647:T7)
                          n768 = for {
                            shift-right: [w2652] -> w2643
                            shift-left: w2646 -> [w2653]
                            tunnel: w2647 -> [w2656]
                            tunnel: string[] ["No."] -> [w2655] mode=indexing
                            tunnel: "No." -> [w2654]
                            shift-right: [w2650] -> w2642
                            shift-left: w2645 -> [w2651]
                            i -> [w2657]
                            n769 = case shown="0, デフォルト" w2657 {
                              tunnel: w2656 -> [w2676]
                              tunnel: w2655 -> [w2674]
                              tunnel: w2654 -> [w2673]
                              tunnel: w2653 -> [w2672]
                              tunnel: [w2660] -> w2652
                              tunnel: w2651 -> [w2666]
                              tunnel: [w2659] -> w2650
                              frame 0, Default {
                                w2662 = "設定"
                                n770 = local read "設定クラスタ_設定1"() -> (w2669:T2)
                                n771 = Unbundle By Name(w2676) -> ("No."=w2675:dbl)
                                n772 = call-poly <vilib>:"Write Key.vi"("section"=w2673, "error in (no error)"=w2666, "value"=w2675, "key"=w2674, "refnum"=w2672) -> ("error out"=w2665:errorcluster, "refnum out"=w2671:T9)  [unwired: 3 in, 2 out]
                                n773 = for {
                                tunnel: w2669 -> [w2720]
                                shift-right: [w2717] -> w2667
                                shift-left: w2671 -> [w2721]
                                tunnel: string[] ["規格", "規格上限", "規格下限", "ポートNo.", "測定モード", "規格単位", "品質チェック項目", "測定周期", "実測MAX", "実測MIN", "実測(MAX)", "実測(MIN)", "測定画面表示ボタン", "ゲージポートNo."] -> [w2719] mode=indexing
                                tunnel: w2662 -> [w2718]
                                shift-right: [w2714] -> w2664
                                shift-left: w2665 -> [w2715]
                                i -> [w2716]
                                n774 = case shown="10" w2716 {
                                tunnel: w2720 -> [w2729 w2737 w2744 w2752 w2760 w2768 w2776 w2784 w2792 w2800 w2809 w2817 w2824 w2832]
                                tunnel: w2719 -> [w2727 w2734 w2743 w2751 w2759 w2767 w2775 w2783 w2791 w2799 w2808 w2816 w2823 w2831]
                                tunnel: w2721 -> [w2726 w2736 w2742 w2750 w2758 w2766 w2774 w2782 w2790 w2798 w2807 w2815 w2822 w2830]
                                tunnel: [w2725 w2732 w2741 w2749 w2757 w2765 w2773 w2781 w2789 w2797 w2806 w2814 w2821 w2829] -> w2717
                                tunnel: w2718 -> [w2724 w2733 w2740 w2748 w2756 w2764 w2772 w2780 w2788 w2796 w2805 w2813 w2820 w2828]
                                tunnel: w2715 -> [w2723 w2731 w2739 w2747 w2755 w2763 w2771 w2779 w2787 w2795 w2804 w2812 w2819 w2827]
                                tunnel: [w2722 w2730 w2738 w2746 w2754 w2762 w2770 w2778 w2786 w2794 w2803 w2811 w2818 w2826] -> w2714
                                frame 0, Default {
                                n775 = Unbundle By Name(w2729) -> ("規格"=w2728:string)
                                n776 = call-poly <vilib>:"Write Key.vi"("section"=w2724, "error in (no error)"=w2723, "value"=w2728, "key"=w2727, "refnum"=w2726) -> ("error out"=w2722:errorcluster, "refnum out"=w2725:T9)  [unwired: 1 in, 4 out]
                                }
                                frame 1 {
                                n777 = Unbundle By Name(w2737) -> ("規格上限"=w2735:string)
                                n778 = call-poly <vilib>:"Write Key.vi"("section"=w2733, "error in (no error)"=w2731, "value"=w2735, "key"=w2734, "refnum"=w2736) -> ("error out"=w2730:errorcluster, "refnum out"=w2732:T9)  [unwired: 1 in, 4 out]
                                }
                                frame 2 {
                                n779 = Unbundle By Name(w2744) -> ("規格下限"=w2745:string)
                                n780 = call-poly <vilib>:"Write Key.vi"("section"=w2740, "error in (no error)"=w2739, "value"=w2745, "key"=w2743, "refnum"=w2742) -> ("error out"=w2738:errorcluster, "refnum out"=w2741:T9)  [unwired: 1 in, 4 out]
                                }
                                frame 3 {
                                n781 = Unbundle By Name(w2752) -> ("ポートNo."=w2753:dbl)
                                n782 = call-poly <vilib>:"Write Key.vi"("section"=w2748, "error in (no error)"=w2747, "value"=w2753, "key"=w2751, "refnum"=w2750) -> ("error out"=w2746:errorcluster, "refnum out"=w2749:T9)  [unwired: 3 in, 2 out]
                                }
                                frame 4 {
                                n783 = Unbundle By Name(w2760) -> ("測定モード"=w2761:u16)
                                n784 = call-poly <vilib>:"Write Key.vi"("section"=w2756, "error in (no error)"=w2755, "value"=w2761, "key"=w2759, "refnum"=w2758) -> ("error out"=w2754:errorcluster, "refnum out"=w2757:T9)  [unwired: 1 in, 4 out]
                                }
                                frame 5 {
                                n785 = Unbundle By Name(w2768) -> ("規格単位"=w2769:string)
                                n786 = call-poly <vilib>:"Write Key.vi"("section"=w2764, "error in (no error)"=w2763, "value"=w2769, "key"=w2767, "refnum"=w2766) -> ("error out"=w2762:errorcluster, "refnum out"=w2765:T9)  [unwired: 1 in, 4 out]
                                }
                                frame 6 {
                                n787 = Unbundle By Name(w2776) -> ("品質チェック項目"=w2777:string)
                                n788 = call-poly <vilib>:"Write Key.vi"("section"=w2772, "error in (no error)"=w2771, "value"=w2777, "key"=w2775, "refnum"=w2774) -> ("error out"=w2770:errorcluster, "refnum out"=w2773:T9)  [unwired: 1 in, 4 out]
                                }
                                frame 7 {
                                n789 = Unbundle By Name(w2784) -> ("測定周期"=w2785:dbl)
                                n790 = call-poly <vilib>:"Write Key.vi"("section"=w2780, "error in (no error)"=w2779, "value"=w2785, "key"=w2783, "refnum"=w2782) -> ("error out"=w2778:errorcluster, "refnum out"=w2781:T9)  [unwired: 3 in, 2 out]
                                }
                                frame 8 {
                                n791 = Unbundle By Name(w2792) -> ("実測値MAX"=w2793:string)
                                n792 = call-poly <vilib>:"Write Key.vi"("section"=w2788, "error in (no error)"=w2787, "value"=w2793, "key"=w2791, "refnum"=w2790) -> ("error out"=w2786:errorcluster, "refnum out"=w2789:T9)  [unwired: 1 in, 4 out]
                                }
                                frame 9 {
                                n793 = Unbundle By Name(w2800) -> ("実測値MIN"=w2801:string)
                                n794 = call-poly <vilib>:"Write Key.vi"("section"=w2796, "error in (no error)"=w2795, "value"=w2801, "key"=w2799, "refnum"=w2798) -> ("error out"=w2794:errorcluster, "refnum out"=w2797:T9)  [unwired: 1 in, 4 out]
                                }
                                frame 10 {
                                n795 = Unbundle By Name(w2809) -> ()  [unwired: 1 out]
                                n796 = call-poly <vilib>:"Write Key.vi"("section"=w2805, "error in (no error)"=w2804, "value"="", "key"=w2808, "refnum"=w2807) -> ("error out"=w2803:errorcluster, "refnum out"=w2806:T9)  [unwired: 1 in, 4 out]
                                }
                                frame 11 {
                                n797 = Unbundle By Name(w2817) -> ()  [unwired: 1 out]
                                n798 = call-poly <vilib>:"Write Key.vi"("section"=w2813, "error in (no error)"=w2812, "value"="", "key"=w2816, "refnum"=w2815) -> ("error out"=w2811:errorcluster, "refnum out"=w2814:T9)  [unwired: 1 in, 4 out]
                                }
                                frame 12 {
                                n799 = Unbundle By Name(w2824) -> ("測定画面表示ボタン"=w2825:bool)
                                n800 = call-poly <vilib>:"Write Key.vi"("section"=w2820, "error in (no error)"=w2819, "value"=w2825, "key"=w2823, "refnum"=w2822) -> ("error out"=w2818:errorcluster, "refnum out"=w2821:T9)  [unwired: 1 in, 4 out]
                                }
                                frame 13 {
                                n801 = Unbundle By Name(w2832) -> ("ゲージポートNo"=w2833:refnum<visa-resource-name>)
                                n802 = call-poly <vilib>:"Write Key.vi"("section"=w2828, "error in (no error)"=w2827, "value"=w2833, "key"=w2831, "refnum"=w2830) -> ("error out"=w2826:errorcluster, "refnum out"=w2829:T9)  [unwired: 1 in, 4 out]
                                }
                                }
                                }
                                n803 = for {
                                shift-right: [w2697] -> w2661
                                shift-left: w2667 -> [w2694]
                                tunnel: string[] ["使用ON/OFF", "CSVヘッダー名"] -> [w2695] mode=indexing
                                tunnel: w2662 -> [w2693]
                                shift-right: [w2691] -> w2658
                                shift-left: w2664 -> [w2692]
                                i -> [w2696]
                                n804 = case shown="1" w2696 {
                                tunnel: [w2705 w2713] -> w2697
                                tunnel: w2695 -> [w2703 w2712]
                                tunnel: w2694 -> [w2702 w2711]
                                tunnel: w2693 -> [w2701 w2710]
                                tunnel: w2692 -> [w2700 w2709]
                                tunnel: [w2699 w2708] -> w2691
                                frame 0, Default {
                                n805 = local read "使用ON/OFFボタン_設定1"() -> (w2698:T5)
                                n806 = Unbundle By Name(w2698) -> ("使用ON/OFF"=w2704:bool)
                                n807 = call-poly <vilib>:"Write Key.vi"("section"=w2701, "error in (no error)"=w2700, "value"=w2704, "key"=w2703, "refnum"=w2702) -> ("error out"=w2699:errorcluster, "refnum out"=w2705:T9)  [unwired: 1 in, 4 out]
                                }
                                frame 1 {
                                n808 = local read "CSV項目名 1"() -> (w2707:T1)
                                n809 = Unbundle By Name(w2707) -> ("CSV項目名"=w2706:string)
                                n810 = call-poly <vilib>:"Write Key.vi"("section"=w2710, "error in (no error)"=w2709, "value"=w2706, "key"=w2712, "refnum"=w2711) -> ("error out"=w2708:errorcluster, "refnum out"=w2713:T9)  [unwired: 1 in, 4 out]
                                }
                                }
                                }
                                n811 = for {
                                tunnel: string[] ["CSV保存先フォルダ"] -> [w2682] mode=indexing
                                shift-right: [w2679] -> w2660
                                shift-left: w2661 -> [w2680]
                                tunnel: w2662 -> [w2681]
                                shift-right: [w2678] -> w2659
                                shift-left: w2658 -> [w2677]
                                i -> [w2683]
                                n812 = case shown="0, デフォルト" w2683 {
                                tunnel: w2682 -> [w2690]
                                tunnel: w2681 -> [w2688]
                                tunnel: w2680 -> [w2687]
                                tunnel: [w2686] -> w2679
                                tunnel: [w2685] -> w2678
                                tunnel: w2677 -> [w2684]
                                frame 0, Default {
                                n813 = local read "CSV保存先フォルダ"() -> (w2689:path)
                                n814 = call-poly <vilib>:"Write Key.vi"("section"=w2688, "error in (no error)"=w2684, "value"=w2689, "key"=w2690, "refnum"=w2687) -> ("error out"=w2685:errorcluster, "refnum out"=w2686:T9)  [unwired: 1 in, 4 out]
                                }
                                }
                                }
                              }
                            }
                          }
                          n815 = call <vilib>:"Close Config Data.vi"("error in (no error)"=w2642, "refnum"=w2643) -> ("error out"=→"iniエラーout":errorcluster)  [unwired: 1 in, 8 out]
                        }
                      }
                    }
                  }
                }
              }
            }
            frame 1 {
              n816 = while {
                tunnel: w2837 -> [w2850]
                tunnel: w2836 -> [w2849]
                tunnel: w2835 -> [w2848]
                tunnel: [w2848] -> w2834
                stop <- TRUE stop-if-true
                w2845 = string[] ["No."]  # キー(配列No)
                w2847 = "設定2"  # セレクション(設定)
                w2846 = "No2."  # セレクション(No)
                # "⑥"
                # "⑤"
                # "⑦"
                # "複製コピー時\nこのまま複製し、\nforループ外の\n①②\nセレクションを変更する\n③④⑤⑥\nローカル変数を設定する項目に合わせる\n⑦複製したケースのTrue定数を消す"
                # "④"
                # "③"
                # "②"
                # "①"
                # "登録ボタンが押された時に動作"
                n817 = local read "No設定クラスタ_設定 2"() -> (w2840:T7)
                n818 = local read "使用ON/OFFボタン_設定 2"() -> (w2841:T5)
                n819 = local read "設定クラスタ_設定 2"() -> (w2839:T2)
                n820 = local read "CSV項目名 2"() -> (w2838:T1)
                n821 = call "設定項目_登録_INI書込サブ.vi"("CSV項目名"=w2838, "設定クラスタ_設定入力"=w2839, "セレクション(設定)"=w2847, "エラー入力"=w2849, "セレクション(No)"=w2846, "使用ON/OFFボタン_設定入力"=w2841, "キー(配列No)"=w2845, "No設定クラスタ_設定入力"=w2840, "Refnum入力"=w2850) -> ("エラー出力"=w2842:errorcluster, "Refnum出力"=w2843:T9)  [unwired: 1 in]
                n822 = call <vilib>:"Close Config Data.vi"("error in (no error)"=w2842, "refnum"=w2843) -> ("error out"=w2844:errorcluster)  [unwired: 1 in, 8 out]
                n823 = local write "iniエラーout"(w2844) -> ()
              }
            }
            frame 2 {
              n824 = while {
                tunnel: w2855 -> [w2868]
                tunnel: w2854 -> [w2867]
                tunnel: w2853 -> [w2866]
                tunnel: [w2866] -> w2852
                stop <- TRUE stop-if-true
                w2863 = string[] ["No."]  # キー(配列No)
                w2865 = "設定3"  # セレクション(設定)
                w2864 = "No3."  # セレクション(No)
                # "⑥"
                # "⑤"
                # "⑦"
                # "複製コピー時\nこのまま複製し、\nforループ外の\n①②\nセレクションを変更する\n③④⑤⑥\nローカル変数を設定する項目に合わせる\n⑦複製したケースのTrue定数を消す"
                # "④"
                # "③"
                # "②"
                # "①"
                # "登録ボタンが押された時に動作"
                n825 = local read "No設定クラスタ_設定 3"() -> (w2858:T7)
                n826 = local read "使用ON/OFFボタン_設定 3"() -> (w2859:T5)
                n827 = local read "設定クラスタ_設定 3"() -> (w2857:T2)
                n828 = local read "CSV項目名 3"() -> (w2856:T1)
                n829 = call "設定項目_登録_INI書込サブ.vi"("CSV項目名"=w2856, "設定クラスタ_設定入力"=w2857, "セレクション(設定)"=w2865, "エラー入力"=w2867, "セレクション(No)"=w2864, "使用ON/OFFボタン_設定入力"=w2859, "キー(配列No)"=w2863, "No設定クラスタ_設定入力"=w2858, "Refnum入力"=w2868) -> ("エラー出力"=w2860:errorcluster, "Refnum出力"=w2861:T9)  [unwired: 1 in]
                n830 = call <vilib>:"Close Config Data.vi"("error in (no error)"=w2860, "refnum"=w2861) -> ("error out"=w2862:errorcluster)  [unwired: 1 in, 8 out]
                n831 = local write "iniエラーout"(w2862) -> ()
              }
            }
            frame 3 {
              n832 = while {
                tunnel: w2873 -> [w2886]
                tunnel: w2872 -> [w2885]
                tunnel: w2871 -> [w2884]
                tunnel: [w2884] -> w2870
                stop <- TRUE stop-if-true
                w2881 = string[] ["No."]  # キー(配列No)
                w2883 = "設定4"  # セレクション(設定)
                w2882 = "No4."  # セレクション(No)
                # "⑥"
                # "⑤"
                # "⑦"
                # "複製コピー時\nこのまま複製し、\nforループ外の\n①②\nセレクションを変更する\n③④⑤⑥\nローカル変数を設定する項目に合わせる\n⑦複製したケースのTrue定数を消す"
                # "④"
                # "③"
                # "②"
                # "①"
                # "登録ボタンが押された時に動作"
                n833 = local read "No設定クラスタ_設定 4"() -> (w2876:T7)
                n834 = local read "使用ON/OFFボタン_設定 4"() -> (w2877:T5)
                n835 = local read "設定クラスタ_設定 4"() -> (w2875:T2)
                n836 = local read "CSV項目名 4"() -> (w2874:T1)
                n837 = call "設定項目_登録_INI書込サブ.vi"("CSV項目名"=w2874, "設定クラスタ_設定入力"=w2875, "セレクション(設定)"=w2883, "エラー入力"=w2885, "セレクション(No)"=w2882, "使用ON/OFFボタン_設定入力"=w2877, "キー(配列No)"=w2881, "No設定クラスタ_設定入力"=w2876, "Refnum入力"=w2886) -> ("エラー出力"=w2878:errorcluster, "Refnum出力"=w2879:T9)  [unwired: 1 in]
                n838 = call <vilib>:"Close Config Data.vi"("error in (no error)"=w2878, "refnum"=w2879) -> ("error out"=w2880:errorcluster)  [unwired: 1 in, 8 out]
                n839 = local write "iniエラーout"(w2880) -> ()
              }
            }
            frame 4 {
              n840 = while {
                tunnel: w2891 -> [w2904]
                tunnel: w2890 -> [w2903]
                tunnel: w2889 -> [w2902]
                tunnel: [w2902] -> w2888
                stop <- TRUE stop-if-true
                w2899 = string[] ["No."]  # キー(配列No)
                w2901 = "設定5"  # セレクション(設定)
                w2900 = "No5."  # セレクション(No)
                # "⑥"
                # "⑤"
                # "⑦"
                # "複製コピー時\nこのまま複製し、\nforループ外の\n①②\nセレクションを変更する\n③④⑤⑥\nローカル変数を設定する項目に合わせる\n⑦複製したケースのTrue定数を消す"
                # "④"
                # "③"
                # "②"
                # "①"
                # "登録ボタンが押された時に動作"
                n841 = local read "No設定クラスタ_設定 5"() -> (w2894:T7)
                n842 = local read "使用ON/OFFボタン_設定 5"() -> (w2895:T5)
                n843 = local read "設定クラスタ_設定 5"() -> (w2893:T2)
                n844 = local read "CSV項目名 5"() -> (w2892:T1)
                n845 = call "設定項目_登録_INI書込サブ.vi"("CSV項目名"=w2892, "設定クラスタ_設定入力"=w2893, "セレクション(設定)"=w2901, "エラー入力"=w2903, "セレクション(No)"=w2900, "使用ON/OFFボタン_設定入力"=w2895, "キー(配列No)"=w2899, "No設定クラスタ_設定入力"=w2894, "Refnum入力"=w2904) -> ("エラー出力"=w2896:errorcluster, "Refnum出力"=w2897:T9)  [unwired: 1 in]
                n846 = call <vilib>:"Close Config Data.vi"("error in (no error)"=w2896, "refnum"=w2897) -> ("error out"=w2898:errorcluster)  [unwired: 1 in, 8 out]
                n847 = local write "iniエラーout"(w2898) -> ()
              }
            }
            frame 5 {
              n848 = while {
                tunnel: w2909 -> [w2922]
                tunnel: w2908 -> [w2921]
                tunnel: w2907 -> [w2920]
                tunnel: [w2920] -> w2906
                stop <- TRUE stop-if-true
                w2917 = string[] ["No."]  # キー(配列No)
                w2919 = "設定6"  # セレクション(設定)
                w2918 = "No6."  # セレクション(No)
                # "⑥"
                # "⑤"
                # "⑦"
                # "複製コピー時\nこのまま複製し、\nforループ外の\n①②\nセレクションを変更する\n③④⑤⑥\nローカル変数を設定する項目に合わせる\n⑦複製したケースのTrue定数を消す"
                # "④"
                # "③"
                # "②"
                # "①"
                # "登録ボタンが押された時に動作"
                n849 = local read "No設定クラスタ_設定 6"() -> (w2912:T7)
                n850 = local read "使用ON/OFFボタン_設定 6"() -> (w2913:T5)
                n851 = local read "設定クラスタ_設定 6"() -> (w2911:T2)
                n852 = local read "CSV項目名 6"() -> (w2910:T1)
                n853 = call "設定項目_登録_INI書込サブ.vi"("CSV項目名"=w2910, "設定クラスタ_設定入力"=w2911, "セレクション(設定)"=w2919, "エラー入力"=w2921, "セレクション(No)"=w2918, "使用ON/OFFボタン_設定入力"=w2913, "キー(配列No)"=w2917, "No設定クラスタ_設定入力"=w2912, "Refnum入力"=w2922) -> ("エラー出力"=w2914:errorcluster, "Refnum出力"=w2915:T9)  [unwired: 1 in]
                n854 = call <vilib>:"Close Config Data.vi"("error in (no error)"=w2914, "refnum"=w2915) -> ("error out"=w2916:errorcluster)  [unwired: 1 in, 8 out]
                n855 = local write "iniエラーout"(w2916) -> ()
              }
            }
            frame 6 {
              n856 = while {
                tunnel: w2927 -> [w2940]
                tunnel: w2926 -> [w2939]
                tunnel: w2925 -> [w2938]
                tunnel: [w2938] -> w2924
                stop <- TRUE stop-if-true
                w2935 = string[] ["No."]  # キー(配列No)
                w2937 = "設定7"  # セレクション(設定)
                w2936 = "No7."  # セレクション(No)
                # "⑥"
                # "⑤"
                # "⑦"
                # "複製コピー時\nこのまま複製し、\nforループ外の\n①②\nセレクションを変更する\n③④⑤⑥\nローカル変数を設定する項目に合わせる\n⑦複製したケースのTrue定数を消す"
                # "④"
                # "③"
                # "②"
                # "①"
                # "登録ボタンが押された時に動作"
                n857 = local read "No設定クラスタ_設定 7"() -> (w2930:T7)
                n858 = local read "使用ON/OFFボタン_設定 7"() -> (w2931:T5)
                n859 = local read "設定クラスタ_設定 7"() -> (w2929:T2)
                n860 = local read "CSV項目名 7"() -> (w2928:T1)
                n861 = call "設定項目_登録_INI書込サブ.vi"("CSV項目名"=w2928, "設定クラスタ_設定入力"=w2929, "セレクション(設定)"=w2937, "エラー入力"=w2939, "セレクション(No)"=w2936, "使用ON/OFFボタン_設定入力"=w2931, "キー(配列No)"=w2935, "No設定クラスタ_設定入力"=w2930, "Refnum入力"=w2940) -> ("エラー出力"=w2932:errorcluster, "Refnum出力"=w2933:T9)  [unwired: 1 in]
                n862 = call <vilib>:"Close Config Data.vi"("error in (no error)"=w2932, "refnum"=w2933) -> ("error out"=w2934:errorcluster)  [unwired: 1 in, 8 out]
                n863 = local write "iniエラーout"(w2934) -> ()
              }
            }
            frame 7 {
              n864 = while {
                tunnel: w2945 -> [w2958]
                tunnel: w2944 -> [w2957]
                tunnel: w2943 -> [w2956]
                tunnel: [w2956] -> w2942
                stop <- TRUE stop-if-true
                w2953 = string[] ["No."]  # キー(配列No)
                w2955 = "設定8"  # セレクション(設定)
                w2954 = "No8."  # セレクション(No)
                # "⑥"
                # "⑤"
                # "⑦"
                # "複製コピー時\nこのまま複製し、\nforループ外の\n①②\nセレクションを変更する\n③④⑤⑥\nローカル変数を設定する項目に合わせる\n⑦複製したケースのTrue定数を消す"
                # "④"
                # "③"
                # "②"
                # "①"
                # "登録ボタンが押された時に動作"
                n865 = local read "No設定クラスタ_設定 8"() -> (w2948:T7)
                n866 = local read "使用ON/OFFボタン_設定 8"() -> (w2949:T5)
                n867 = local read "設定クラスタ_設定 8"() -> (w2947:T2)
                n868 = local read "CSV項目名 8"() -> (w2946:T1)
                n869 = call "設定項目_登録_INI書込サブ.vi"("CSV項目名"=w2946, "設定クラスタ_設定入力"=w2947, "セレクション(設定)"=w2955, "エラー入力"=w2957, "セレクション(No)"=w2954, "使用ON/OFFボタン_設定入力"=w2949, "キー(配列No)"=w2953, "No設定クラスタ_設定入力"=w2948, "Refnum入力"=w2958) -> ("エラー出力"=w2950:errorcluster, "Refnum出力"=w2951:T9)  [unwired: 1 in]
                n870 = call <vilib>:"Close Config Data.vi"("error in (no error)"=w2950, "refnum"=w2951) -> ("error out"=w2952:errorcluster)  [unwired: 1 in, 8 out]
                n871 = local write "iniエラーout"(w2952) -> ()
              }
            }
            frame 8 {
              n872 = while {
                tunnel: w2963 -> [w2976]
                tunnel: w2962 -> [w2975]
                tunnel: w2961 -> [w2974]
                tunnel: [w2974] -> w2960
                stop <- TRUE stop-if-true
                w2971 = string[] ["No."]  # キー(配列No)
                w2973 = "設定9"  # セレクション(設定)
                w2972 = "No9."  # セレクション(No)
                # "⑥"
                # "⑤"
                # "⑦"
                # "複製コピー時\nこのまま複製し、\nforループ外の\n①②\nセレクションを変更する\n③④⑤⑥\nローカル変数を設定する項目に合わせる\n⑦複製したケースのTrue定数を消す"
                # "④"
                # "③"
                # "②"
                # "①"
                # "登録ボタンが押された時に動作"
                n873 = local read "No設定クラスタ_設定 9"() -> (w2966:T7)
                n874 = local read "使用ON/OFFボタン_設定 9"() -> (w2967:T5)
                n875 = local read "設定クラスタ_設定 9"() -> (w2965:T2)
                n876 = local read "CSV項目名 9"() -> (w2964:T1)
                n877 = call "設定項目_登録_INI書込サブ.vi"("CSV項目名"=w2964, "設定クラスタ_設定入力"=w2965, "セレクション(設定)"=w2973, "エラー入力"=w2975, "セレクション(No)"=w2972, "使用ON/OFFボタン_設定入力"=w2967, "キー(配列No)"=w2971, "No設定クラスタ_設定入力"=w2966, "Refnum入力"=w2976) -> ("エラー出力"=w2968:errorcluster, "Refnum出力"=w2969:T9)  [unwired: 1 in]
                n878 = call <vilib>:"Close Config Data.vi"("error in (no error)"=w2968, "refnum"=w2969) -> ("error out"=w2970:errorcluster)  [unwired: 1 in, 8 out]
                n879 = local write "iniエラーout"(w2970) -> ()
              }
            }
            frame 9 {
              n880 = while {
                tunnel: w2981 -> [w2994]
                tunnel: w2980 -> [w2993]
                tunnel: w2979 -> [w2992]
                tunnel: [w2992] -> w2978
                stop <- TRUE stop-if-true
                w2989 = string[] ["No."]  # キー(配列No)
                w2991 = "設定10"  # セレクション(設定)
                w2990 = "No10."  # セレクション(No)
                # "⑥"
                # "⑤"
                # "⑦"
                # "複製コピー時\nこのまま複製し、\nforループ外の\n①②\nセレクションを変更する\n③④⑤⑥\nローカル変数を設定する項目に合わせる\n⑦複製したケースのTrue定数を消す"
                # "④"
                # "③"
                # "②"
                # "①"
                # "登録ボタンが押された時に動作"
                n881 = local read "No設定クラスタ_設定 10"() -> (w2984:T7)
                n882 = local read "使用ON/OFFボタン_設定 10"() -> (w2985:T5)
                n883 = local read "設定クラスタ_設定 10"() -> (w2983:T2)
                n884 = local read "CSV項目名 10"() -> (w2982:T1)
                n885 = call "設定項目_登録_INI書込サブ.vi"("CSV項目名"=w2982, "設定クラスタ_設定入力"=w2983, "セレクション(設定)"=w2991, "エラー入力"=w2993, "セレクション(No)"=w2990, "使用ON/OFFボタン_設定入力"=w2985, "キー(配列No)"=w2989, "No設定クラスタ_設定入力"=w2984, "Refnum入力"=w2994) -> ("エラー出力"=w2986:errorcluster, "Refnum出力"=w2987:T9)  [unwired: 1 in]
                n886 = call <vilib>:"Close Config Data.vi"("error in (no error)"=w2986, "refnum"=w2987) -> ("error out"=w2988:errorcluster)  [unwired: 1 in, 8 out]
                n887 = local write "iniエラーout"(w2988) -> ()
              }
            }
            frame 10 {
              n888 = while {
                tunnel: w2999 -> [w3012]
                tunnel: w2998 -> [w3011]
                tunnel: w2997 -> [w3010]
                tunnel: [w3010] -> w2996
                stop <- TRUE stop-if-true
                w3007 = string[] ["No."]  # キー(配列No)
                w3009 = "設定11"  # セレクション(設定)
                w3008 = "No11."  # セレクション(No)
                # "⑥"
                # "⑤"
                # "⑦"
                # "複製コピー時\nこのまま複製し、\nforループ外の\n①②\nセレクションを変更する\n③④⑤⑥\nローカル変数を設定する項目に合わせる\n⑦複製したケースのTrue定数を消す"
                # "④"
                # "③"
                # "②"
                # "①"
                # "登録ボタンが押された時に動作"
                n889 = local read "No設定クラスタ_設定 11"() -> (w3002:T7)
                n890 = local read "使用ON/OFFボタン_設定 11"() -> (w3003:T5)
                n891 = local read "設定クラスタ_設定 11"() -> (w3001:T2)
                n892 = local read "CSV項目名 11"() -> (w3000:T1)
                n893 = call "設定項目_登録_INI書込サブ.vi"("CSV項目名"=w3000, "設定クラスタ_設定入力"=w3001, "セレクション(設定)"=w3009, "エラー入力"=w3011, "セレクション(No)"=w3008, "使用ON/OFFボタン_設定入力"=w3003, "キー(配列No)"=w3007, "No設定クラスタ_設定入力"=w3002, "Refnum入力"=w3012) -> ("エラー出力"=w3004:errorcluster, "Refnum出力"=w3005:T9)  [unwired: 1 in]
                n894 = call <vilib>:"Close Config Data.vi"("error in (no error)"=w3004, "refnum"=w3005) -> ("error out"=w3006:errorcluster)  [unwired: 1 in, 8 out]
                n895 = local write "iniエラーout"(w3006) -> ()
              }
            }
            frame 11 {
              n896 = while {
                tunnel: w3017 -> [w3030]
                tunnel: w3016 -> [w3029]
                tunnel: w3015 -> [w3028]
                tunnel: [w3028] -> w3014
                stop <- TRUE stop-if-true
                w3025 = string[] ["No."]  # キー(配列No)
                w3027 = "設定12"  # セレクション(設定)
                w3026 = "No12."  # セレクション(No)
                # "⑥"
                # "⑤"
                # "⑦"
                # "複製コピー時\nこのまま複製し、\nforループ外の\n①②\nセレクションを変更する\n③④⑤⑥\nローカル変数を設定する項目に合わせる\n⑦複製したケースのTrue定数を消す"
                # "④"
                # "③"
                # "②"
                # "①"
                # "登録ボタンが押された時に動作"
                n897 = local read "No設定クラスタ_設定 12"() -> (w3020:T7)
                n898 = local read "使用ON/OFFボタン_設定 12"() -> (w3021:T5)
                n899 = local read "設定クラスタ_設定 12"() -> (w3019:T2)
                n900 = local read "CSV項目名 12"() -> (w3018:T1)
                n901 = call "設定項目_登録_INI書込サブ.vi"("CSV項目名"=w3018, "設定クラスタ_設定入力"=w3019, "セレクション(設定)"=w3027, "エラー入力"=w3029, "セレクション(No)"=w3026, "使用ON/OFFボタン_設定入力"=w3021, "キー(配列No)"=w3025, "No設定クラスタ_設定入力"=w3020, "Refnum入力"=w3030) -> ("エラー出力"=w3022:errorcluster, "Refnum出力"=w3023:T9)  [unwired: 1 in]
                n902 = call <vilib>:"Close Config Data.vi"("error in (no error)"=w3022, "refnum"=w3023) -> ("error out"=w3024:errorcluster)  [unwired: 1 in, 8 out]
                n903 = local write "iniエラーout"(w3024) -> ()
              }
            }
            frame 12 {
            }
          }
        }
      }
      frame "キャンセルして戻る" {
        # "ループ停止True処理のみ\n他項目複製時も変更無"
        # "キャンセルボタンが押されたら何もせずに画面を閉じる"
      }
      frame "初期化" {
        # "②"
        # "①"
        # "他の項目を複製した時に変更する項目\n①複製したボタン\n②複製した配列\nを追加"
        # "初期化ボタンを押した時、全ての項目がキャンセルされる"
        n904 = local read "使用ON/OFFボタン_リセット用"() -> (w3036:T5)
        n905 = local write "使用ON/OFFボタン_設定 11"(w3036) -> ()
        n906 = local write "使用ON/OFFボタン_設定 10"(w3036) -> ()
        n907 = local write "使用ON/OFFボタン_設定 12"(w3036) -> ()
        n908 = local write "使用ON/OFFボタン_設定1"(w3036) -> ()
        n909 = local write "使用ON/OFFボタン_設定 2"(w3036) -> ()
        n910 = local write "使用ON/OFFボタン_設定 3"(w3036) -> ()
        n911 = local write "使用ON/OFFボタン_設定 4"(w3036) -> ()
        n912 = local write "使用ON/OFFボタン_設定 5"(w3036) -> ()
        n913 = local write "使用ON/OFFボタン_設定 6"(w3036) -> ()
        n914 = local write "使用ON/OFFボタン_設定 7"(w3036) -> ()
        n915 = local write "使用ON/OFFボタン_設定 8"(w3036) -> ()
        n916 = local write "使用ON/OFFボタン_設定 9"(w3036) -> ()
        n917 = local read "CSV保存名_リセット用"() -> (w3035:string)
        n918 = local read "品番・品名_リセット用"() -> (w3039:T3)
        n919 = local read "設定クラスタ_リセット"() -> (w3037:T4)
        n920 = local write "品番・品名クラスタ_設定"(w3039) -> ()
        n921 = local write "② CSV保存名"(w3035) -> ()
        n922 = local write "設定クラスタ_設定1"(w3037) -> ()
        n923 = local write "設定クラスタ_設定 2"(w3037) -> ()
        n924 = local write "設定クラスタ_設定 3"(w3037) -> ()
        n925 = local write "設定クラスタ_設定 4"(w3037) -> ()
        n926 = local write "設定クラスタ_設定 5"(w3037) -> ()
        n927 = local write "設定クラスタ_設定 6"(w3037) -> ()
        n928 = local write "設定クラスタ_設定 7"(w3037) -> ()
        n929 = local write "設定クラスタ_設定 8"(w3037) -> ()
        n930 = local write "設定クラスタ_設定 9"(w3037) -> ()
        n931 = local write "設定クラスタ_設定 10"(w3037) -> ()
        n932 = local write "設定クラスタ_設定 11"(w3037) -> ()
        n933 = local write "設定クラスタ_設定 12"(w3037) -> ()
        n934 = local write "CSV保存先フォルダ"("CSV保存先フォルダ_リセット用") -> ()
        n935 = local read "CSV項目名_リセット用"() -> (w3034:T1)
        n936 = local write "CSV項目名 1"(w3034) -> ()
        n937 = local write "CSV項目名 2"(w3034) -> ()
        n938 = local write "CSV項目名 3"(w3034) -> ()
        n939 = local write "CSV項目名 4"(w3034) -> ()
        n940 = local write "CSV項目名 5"(w3034) -> ()
        n941 = local write "CSV項目名 6"(w3034) -> ()
        n942 = local write "CSV項目名 7"(w3034) -> ()
        n943 = local write "CSV項目名 8"(w3034) -> ()
        n944 = local write "CSV項目名 9"(w3034) -> ()
        n945 = local write "CSV項目名 10"(w3034) -> ()
        n946 = local write "CSV項目名 11"(w3034) -> ()
        n947 = local write "CSV項目名 12"(w3034) -> ()
      }
      frame "ゲージ確認" {
        # "他複製時に変更する項目\n①\nケースストラクチャ\"2\"複製\n②③\nローカル変数\n④\nケースストラクチャ\"2\"複製\nケース内の②③の\nローカル変数\n\n⑤\nループカウント修正"
        n948 = flat-sequence {
          tunnel: w3041 -> [w3043]
          frame #0 {
            w3045 = T8."Disabled and Grayed Out" ("無効")
            n949 = local read "ゲージ確認ボタンBOOL"() -> (w3042:bool)
            n950 = local read "測定周期/ms"() -> (w3044:dbl)
            n951 = call "ゲージデータ取り込み.vi"("測定周期/ms"=w3044, "値転記用配列_\n設定項目画面からの転記"=w3043, "ゲージ確認ボタンBOOL"=w3042) -> ()  [unwired: 7 in, 2 out]
            n952 = while {
              tunnel: w3044 -> [w3047]
              stop <- w3048 stop-if-true
              # "⑤"
              n953 = for {
                N: 12 -> [_]
                i -> [w3054]
                # "文字列がERRERだったらERRERを返す\nそれ以外は数値を返す"
                # "文字列からスキャンで文字列抽出"
                # "取り出した文字列データがERRERという文字列か判別、取り出した文字列データが数値か判別し、ERRERだったらERRERを返し、それ以外は数値の文字列を返す"
                # "①"
                n954 = global read "測定データ転記.vi" "測定転記一時データ"() -> (w3055:string[])
                n955 = Index Array(array=w3055, index=w3054) -> (element=w3052:string)
                n956 = for {
                  N: 1 -> [_]
                  tunnel: w3052 -> [w3066]
                  tunnel: [w3061] -> w3051 mode=indexing if=w3062
                  n957 = Scan From String(format string=" %f ", input string=w3066) -> (error out=w3064:errorcluster, output 1=w3061:dbl)  [unwired: 3 in, 2 out]
                  n958 = Unbundle By Name(w3064) -> ("status"=w3063:bool)
                  n959 = Not(x=w3063) -> (.not. x?=w3062:bool)
                }
                n960 = Index Array(array=w3051, index=0) -> (element=w3050:dbl)
                n961 = Number To Fractional String(number=w3050, precision (6)=3) -> (F-format string=w3057:string)  [unwired: 2 in]
                n962 = Equal?(x=w3052, y="ERROR") -> (x = y?=w3059:bool)
                n963 = Select(t=w3052, s=w3059, f=w3057) -> (s? t:f=w3058:string)
                n964 = case shown="2" w3054 {
                  tunnel: w3058 -> [w3067 w3070 w3073 w3076 w3079 w3082 w3085 w3088 w3091 w3094 w3097 w3100]
                  frame 0, Default {
                    # "③"
                    # "②"
                    n965 = local read "設定クラスタ_設定1"() -> (w3069:T2)
                    n966 = Bundle By Name(cluster=w3069, "実測値(MAX)"=w3067) -> (w3068:T2)
                    n967 = local write "設定クラスタ_設定1"(w3068) -> ()
                  }
                  frame 1 {
                    # "③"
                    # "②"
                    n968 = local read "設定クラスタ_設定 2"() -> (w3072:T2)
                    n969 = Bundle By Name(cluster=w3072, "実測値(MAX)"=w3070) -> (w3071:T2)
                    n970 = local write "設定クラスタ_設定 2"(w3071) -> ()
                  }
                  frame 2 {
                    # "③"
                    # "②"
                    n971 = local read "設定クラスタ_設定 3"() -> (w3075:T2)
                    n972 = Bundle By Name(cluster=w3075, "実測値(MAX)"=w3073) -> (w3074:T2)
                    n973 = local write "設定クラスタ_設定 3"(w3074) -> ()
                  }
                  frame 3 {
                    # "③"
                    # "②"
                    n974 = local read "設定クラスタ_設定 4"() -> (w3078:T2)
                    n975 = Bundle By Name(cluster=w3078, "実測値(MAX)"=w3076) -> (w3077:T2)
                    n976 = local write "設定クラスタ_設定 4"(w3077) -> ()
                  }
                  frame 4 {
                    # "③"
                    # "②"
                    n977 = local read "設定クラスタ_設定 5"() -> (w3081:T2)
                    n978 = Bundle By Name(cluster=w3081, "実測値(MAX)"=w3079) -> (w3080:T2)
                    n979 = local write "設定クラスタ_設定 5"(w3080) -> ()
                  }
                  frame 5 {
                    # "③"
                    # "②"
                    n980 = local read "設定クラスタ_設定 6"() -> (w3084:T2)
                    n981 = Bundle By Name(cluster=w3084, "実測値(MAX)"=w3082) -> (w3083:T2)
                    n982 = local write "設定クラスタ_設定 6"(w3083) -> ()
                  }
                  frame 6 {
                    # "③"
                    # "②"
                    n983 = local read "設定クラスタ_設定 7"() -> (w3087:T2)
                    n984 = Bundle By Name(cluster=w3087, "実測値(MAX)"=w3085) -> (w3086:T2)
                    n985 = local write "設定クラスタ_設定 7"(w3086) -> ()
                  }
                  frame 7 {
                    # "③"
                    # "②"
                    n986 = local read "設定クラスタ_設定 8"() -> (w3090:T2)
                    n987 = Bundle By Name(cluster=w3090, "実測値(MAX)"=w3088) -> (w3089:T2)
                    n988 = local write "設定クラスタ_設定 8"(w3089) -> ()
                  }
                  frame 8 {
                    # "③"
                    # "②"
                    n989 = local read "設定クラスタ_設定 9"() -> (w3093:T2)
                    n990 = Bundle By Name(cluster=w3093, "実測値(MAX)"=w3091) -> (w3092:T2)
                    n991 = local write "設定クラスタ_設定 9"(w3092) -> ()
                  }
                  frame 9 {
                    # "③"
                    # "②"
                    n992 = local read "設定クラスタ_設定 10"() -> (w3096:T2)
                    n993 = Bundle By Name(cluster=w3096, "実測値(MAX)"=w3094) -> (w3095:T2)
                    n994 = local write "設定クラスタ_設定 10"(w3095) -> ()
                  }
                  frame 10 {
                    # "③"
                    # "②"
                    n995 = local read "設定クラスタ_設定 11"() -> (w3099:T2)
                    n996 = Bundle By Name(cluster=w3099, "実測値(MAX)"=w3097) -> (w3098:T2)
                    n997 = local write "設定クラスタ_設定 11"(w3098) -> ()
                  }
                  frame 11 {
                    # "③"
                    # "②"
                    n998 = local read "設定クラスタ_設定 12"() -> (w3102:T2)
                    n999 = Bundle By Name(cluster=w3102, "実測値(MAX)"=w3100) -> (w3101:T2)
                    n1000 = local write "設定クラスタ_設定 12"(w3101) -> ()
                  }
                }
              }
              n1001 = Wait Until Next ms Multiple(millisecond multiple=w3047) -> ()  [unwired: 1 out]
              n1002 = global read "VISA停止_G.vi" "VISA停止_\nグローバル"() -> (w3048:bool)
            }
            n1003 = property on="登録ボタン" class="Bool"("DisabledEnum"=w3045) -> ()  [unwired: 2 in, 2 out]
            n1004 = property on="キャンセルして戻るボタン" class="Bool"("DisabledEnum"=w3045) -> ()  [unwired: 2 in, 2 out]
          }
          frame #1 {
            w3103 = T8."Enabled" ("無効")
            w3104 = ""
            # "値の初期化"
            n1005 = local read "設定クラスタ_設定 10"() -> (w3118:T2)
            n1006 = Bundle By Name(cluster=w3118, "実測値(MAX)"=w3104) -> (w3117:T2)
            n1007 = local read "設定クラスタ_設定 11"() -> (w3108:T2)
            n1008 = Bundle By Name(cluster=w3108, "実測値(MAX)"=w3104) -> (w3107:T2)
            n1009 = local read "設定クラスタ_設定 12"() -> (w3105:T2)
            n1010 = Bundle By Name(cluster=w3105, "実測値(MAX)"=w3104) -> (w3106:T2)
            n1011 = local read "設定クラスタ_設定 2"() -> (w3126:T2)
            n1012 = Bundle By Name(cluster=w3126, "実測値(MAX)"=w3104) -> (w3125:T2)
            n1013 = local read "設定クラスタ_設定 3"() -> (w3123:T2)
            n1014 = Bundle By Name(cluster=w3123, "実測値(MAX)"=w3104) -> (w3124:T2)
            n1015 = local read "設定クラスタ_設定 4"() -> (w3122:T2)
            n1016 = Bundle By Name(cluster=w3122, "実測値(MAX)"=w3104) -> (w3121:T2)
            n1017 = local read "設定クラスタ_設定 5"() -> (w3119:T2)
            n1018 = Bundle By Name(cluster=w3119, "実測値(MAX)"=w3104) -> (w3120:T2)
            n1019 = local read "設定クラスタ_設定 6"() -> (w3110:T2)
            n1020 = Bundle By Name(cluster=w3110, "実測値(MAX)"=w3104) -> (w3109:T2)
            n1021 = local read "設定クラスタ_設定 7"() -> (w3111:T2)
            n1022 = Bundle By Name(cluster=w3111, "実測値(MAX)"=w3104) -> (w3112:T2)
            n1023 = local read "設定クラスタ_設定 8"() -> (w3114:T2)
            n1024 = Bundle By Name(cluster=w3114, "実測値(MAX)"=w3104) -> (w3113:T2)
            n1025 = local read "設定クラスタ_設定 9"() -> (w3115:T2)
            n1026 = Bundle By Name(cluster=w3115, "実測値(MAX)"=w3104) -> (w3116:T2)
            n1027 = local read "設定クラスタ_設定1"() -> (w3127:T2)
            n1028 = Bundle By Name(cluster=w3127, "実測値(MAX)"=w3104) -> (w3128:T2)
            n1029 = property on="登録ボタン" class="Bool"("DisabledEnum"=w3103) -> ()  [unwired: 2 in, 2 out]
            n1030 = property on="キャンセルして戻るボタン" class="Bool"("DisabledEnum"=w3103) -> ()  [unwired: 2 in, 2 out]
            n1031 = local write "設定クラスタ_設定 10"(w3117) -> ()
            n1032 = local write "設定クラスタ_設定 11"(w3107) -> ()
            n1033 = local write "設定クラスタ_設定 12"(w3106) -> ()
            n1034 = local write "設定クラスタ_設定 2"(w3125) -> ()
            n1035 = local write "設定クラスタ_設定 3"(w3124) -> ()
            n1036 = local write "設定クラスタ_設定 4"(w3121) -> ()
            n1037 = local write "設定クラスタ_設定 5"(w3120) -> ()
            n1038 = local write "設定クラスタ_設定 6"(w3109) -> ()
            n1039 = local write "設定クラスタ_設定 7"(w3112) -> ()
            n1040 = local write "設定クラスタ_設定 8"(w3113) -> ()
            n1041 = local write "設定クラスタ_設定 9"(w3116) -> ()
            n1042 = local write "設定クラスタ_設定1"(w3128) -> ()
          }
        }
      }
      frame "キャンセル1" {
        n1043 = local read "使用ON/OFFボタン_リセット用"() -> (w3134:T5)
        n1044 = local read "設定クラスタ_リセット"() -> (w3131:T4)
        n1045 = local read "CSV項目名_リセット用"() -> (w3129:T1)
        n1046 = local write "使用ON/OFFボタン_設定1"(w3134) -> ()
        n1047 = local write "CSV項目名 1"(w3129) -> ()
        n1048 = local write "設定クラスタ_設定1"(w3131) -> ()
        n1049 = Replace Array Subset(array=w3133, new element=w3131, index=0) -> (w3132:T2[])
      }
      frame "キャンセル2" {
        # "④"
        # "③"
        # "②"
        # "①"
        # "複製時の変更項目下に有"
        # "複製時の変更項目\n①②　④\nグローバル変数\n③\n指標値"
        n1050 = local read "使用ON/OFFボタン_リセット用"() -> (w3140:T5)
        n1051 = local read "CSV項目名_リセット用"() -> (w3135:T1)
        n1052 = local read "設定クラスタ_リセット"() -> (w3137:T4)
        n1053 = local write "CSV項目名 2"(w3135) -> ()
        n1054 = local write "使用ON/OFFボタン_設定 2"(w3140) -> ()
        n1055 = local write "設定クラスタ_設定 2"(w3137) -> ()
        n1056 = Replace Array Subset(array=w3139, new element=w3137, index=1) -> (w3138:T2[])
      }
      frame "キャンセル3" {
        # "④"
        # "複製時の変更項目\n①②　④\nグローバル変数\n③\n指標値"
        # "③"
        # "②"
        # "①"
        # "複製時の変更項目下に有"
        n1057 = local read "使用ON/OFFボタン_リセット用"() -> (w3146:T5)
        n1058 = local read "設定クラスタ_リセット"() -> (w3143:T4)
        n1059 = local read "CSV項目名_リセット用"() -> (w3141:T1)
        n1060 = local write "使用ON/OFFボタン_設定 3"(w3146) -> ()
        n1061 = local write "CSV項目名 3"(w3141) -> ()
        n1062 = local write "設定クラスタ_設定 3"(w3143) -> ()
        n1063 = Replace Array Subset(array=w3145, new element=w3143, index=2) -> (w3144:T2[])
      }
      frame "キャンセル4" {
        # "④"
        # "複製時の変更項目\n①②　④\nグローバル変数\n③\n指標値"
        # "③"
        # "②"
        # "①"
        # "複製時の変更項目下に有"
        n1064 = local read "使用ON/OFFボタン_リセット用"() -> (w3152:T5)
        n1065 = local read "設定クラスタ_リセット"() -> (w3149:T4)
        n1066 = local read "CSV項目名_リセット用"() -> (w3147:T1)
        n1067 = local write "使用ON/OFFボタン_設定 4"(w3152) -> ()
        n1068 = local write "CSV項目名 4"(w3147) -> ()
        n1069 = local write "設定クラスタ_設定 4"(w3149) -> ()
        n1070 = Replace Array Subset(array=w3151, new element=w3149, index=3) -> (w3150:T2[])
      }
      frame "キャンセル5" {
        # "④"
        # "複製時の変更項目\n①②　④\nグローバル変数\n③\n指標値"
        # "③"
        # "②"
        # "①"
        # "複製時の変更項目下に有"
        n1071 = local read "使用ON/OFFボタン_リセット用"() -> (w3158:T5)
        n1072 = local read "CSV項目名_リセット用"() -> (w3153:T1)
        n1073 = local read "設定クラスタ_リセット"() -> (w3155:T4)
        n1074 = local write "CSV項目名 5"(w3153) -> ()
        n1075 = local write "使用ON/OFFボタン_設定 5"(w3158) -> ()
        n1076 = local write "設定クラスタ_設定 5"(w3155) -> ()
        n1077 = Replace Array Subset(array=w3157, new element=w3155, index=4) -> (w3156:T2[])
      }
      frame "キャンセル6" {
        # "④"
        # "複製時の変更項目\n①②　④\nグローバル変数\n③\n指標値"
        # "③"
        # "②"
        # "①"
        # "複製時の変更項目下に有"
        n1078 = local read "使用ON/OFFボタン_リセット用"() -> (w3164:T5)
        n1079 = local read "設定クラスタ_リセット"() -> (w3161:T4)
        n1080 = local read "CSV項目名_リセット用"() -> (w3159:T1)
        n1081 = local write "使用ON/OFFボタン_設定 6"(w3164) -> ()
        n1082 = local write "CSV項目名 6"(w3159) -> ()
        n1083 = local write "設定クラスタ_設定 6"(w3161) -> ()
        n1084 = Replace Array Subset(array=w3163, new element=w3161, index=5) -> (w3162:T2[])
      }
      frame "キャンセル7" {
        # "④"
        # "複製時の変更項目\n①②　④\nグローバル変数\n③\n指標値"
        # "③"
        # "②"
        # "①"
        # "複製時の変更項目下に有"
        n1085 = local read "使用ON/OFFボタン_リセット用"() -> (w3170:T5)
        n1086 = local read "設定クラスタ_リセット"() -> (w3167:T4)
        n1087 = local read "CSV項目名_リセット用"() -> (w3165:T1)
        n1088 = local write "使用ON/OFFボタン_設定 7"(w3170) -> ()
        n1089 = local write "CSV項目名 7"(w3165) -> ()
        n1090 = local write "設定クラスタ_設定 7"(w3167) -> ()
        n1091 = Replace Array Subset(array=w3169, new element=w3167, index=6) -> (w3168:T2[])
      }
      frame "キャンセル8" {
        # "④"
        # "複製時の変更項目\n①②　④\nグローバル変数\n③\n指標値"
        # "③"
        # "②"
        # "①"
        # "複製時の変更項目下に有"
        n1092 = local read "使用ON/OFFボタン_リセット用"() -> (w3176:T5)
        n1093 = local read "設定クラスタ_リセット"() -> (w3173:T4)
        n1094 = local read "CSV項目名_リセット用"() -> (w3171:T1)
        n1095 = local write "CSV項目名 8"(w3171) -> ()
        n1096 = local write "使用ON/OFFボタン_設定 8"(w3176) -> ()
        n1097 = local write "設定クラスタ_設定 8"(w3173) -> ()
        n1098 = Replace Array Subset(array=w3175, new element=w3173, index=7) -> (w3174:T2[])
      }
      frame "キャンセル9" {
        # "④"
        # "複製時の変更項目\n①②　④\nグローバル変数\n③\n指標値"
        # "③"
        # "②"
        # "①"
        # "複製時の変更項目下に有"
        n1099 = local read "使用ON/OFFボタン_リセット用"() -> (w3182:T5)
        n1100 = local read "設定クラスタ_リセット"() -> (w3179:T4)
        n1101 = local read "CSV項目名_リセット用"() -> (w3177:T1)
        n1102 = local write "使用ON/OFFボタン_設定 9"(w3182) -> ()
        n1103 = local write "CSV項目名 9"(w3177) -> ()
        n1104 = local write "設定クラスタ_設定 9"(w3179) -> ()
        n1105 = Replace Array Subset(array=w3181, new element=w3179, index=8) -> (w3180:T2[])
      }
      frame "キャンセル10" {
        # "④"
        # "複製時の変更項目\n①②　④\nグローバル変数\n③\n指標値"
        # "③"
        # "②"
        # "①"
        # "複製時の変更項目下に有"
        n1106 = local read "使用ON/OFFボタン_リセット用"() -> (w3188:T5)
        n1107 = local read "設定クラスタ_リセット"() -> (w3185:T4)
        n1108 = local read "CSV項目名_リセット用"() -> (w3183:T1)
        n1109 = local write "使用ON/OFFボタン_設定 10"(w3188) -> ()
        n1110 = local write "CSV項目名 10"(w3183) -> ()
        n1111 = local write "設定クラスタ_設定 10"(w3185) -> ()
        n1112 = Replace Array Subset(array=w3187, new element=w3185, index=9) -> (w3186:T2[])
      }
      frame "キャンセル11" {
        # "④"
        # "複製時の変更項目\n①②　④\nグローバル変数\n③\n指標値"
        # "③"
        # "②"
        # "①"
        # "複製時の変更項目下に有"
        n1113 = local read "使用ON/OFFボタン_リセット用"() -> (w3194:T5)
        n1114 = local read "設定クラスタ_リセット"() -> (w3191:T4)
        n1115 = local read "CSV項目名_リセット用"() -> (w3189:T1)
        n1116 = local write "使用ON/OFFボタン_設定 11"(w3194) -> ()
        n1117 = local write "CSV項目名 11"(w3189) -> ()
        n1118 = local write "設定クラスタ_設定 11"(w3191) -> ()
        n1119 = Replace Array Subset(array=w3193, new element=w3191, index=10) -> (w3192:T2[])
      }
      frame "キャンセル12" {
        # "④"
        # "複製時の変更項目\n①②　④\nグローバル変数\n③\n指標値"
        # "③"
        # "②"
        # "①"
        # "複製時の変更項目下に有"
        n1120 = local read "使用ON/OFFボタン_リセット用"() -> (w3200:T5)
        n1121 = local read "設定クラスタ_リセット"() -> (w3197:T4)
        n1122 = local read "CSV項目名_リセット用"() -> (w3195:T1)
        n1123 = local write "使用ON/OFFボタン_設定 12"(w3200) -> ()
        n1124 = local write "CSV項目名 12"(w3195) -> ()
        n1125 = local write "設定クラスタ_設定 12"(w3197) -> ()
        n1126 = Replace Array Subset(array=w3199, new element=w3197, index=11) -> (w3198:T2[])
      }
      frame "設定変更1" {
        # "品番・品名クラスタ_設定を表示器へ転記"
        # "オブジェクトのオリジナルはここに置いてある\n①使用ON/OFFボタン_設定\n②No設定クラスタ_設定\n③キャンセルボタン\n④設定クラスタ_設定"
        # "測定モード設定時の動作"
        # "設定項目毎にケースを作成\n設定変更1のケースは複製不可"
        n1127 = for {
          N: 1 -> [_]
          tunnel: "設定クラスタ_設定1" -> [w3210]
          tunnel: "設定クラスタ_設定1" -> [w3208]
          n1128 = Unbundle By Name(w3210) -> ("測定モード"=w3209:u16)
          n1129 = case shown="0, デフォルト" w3209 {
            tunnel: w3208 -> [w3212 w3222 w3232]
            tunnel: [w3211 w3221 w3231] -> w3207
            frame 1 {
              # "連続測定モードの場合MAXとMINを表示する"
              n1130 = for {
                N: 1 -> [_]
                tunnel: w3212 -> [w3220]
                tunnel: [w3214] -> w3211
                w3217 = ""
                n1131 = Bundle By Name(cluster=w3220, "実測値MAX"="MAX", "実測値MIN"="MIN", "実測値(MAX)"=w3217, "実測値(MIN)"=w3217) -> (w3214:T2)
                n1132 = property on="実測値(MIN)" class="Str"("DisabledEnum"=T8."Enabled" ("無効")) -> ()  [unwired: 2 in, 2 out]
                n1133 = property on="実測値MIN" class="Str"("DisabledEnum"=T8."Enabled" ("無効")) -> ()  [unwired: 2 in, 2 out]
              }
            }
            frame 2 {
              # "連続測定モードの場合MAXとMINを表示する"
              n1134 = for {
                N: 1 -> [_]
                tunnel: w3222 -> [w3230]
                tunnel: [w3224] -> w3221
                w3227 = ""
                n1135 = Bundle By Name(cluster=w3230, "実測値MAX"="MAX", "実測値MIN"="MIN", "実測値(MAX)"=w3227, "実測値(MIN)"=w3227) -> (w3224:T2)
                n1136 = property on="実測値(MIN)" class="Str"("DisabledEnum"=T8."Enabled" ("無効")) -> ()  [unwired: 2 in, 2 out]
                n1137 = property on="実測値MIN" class="Str"("DisabledEnum"=T8."Enabled" ("無効")) -> ()  [unwired: 2 in, 2 out]
              }
            }
            frame 0, Default {
              n1138 = for {
                N: 1 -> [_]
                tunnel: w3232 -> [w3241]
                tunnel: [w3234] -> w3231
                n1139 = Bundle By Name(cluster=w3241, "実測値(MAX)"="", "実測値MAX"="値", "実測値(MIN)"="", "実測値MIN"="") -> (w3234:T2)
                n1140 = property on="実測値(MIN)" class="Str"("DisabledEnum"=T8."Disabled and Grayed Out" ("無効")) -> ()  [unwired: 2 in, 2 out]
                n1141 = property on="実測値MIN" class="Str"("DisabledEnum"=T8."Disabled and Grayed Out" ("無効")) -> ()  [unwired: 2 in, 2 out]
              }
            }
          }
          n1142 = local write "設定クラスタ_設定1"(w3207) -> ()
        }
        n1143 = property on="品番・品名クラスタ_設定" class="Clust (指定)"() -> ("Value"=w3206:T3)  [unwired: 2 in, 2 out]
        n1144 = property on="品番・品名クラスタ_設定 _表示器" class="Clust (指定)"("Value"=w3206) -> ()  [unwired: 2 in, 2 out]
        n1145 = Replace Array Subset(array=w3204, new element="設定クラスタ_設定1", index=0) -> (w3201:T2[])
        n1146 = local write "値転記用配列"(w3201) -> ()
      }
      frame "設定変更2" {
        # "③"
        # "①"
        # "オブジェクトのオリジナルはここに置いてある\n①使用ON/OFFボタン_設定\n②No設定クラスタ_設定\n③キャンセルボタン\n④設定クラスタ_設定"
        # "測定モード設定時の動作"
        # "※複製する場合このケースを複製\n複製時変更項目\n①ケース名\n②ローカル変数\n③指標値"
        n1147 = for {
          N: 1 -> [_]
          tunnel: "設定クラスタ_設定 2" -> [w3250]
          tunnel: "設定クラスタ_設定 2" -> [w3248]
          # "②"
          n1148 = Unbundle By Name(w3250) -> ("測定モード"=w3249:u16)
          n1149 = case shown="1" w3249 {
            tunnel: w3248 -> [w3252 w3262 w3272]
            tunnel: [w3251 w3261 w3271] -> w3247
            frame 1 {
              # "連続測定モードの場合MAXとMINを表示する"
              n1150 = for {
                N: 1 -> [_]
                tunnel: w3252 -> [w3260]
                tunnel: [w3254] -> w3251
                w3257 = ""
                n1151 = Bundle By Name(cluster=w3260, "実測値MAX"="MAX", "実測値MIN"="MIN", "実測値(MAX)"=w3257, "実測値(MIN)"=w3257) -> (w3254:T2)
                n1152 = property on="実測値(MIN)" class="Str"("DisabledEnum"=T8."Enabled" ("無効")) -> ()  [unwired: 2 in, 2 out]
                n1153 = property on="実測値MIN" class="Str"("DisabledEnum"=T8."Enabled" ("無効")) -> ()  [unwired: 2 in, 2 out]
              }
            }
            frame 2 {
              # "連続測定モードの場合MAXとMINを表示する"
              n1154 = for {
                N: 1 -> [_]
                tunnel: w3262 -> [w3270]
                tunnel: [w3264] -> w3261
                w3267 = ""
                n1155 = Bundle By Name(cluster=w3270, "実測値MAX"="MAX", "実測値MIN"="MIN", "実測値(MAX)"=w3267, "実測値(MIN)"=w3267) -> (w3264:T2)
                n1156 = property on="実測値(MIN)" class="Str"("DisabledEnum"=T8."Enabled" ("無効")) -> ()  [unwired: 2 in, 2 out]
                n1157 = property on="実測値MIN" class="Str"("DisabledEnum"=T8."Enabled" ("無効")) -> ()  [unwired: 2 in, 2 out]
              }
            }
            frame 0, Default {
              n1158 = for {
                N: 1 -> [_]
                tunnel: w3272 -> [w3281]
                tunnel: [w3274] -> w3271
                n1159 = Bundle By Name(cluster=w3281, "実測値(MAX)"="", "実測値MAX"="値", "実測値(MIN)"="", "実測値MIN"="") -> (w3274:T2)
                n1160 = property on="実測値(MIN)" class="Str"("DisabledEnum"=T8."Disabled and Grayed Out" ("無効")) -> ()  [unwired: 2 in, 2 out]
                n1161 = property on="実測値MIN" class="Str"("DisabledEnum"=T8."Disabled and Grayed Out" ("無効")) -> ()  [unwired: 2 in, 2 out]
              }
            }
          }
          n1162 = local write "設定クラスタ_設定 2"(w3247) -> ()
        }
        n1163 = Replace Array Subset(array=w3245, new element="設定クラスタ_設定 2", index=1) -> (w3242:T2[])
        n1164 = local write "値転記用配列"(w3242) -> ()
      }
      frame "設定変更3" {
        # "③"
        # "①"
        # "オブジェクトのオリジナルはここに置いてある\n①使用ON/OFFボタン_設定\n②No設定クラスタ_設定\n③キャンセルボタン\n④設定クラスタ_設定"
        # "測定モード設定時の動作"
        # "※複製する場合このケースを複製\n複製時変更項目\n①ケース名\n②ローカル変数\n③指標値"
        n1165 = for {
          N: 1 -> [_]
          tunnel: "設定クラスタ_設定 3" -> [w3290]
          tunnel: "設定クラスタ_設定 3" -> [w3288]
          # "②"
          n1166 = Unbundle By Name(w3290) -> ("測定モード"=w3289:u16)
          n1167 = case shown="0, デフォルト" w3289 {
            tunnel: w3288 -> [w3292 w3302 w3312]
            tunnel: [w3291 w3301 w3311] -> w3287
            frame 1 {
              # "連続測定モードの場合MAXとMINを表示する"
              n1168 = for {
                N: 1 -> [_]
                tunnel: w3292 -> [w3300]
                tunnel: [w3294] -> w3291
                w3297 = ""
                n1169 = Bundle By Name(cluster=w3300, "実測値MAX"="MAX", "実測値MIN"="MIN", "実測値(MAX)"=w3297, "実測値(MIN)"=w3297) -> (w3294:T2)
                n1170 = property on="実測値(MIN)" class="Str"("DisabledEnum"=T8."Enabled" ("無効")) -> ()  [unwired: 2 in, 2 out]
                n1171 = property on="実測値MIN" class="Str"("DisabledEnum"=T8."Enabled" ("無効")) -> ()  [unwired: 2 in, 2 out]
              }
            }
            frame 2 {
              # "連続測定モードの場合MAXとMINを表示する"
              n1172 = for {
                N: 1 -> [_]
                tunnel: w3302 -> [w3310]
                tunnel: [w3304] -> w3301
                w3307 = ""
                n1173 = Bundle By Name(cluster=w3310, "実測値MAX"="MAX", "実測値MIN"="MIN", "実測値(MAX)"=w3307, "実測値(MIN)"=w3307) -> (w3304:T2)
                n1174 = property on="実測値(MIN)" class="Str"("DisabledEnum"=T8."Enabled" ("無効")) -> ()  [unwired: 2 in, 2 out]
                n1175 = property on="実測値MIN" class="Str"("DisabledEnum"=T8."Enabled" ("無効")) -> ()  [unwired: 2 in, 2 out]
              }
            }
            frame 0, Default {
              n1176 = for {
                N: 1 -> [_]
                tunnel: w3312 -> [w3321]
                tunnel: [w3314] -> w3311
                n1177 = Bundle By Name(cluster=w3321, "実測値(MAX)"="", "実測値MAX"="値", "実測値(MIN)"="", "実測値MIN"="") -> (w3314:T2)
                n1178 = property on="実測値(MIN)" class="Str"("DisabledEnum"=T8."Disabled and Grayed Out" ("無効")) -> ()  [unwired: 2 in, 2 out]
                n1179 = property on="実測値MIN" class="Str"("DisabledEnum"=T8."Disabled and Grayed Out" ("無効")) -> ()  [unwired: 2 in, 2 out]
              }
            }
          }
          n1180 = local write "設定クラスタ_設定 3"(w3287) -> ()
        }
        n1181 = Replace Array Subset(array=w3285, new element="設定クラスタ_設定 3", index=2) -> (w3282:T2[])
        n1182 = local write "値転記用配列"(w3282) -> ()
      }
      frame "設定変更4" {
        # "③"
        # "①"
        # "オブジェクトのオリジナルはここに置いてある\n①使用ON/OFFボタン_設定\n②No設定クラスタ_設定\n③キャンセルボタン\n④設定クラスタ_設定"
        # "測定モード設定時の動作"
        # "※複製する場合このケースを複製\n複製時変更項目\n①ケース名\n②ローカル変数\n③指標値"
        n1183 = for {
          N: 1 -> [_]
          tunnel: "設定クラスタ_設定 4" -> [w3330]
          tunnel: "設定クラスタ_設定 4" -> [w3328]
          # "②"
          n1184 = Unbundle By Name(w3330) -> ("測定モード"=w3329:u16)
          n1185 = case shown="1" w3329 {
            tunnel: w3328 -> [w3332 w3342 w3352]
            tunnel: [w3331 w3341 w3351] -> w3327
            frame 1 {
              # "連続測定モードの場合MAXとMINを表示する"
              n1186 = for {
                N: 1 -> [_]
                tunnel: w3332 -> [w3340]
                tunnel: [w3334] -> w3331
                w3337 = ""
                n1187 = Bundle By Name(cluster=w3340, "実測値MAX"="MAX", "実測値MIN"="MIN", "実測値(MAX)"=w3337, "実測値(MIN)"=w3337) -> (w3334:T2)
                n1188 = property on="実測値(MIN)" class="Str"("DisabledEnum"=T8."Enabled" ("無効")) -> ()  [unwired: 2 in, 2 out]
                n1189 = property on="実測値MIN" class="Str"("DisabledEnum"=T8."Enabled" ("無効")) -> ()  [unwired: 2 in, 2 out]
              }
            }
            frame 2 {
              # "連続測定モードの場合MAXとMINを表示する"
              n1190 = for {
                N: 1 -> [_]
                tunnel: w3342 -> [w3350]
                tunnel: [w3344] -> w3341
                w3347 = ""
                n1191 = Bundle By Name(cluster=w3350, "実測値MAX"="MAX", "実測値MIN"="MIN", "実測値(MAX)"=w3347, "実測値(MIN)"=w3347) -> (w3344:T2)
                n1192 = property on="実測値(MIN)" class="Str"("DisabledEnum"=T8."Enabled" ("無効")) -> ()  [unwired: 2 in, 2 out]
                n1193 = property on="実測値MIN" class="Str"("DisabledEnum"=T8."Enabled" ("無効")) -> ()  [unwired: 2 in, 2 out]
              }
            }
            frame 0, Default {
              n1194 = for {
                N: 1 -> [_]
                tunnel: w3352 -> [w3361]
                tunnel: [w3354] -> w3351
                n1195 = Bundle By Name(cluster=w3361, "実測値(MAX)"="", "実測値MAX"="値", "実測値(MIN)"="", "実測値MIN"="") -> (w3354:T2)
                n1196 = property on="実測値(MIN)" class="Str"("DisabledEnum"=T8."Disabled and Grayed Out" ("無効")) -> ()  [unwired: 2 in, 2 out]
                n1197 = property on="実測値MIN" class="Str"("DisabledEnum"=T8."Disabled and Grayed Out" ("無効")) -> ()  [unwired: 2 in, 2 out]
              }
            }
          }
          n1198 = local write "設定クラスタ_設定 4"(w3327) -> ()
        }
        n1199 = Replace Array Subset(array=w3325, new element="設定クラスタ_設定 4", index=3) -> (w3322:T2[])
        n1200 = local write "値転記用配列"(w3322) -> ()
      }
      frame "設定変更5" {
        # "③"
        # "①"
        # "オブジェクトのオリジナルはここに置いてある\n①使用ON/OFFボタン_設定\n②No設定クラスタ_設定\n③キャンセルボタン\n④設定クラスタ_設定"
        # "測定モード設定時の動作"
        # "※複製する場合このケースを複製\n複製時変更項目\n①ケース名\n②ローカル変数\n③指標値"
        n1201 = for {
          N: 1 -> [_]
          tunnel: "設定クラスタ_設定 5" -> [w3370]
          tunnel: "設定クラスタ_設定 5" -> [w3368]
          # "②"
          n1202 = Unbundle By Name(w3370) -> ("測定モード"=w3369:u16)
          n1203 = case shown="1" w3369 {
            tunnel: w3368 -> [w3372 w3382 w3392]
            tunnel: [w3371 w3381 w3391] -> w3367
            frame 1 {
              # "連続測定モードの場合MAXとMINを表示する"
              n1204 = for {
                N: 1 -> [_]
                tunnel: w3372 -> [w3380]
                tunnel: [w3374] -> w3371
                w3377 = ""
                n1205 = Bundle By Name(cluster=w3380, "実測値MAX"="MAX", "実測値MIN"="MIN", "実測値(MAX)"=w3377, "実測値(MIN)"=w3377) -> (w3374:T2)
                n1206 = property on="実測値(MIN)" class="Str"("DisabledEnum"=T8."Enabled" ("無効")) -> ()  [unwired: 2 in, 2 out]
                n1207 = property on="実測値MIN" class="Str"("DisabledEnum"=T8."Enabled" ("無効")) -> ()  [unwired: 2 in, 2 out]
              }
            }
            frame 2 {
              # "連続測定モードの場合MAXとMINを表示する"
              n1208 = for {
                N: 1 -> [_]
                tunnel: w3382 -> [w3390]
                tunnel: [w3384] -> w3381
                w3387 = ""
                n1209 = Bundle By Name(cluster=w3390, "実測値MAX"="MAX", "実測値MIN"="MIN", "実測値(MAX)"=w3387, "実測値(MIN)"=w3387) -> (w3384:T2)
                n1210 = property on="実測値(MIN)" class="Str"("DisabledEnum"=T8."Enabled" ("無効")) -> ()  [unwired: 2 in, 2 out]
                n1211 = property on="実測値MIN" class="Str"("DisabledEnum"=T8."Enabled" ("無効")) -> ()  [unwired: 2 in, 2 out]
              }
            }
            frame 0, Default {
              n1212 = for {
                N: 1 -> [_]
                tunnel: w3392 -> [w3401]
                tunnel: [w3394] -> w3391
                n1213 = Bundle By Name(cluster=w3401, "実測値(MAX)"="", "実測値MAX"="値", "実測値(MIN)"="", "実測値MIN"="") -> (w3394:T2)
                n1214 = property on="実測値(MIN)" class="Str"("DisabledEnum"=T8."Disabled and Grayed Out" ("無効")) -> ()  [unwired: 2 in, 2 out]
                n1215 = property on="実測値MIN" class="Str"("DisabledEnum"=T8."Disabled and Grayed Out" ("無効")) -> ()  [unwired: 2 in, 2 out]
              }
            }
          }
          n1216 = local write "設定クラスタ_設定 5"(w3367) -> ()
        }
        n1217 = Replace Array Subset(array=w3365, new element="設定クラスタ_設定 5", index=4) -> (w3362:T2[])
        n1218 = local write "値転記用配列"(w3362) -> ()
      }
      frame "設定変更6" {
        # "③"
        # "①"
        # "オブジェクトのオリジナルはここに置いてある\n①使用ON/OFFボタン_設定\n②No設定クラスタ_設定\n③キャンセルボタン\n④設定クラスタ_設定"
        # "測定モード設定時の動作"
        # "※複製する場合このケースを複製\n複製時変更項目\n①ケース名\n②ローカル変数\n③指標値"
        n1219 = for {
          N: 1 -> [_]
          tunnel: "設定クラスタ_設定 6" -> [w3410]
          tunnel: "設定クラスタ_設定 6" -> [w3408]
          # "②"
          n1220 = Unbundle By Name(w3410) -> ("測定モード"=w3409:u16)
          n1221 = case shown="1" w3409 {
            tunnel: w3408 -> [w3412 w3422 w3432]
            tunnel: [w3411 w3421 w3431] -> w3407
            frame 1 {
              # "連続測定モードの場合MAXとMINを表示する"
              n1222 = for {
                N: 1 -> [_]
                tunnel: w3412 -> [w3420]
                tunnel: [w3414] -> w3411
                w3417 = ""
                n1223 = Bundle By Name(cluster=w3420, "実測値MAX"="MAX", "実測値MIN"="MIN", "実測値(MAX)"=w3417, "実測値(MIN)"=w3417) -> (w3414:T2)
                n1224 = property on="実測値(MIN)" class="Str"("DisabledEnum"=T8."Enabled" ("無効")) -> ()  [unwired: 2 in, 2 out]
                n1225 = property on="実測値MIN" class="Str"("DisabledEnum"=T8."Enabled" ("無効")) -> ()  [unwired: 2 in, 2 out]
              }
            }
            frame 2 {
              # "連続測定モードの場合MAXとMINを表示する"
              n1226 = for {
                N: 1 -> [_]
                tunnel: w3422 -> [w3430]
                tunnel: [w3424] -> w3421
                w3427 = ""
                n1227 = Bundle By Name(cluster=w3430, "実測値MAX"="MAX", "実測値MIN"="MIN", "実測値(MAX)"=w3427, "実測値(MIN)"=w3427) -> (w3424:T2)
                n1228 = property on="実測値(MIN)" class="Str"("DisabledEnum"=T8."Enabled" ("無効")) -> ()  [unwired: 2 in, 2 out]
                n1229 = property on="実測値MIN" class="Str"("DisabledEnum"=T8."Enabled" ("無効")) -> ()  [unwired: 2 in, 2 out]
              }
            }
            frame 0, Default {
              n1230 = for {
                N: 1 -> [_]
                tunnel: w3432 -> [w3441]
                tunnel: [w3434] -> w3431
                n1231 = Bundle By Name(cluster=w3441, "実測値(MAX)"="", "実測値MAX"="値", "実測値(MIN)"="", "実測値MIN"="") -> (w3434:T2)
                n1232 = property on="実測値(MIN)" class="Str"("DisabledEnum"=T8."Disabled and Grayed Out" ("無効")) -> ()  [unwired: 2 in, 2 out]
                n1233 = property on="実測値MIN" class="Str"("DisabledEnum"=T8."Disabled and Grayed Out" ("無効")) -> ()  [unwired: 2 in, 2 out]
              }
            }
          }
          n1234 = local write "設定クラスタ_設定 6"(w3407) -> ()
        }
        n1235 = Replace Array Subset(array=w3405, new element="設定クラスタ_設定 6", index=5) -> (w3402:T2[])
        n1236 = local write "値転記用配列"(w3402) -> ()
      }
      frame "設定変更7" {
        # "③"
        # "①"
        # "オブジェクトのオリジナルはここに置いてある\n①使用ON/OFFボタン_設定\n②No設定クラスタ_設定\n③キャンセルボタン\n④設定クラスタ_設定"
        # "測定モード設定時の動作"
        # "※複製する場合このケースを複製\n複製時変更項目\n①ケース名\n②ローカル変数\n③指標値"
        n1237 = for {
          N: 1 -> [_]
          tunnel: "設定クラスタ_設定 7" -> [w3450]
          tunnel: "設定クラスタ_設定 7" -> [w3448]
          # "②"
          n1238 = Unbundle By Name(w3450) -> ("測定モード"=w3449:u16)
          n1239 = case shown="1" w3449 {
            tunnel: w3448 -> [w3452 w3462 w3472]
            tunnel: [w3451 w3461 w3471] -> w3447
            frame 1 {
              # "連続測定モードの場合MAXとMINを表示する"
              n1240 = for {
                N: 1 -> [_]
                tunnel: w3452 -> [w3460]
                tunnel: [w3454] -> w3451
                w3457 = ""
                n1241 = Bundle By Name(cluster=w3460, "実測値MAX"="MAX", "実測値MIN"="MIN", "実測値(MAX)"=w3457, "実測値(MIN)"=w3457) -> (w3454:T2)
                n1242 = property on="実測値(MIN)" class="Str"("DisabledEnum"=T8."Enabled" ("無効")) -> ()  [unwired: 2 in, 2 out]
                n1243 = property on="実測値MIN" class="Str"("DisabledEnum"=T8."Enabled" ("無効")) -> ()  [unwired: 2 in, 2 out]
              }
            }
            frame 2 {
              # "連続測定モードの場合MAXとMINを表示する"
              n1244 = for {
                N: 1 -> [_]
                tunnel: w3462 -> [w3470]
                tunnel: [w3464] -> w3461
                w3467 = ""
                n1245 = Bundle By Name(cluster=w3470, "実測値MAX"="MAX", "実測値MIN"="MIN", "実測値(MAX)"=w3467, "実測値(MIN)"=w3467) -> (w3464:T2)
                n1246 = property on="実測値(MIN)" class="Str"("DisabledEnum"=T8."Enabled" ("無効")) -> ()  [unwired: 2 in, 2 out]
                n1247 = property on="実測値MIN" class="Str"("DisabledEnum"=T8."Enabled" ("無効")) -> ()  [unwired: 2 in, 2 out]
              }
            }
            frame 0, Default {
              n1248 = for {
                N: 1 -> [_]
                tunnel: w3472 -> [w3481]
                tunnel: [w3474] -> w3471
                n1249 = Bundle By Name(cluster=w3481, "実測値(MAX)"="", "実測値MAX"="値", "実測値(MIN)"="", "実測値MIN"="") -> (w3474:T2)
                n1250 = property on="実測値(MIN)" class="Str"("DisabledEnum"=T8."Disabled and Grayed Out" ("無効")) -> ()  [unwired: 2 in, 2 out]
                n1251 = property on="実測値MIN" class="Str"("DisabledEnum"=T8."Disabled and Grayed Out" ("無効")) -> ()  [unwired: 2 in, 2 out]
              }
            }
          }
          n1252 = local write "設定クラスタ_設定 7"(w3447) -> ()
        }
        n1253 = Replace Array Subset(array=w3445, new element="設定クラスタ_設定 7", index=6) -> (w3442:T2[])
        n1254 = local write "値転記用配列"(w3442) -> ()
      }
      frame "設定変更8" {
        # "③"
        # "①"
        # "オブジェクトのオリジナルはここに置いてある\n①使用ON/OFFボタン_設定\n②No設定クラスタ_設定\n③キャンセルボタン\n④設定クラスタ_設定"
        # "測定モード設定時の動作"
        # "※複製する場合このケースを複製\n複製時変更項目\n①ケース名\n②ローカル変数\n③指標値"
        n1255 = for {
          N: 1 -> [_]
          tunnel: "設定クラスタ_設定 8" -> [w3490]
          tunnel: "設定クラスタ_設定 8" -> [w3488]
          # "②"
          n1256 = Unbundle By Name(w3490) -> ("測定モード"=w3489:u16)
          n1257 = case shown="1" w3489 {
            tunnel: w3488 -> [w3492 w3502 w3512]
            tunnel: [w3491 w3501 w3511] -> w3487
            frame 1 {
              # "連続測定モードの場合MAXとMINを表示する"
              n1258 = for {
                N: 1 -> [_]
                tunnel: w3492 -> [w3500]
                tunnel: [w3494] -> w3491
                w3497 = ""
                n1259 = Bundle By Name(cluster=w3500, "実測値MAX"="MAX", "実測値MIN"="MIN", "実測値(MAX)"=w3497, "実測値(MIN)"=w3497) -> (w3494:T2)
                n1260 = property on="実測値(MIN)" class="Str"("DisabledEnum"=T8."Enabled" ("無効")) -> ()  [unwired: 2 in, 2 out]
                n1261 = property on="実測値MIN" class="Str"("DisabledEnum"=T8."Enabled" ("無効")) -> ()  [unwired: 2 in, 2 out]
              }
            }
            frame 2 {
              # "連続測定モードの場合MAXとMINを表示する"
              n1262 = for {
                N: 1 -> [_]
                tunnel: w3502 -> [w3510]
                tunnel: [w3504] -> w3501
                w3507 = ""
                n1263 = Bundle By Name(cluster=w3510, "実測値MAX"="MAX", "実測値MIN"="MIN", "実測値(MAX)"=w3507, "実測値(MIN)"=w3507) -> (w3504:T2)
                n1264 = property on="実測値(MIN)" class="Str"("DisabledEnum"=T8."Enabled" ("無効")) -> ()  [unwired: 2 in, 2 out]
                n1265 = property on="実測値MIN" class="Str"("DisabledEnum"=T8."Enabled" ("無効")) -> ()  [unwired: 2 in, 2 out]
              }
            }
            frame 0, Default {
              n1266 = for {
                N: 1 -> [_]
                tunnel: w3512 -> [w3521]
                tunnel: [w3514] -> w3511
                n1267 = Bundle By Name(cluster=w3521, "実測値(MAX)"="", "実測値MAX"="値", "実測値(MIN)"="", "実測値MIN"="") -> (w3514:T2)
                n1268 = property on="実測値(MIN)" class="Str"("DisabledEnum"=T8."Disabled and Grayed Out" ("無効")) -> ()  [unwired: 2 in, 2 out]
                n1269 = property on="実測値MIN" class="Str"("DisabledEnum"=T8."Disabled and Grayed Out" ("無効")) -> ()  [unwired: 2 in, 2 out]
              }
            }
          }
          n1270 = local write "設定クラスタ_設定 8"(w3487) -> ()
        }
        n1271 = Replace Array Subset(array=w3485, new element="設定クラスタ_設定 8", index=7) -> (w3482:T2[])
        n1272 = local write "値転記用配列"(w3482) -> ()
      }
      frame "設定変更9" {
        # "③"
        # "①"
        # "オブジェクトのオリジナルはここに置いてある\n①使用ON/OFFボタン_設定\n②No設定クラスタ_設定\n③キャンセルボタン\n④設定クラスタ_設定"
        # "測定モード設定時の動作"
        # "※複製する場合このケースを複製\n複製時変更項目\n①ケース名\n②ローカル変数\n③指標値"
        n1273 = for {
          N: 1 -> [_]
          tunnel: "設定クラスタ_設定 9" -> [w3530]
          tunnel: "設定クラスタ_設定 9" -> [w3528]
          # "②"
          n1274 = Unbundle By Name(w3530) -> ("測定モード"=w3529:u16)
          n1275 = case shown="1" w3529 {
            tunnel: w3528 -> [w3532 w3542 w3552]
            tunnel: [w3531 w3541 w3551] -> w3527
            frame 1 {
              # "連続測定モードの場合MAXとMINを表示する"
              n1276 = for {
                N: 1 -> [_]
                tunnel: w3532 -> [w3540]
                tunnel: [w3534] -> w3531
                w3537 = ""
                n1277 = Bundle By Name(cluster=w3540, "実測値MAX"="MAX", "実測値MIN"="MIN", "実測値(MAX)"=w3537, "実測値(MIN)"=w3537) -> (w3534:T2)
                n1278 = property on="実測値(MIN)" class="Str"("DisabledEnum"=T8."Enabled" ("無効")) -> ()  [unwired: 2 in, 2 out]
                n1279 = property on="実測値MIN" class="Str"("DisabledEnum"=T8."Enabled" ("無効")) -> ()  [unwired: 2 in, 2 out]
              }
            }
            frame 2 {
              # "連続測定モードの場合MAXとMINを表示する"
              n1280 = for {
                N: 1 -> [_]
                tunnel: w3542 -> [w3550]
                tunnel: [w3544] -> w3541
                w3547 = ""
                n1281 = Bundle By Name(cluster=w3550, "実測値MAX"="MAX", "実測値MIN"="MIN", "実測値(MAX)"=w3547, "実測値(MIN)"=w3547) -> (w3544:T2)
                n1282 = property on="実測値(MIN)" class="Str"("DisabledEnum"=T8."Enabled" ("無効")) -> ()  [unwired: 2 in, 2 out]
                n1283 = property on="実測値MIN" class="Str"("DisabledEnum"=T8."Enabled" ("無効")) -> ()  [unwired: 2 in, 2 out]
              }
            }
            frame 0, Default {
              n1284 = for {
                N: 1 -> [_]
                tunnel: w3552 -> [w3561]
                tunnel: [w3554] -> w3551
                n1285 = Bundle By Name(cluster=w3561, "実測値(MAX)"="", "実測値MAX"="値", "実測値(MIN)"="", "実測値MIN"="") -> (w3554:T2)
                n1286 = property on="実測値(MIN)" class="Str"("DisabledEnum"=T8."Disabled and Grayed Out" ("無効")) -> ()  [unwired: 2 in, 2 out]
                n1287 = property on="実測値MIN" class="Str"("DisabledEnum"=T8."Disabled and Grayed Out" ("無効")) -> ()  [unwired: 2 in, 2 out]
              }
            }
          }
          n1288 = local write "設定クラスタ_設定 9"(w3527) -> ()
        }
        n1289 = Replace Array Subset(array=w3525, new element="設定クラスタ_設定 9", index=8) -> (w3522:T2[])
        n1290 = local write "値転記用配列"(w3522) -> ()
      }
      frame "設定変更10" {
        # "③"
        # "①"
        # "オブジェクトのオリジナルはここに置いてある\n①使用ON/OFFボタン_設定\n②No設定クラスタ_設定\n③キャンセルボタン\n④設定クラスタ_設定"
        # "測定モード設定時の動作"
        # "※複製する場合このケースを複製\n複製時変更項目\n①ケース名\n②ローカル変数\n③指標値"
        n1291 = for {
          N: 1 -> [_]
          tunnel: "設定クラスタ_設定 10" -> [w3570]
          tunnel: "設定クラスタ_設定 10" -> [w3568]
          # "②"
          n1292 = Unbundle By Name(w3570) -> ("測定モード"=w3569:u16)
          n1293 = case shown="1" w3569 {
            tunnel: w3568 -> [w3572 w3582 w3592]
            tunnel: [w3571 w3581 w3591] -> w3567
            frame 1 {
              # "連続測定モードの場合MAXとMINを表示する"
              n1294 = for {
                N: 1 -> [_]
                tunnel: w3572 -> [w3580]
                tunnel: [w3574] -> w3571
                w3577 = ""
                n1295 = Bundle By Name(cluster=w3580, "実測値MAX"="MAX", "実測値MIN"="MIN", "実測値(MAX)"=w3577, "実測値(MIN)"=w3577) -> (w3574:T2)
                n1296 = property on="実測値(MIN)" class="Str"("DisabledEnum"=T8."Enabled" ("無効")) -> ()  [unwired: 2 in, 2 out]
                n1297 = property on="実測値MIN" class="Str"("DisabledEnum"=T8."Enabled" ("無効")) -> ()  [unwired: 2 in, 2 out]
              }
            }
            frame 2 {
              # "連続測定モードの場合MAXとMINを表示する"
              n1298 = for {
                N: 1 -> [_]
                tunnel: w3582 -> [w3590]
                tunnel: [w3584] -> w3581
                w3587 = ""
                n1299 = Bundle By Name(cluster=w3590, "実測値MAX"="MAX", "実測値MIN"="MIN", "実測値(MAX)"=w3587, "実測値(MIN)"=w3587) -> (w3584:T2)
                n1300 = property on="実測値(MIN)" class="Str"("DisabledEnum"=T8."Enabled" ("無効")) -> ()  [unwired: 2 in, 2 out]
                n1301 = property on="実測値MIN" class="Str"("DisabledEnum"=T8."Enabled" ("無効")) -> ()  [unwired: 2 in, 2 out]
              }
            }
            frame 0, Default {
              n1302 = for {
                N: 1 -> [_]
                tunnel: w3592 -> [w3601]
                tunnel: [w3594] -> w3591
                n1303 = Bundle By Name(cluster=w3601, "実測値(MAX)"="", "実測値MAX"="値", "実測値(MIN)"="", "実測値MIN"="") -> (w3594:T2)
                n1304 = property on="実測値(MIN)" class="Str"("DisabledEnum"=T8."Disabled and Grayed Out" ("無効")) -> ()  [unwired: 2 in, 2 out]
                n1305 = property on="実測値MIN" class="Str"("DisabledEnum"=T8."Disabled and Grayed Out" ("無効")) -> ()  [unwired: 2 in, 2 out]
              }
            }
          }
          n1306 = local write "設定クラスタ_設定 10"(w3567) -> ()
        }
        n1307 = Replace Array Subset(array=w3565, new element="設定クラスタ_設定 10", index=9) -> (w3562:T2[])
        n1308 = local write "値転記用配列"(w3562) -> ()
      }
      frame "設定変更11" {
        # "③"
        # "①"
        # "オブジェクトのオリジナルはここに置いてある\n①使用ON/OFFボタン_設定\n②No設定クラスタ_設定\n③キャンセルボタン\n④設定クラスタ_設定"
        # "測定モード設定時の動作"
        # "※複製する場合このケースを複製\n複製時変更項目\n①ケース名\n②ローカル変数\n③指標値"
        n1309 = for {
          N: 1 -> [_]
          tunnel: "設定クラスタ_設定 11" -> [w3610]
          tunnel: "設定クラスタ_設定 11" -> [w3608]
          # "②"
          n1310 = Unbundle By Name(w3610) -> ("測定モード"=w3609:u16)
          n1311 = case shown="1" w3609 {
            tunnel: w3608 -> [w3612 w3622 w3632]
            tunnel: [w3611 w3621 w3631] -> w3607
            frame 1 {
              # "連続測定モードの場合MAXとMINを表示する"
              n1312 = for {
                N: 1 -> [_]
                tunnel: w3612 -> [w3620]
                tunnel: [w3614] -> w3611
                w3617 = ""
                n1313 = Bundle By Name(cluster=w3620, "実測値MAX"="MAX", "実測値MIN"="MIN", "実測値(MAX)"=w3617, "実測値(MIN)"=w3617) -> (w3614:T2)
                n1314 = property on="実測値(MIN)" class="Str"("DisabledEnum"=T8."Enabled" ("無効")) -> ()  [unwired: 2 in, 2 out]
                n1315 = property on="実測値MIN" class="Str"("DisabledEnum"=T8."Enabled" ("無効")) -> ()  [unwired: 2 in, 2 out]
              }
            }
            frame 2 {
              # "連続測定モードの場合MAXとMINを表示する"
              n1316 = for {
                N: 1 -> [_]
                tunnel: w3622 -> [w3630]
                tunnel: [w3624] -> w3621
                w3627 = ""
                n1317 = Bundle By Name(cluster=w3630, "実測値MAX"="MAX", "実測値MIN"="MIN", "実測値(MAX)"=w3627, "実測値(MIN)"=w3627) -> (w3624:T2)
                n1318 = property on="実測値(MIN)" class="Str"("DisabledEnum"=T8."Enabled" ("無効")) -> ()  [unwired: 2 in, 2 out]
                n1319 = property on="実測値MIN" class="Str"("DisabledEnum"=T8."Enabled" ("無効")) -> ()  [unwired: 2 in, 2 out]
              }
            }
            frame 0, Default {
              n1320 = for {
                N: 1 -> [_]
                tunnel: w3632 -> [w3641]
                tunnel: [w3634] -> w3631
                n1321 = Bundle By Name(cluster=w3641, "実測値(MAX)"="", "実測値MAX"="値", "実測値(MIN)"="", "実測値MIN"="") -> (w3634:T2)
                n1322 = property on="実測値(MIN)" class="Str"("DisabledEnum"=T8."Disabled and Grayed Out" ("無効")) -> ()  [unwired: 2 in, 2 out]
                n1323 = property on="実測値MIN" class="Str"("DisabledEnum"=T8."Disabled and Grayed Out" ("無効")) -> ()  [unwired: 2 in, 2 out]
              }
            }
          }
          n1324 = local write "設定クラスタ_設定 11"(w3607) -> ()
        }
        n1325 = Replace Array Subset(array=w3605, new element="設定クラスタ_設定 11", index=10) -> (w3602:T2[])
        n1326 = local write "値転記用配列"(w3602) -> ()
      }
      frame "設定変更12" {
        # "③"
        # "①"
        # "オブジェクトのオリジナルはここに置いてある\n①使用ON/OFFボタン_設定\n②No設定クラスタ_設定\n③キャンセルボタン\n④設定クラスタ_設定"
        # "測定モード設定時の動作"
        # "※複製する場合このケースを複製\n複製時変更項目\n①ケース名\n②ローカル変数\n③指標値"
        n1327 = for {
          N: 1 -> [_]
          tunnel: "設定クラスタ_設定 12" -> [w3650]
          tunnel: "設定クラスタ_設定 12" -> [w3648]
          # "②"
          n1328 = Unbundle By Name(w3650) -> ("測定モード"=w3649:u16)
          n1329 = case shown="1" w3649 {
            tunnel: w3648 -> [w3652 w3662 w3672]
            tunnel: [w3651 w3661 w3671] -> w3647
            frame 1 {
              # "連続測定モードの場合MAXとMINを表示する"
              n1330 = for {
                N: 1 -> [_]
                tunnel: w3652 -> [w3660]
                tunnel: [w3654] -> w3651
                w3657 = ""
                n1331 = Bundle By Name(cluster=w3660, "実測値MAX"="MAX", "実測値MIN"="MIN", "実測値(MAX)"=w3657, "実測値(MIN)"=w3657) -> (w3654:T2)
                n1332 = property on="実測値(MIN)" class="Str"("DisabledEnum"=T8."Enabled" ("無効")) -> ()  [unwired: 2 in, 2 out]
                n1333 = property on="実測値MIN" class="Str"("DisabledEnum"=T8."Enabled" ("無効")) -> ()  [unwired: 2 in, 2 out]
              }
            }
            frame 2 {
              # "連続測定モードの場合MAXとMINを表示する"
              n1334 = for {
                N: 1 -> [_]
                tunnel: w3662 -> [w3670]
                tunnel: [w3664] -> w3661
                w3667 = ""
                n1335 = Bundle By Name(cluster=w3670, "実測値MAX"="MAX", "実測値MIN"="MIN", "実測値(MAX)"=w3667, "実測値(MIN)"=w3667) -> (w3664:T2)
                n1336 = property on="実測値(MIN)" class="Str"("DisabledEnum"=T8."Enabled" ("無効")) -> ()  [unwired: 2 in, 2 out]
                n1337 = property on="実測値MIN" class="Str"("DisabledEnum"=T8."Enabled" ("無効")) -> ()  [unwired: 2 in, 2 out]
              }
            }
            frame 0, Default {
              n1338 = for {
                N: 1 -> [_]
                tunnel: w3672 -> [w3681]
                tunnel: [w3674] -> w3671
                n1339 = Bundle By Name(cluster=w3681, "実測値(MAX)"="", "実測値MAX"="値", "実測値(MIN)"="", "実測値MIN"="") -> (w3674:T2)
                n1340 = property on="実測値(MIN)" class="Str"("DisabledEnum"=T8."Disabled and Grayed Out" ("無効")) -> ()  [unwired: 2 in, 2 out]
                n1341 = property on="実測値MIN" class="Str"("DisabledEnum"=T8."Disabled and Grayed Out" ("無効")) -> ()  [unwired: 2 in, 2 out]
              }
            }
          }
          n1342 = local write "設定クラスタ_設定 12"(w3647) -> ()
        }
        n1343 = Replace Array Subset(array=w3645, new element="設定クラスタ_設定 12", index=11) -> (w3642:T2[])
        n1344 = local write "値転記用配列"(w3642) -> ()
      }
    }
  }
  n1345 = while {
    tunnel: w6 -> [w3686]
    tunnel: w5 -> [w3685]
    tunnel: [w3684] -> w11
    tunnel: [w3683] -> w10
    stop <- w3682 stop-if-true
    n1346 = event "イベントストラクチャ" shown="[3] \"ゲージ確認ボタン\": 値変更" {
      selector: _ -> [_ _ _ _ _ _ _ _ _ _ _ _ _ _ _ _ _ _ _ _ _ _ _ _ _ _ _ _]
      dyn-events: _ -> [_ _ _ _ _ _ _ _ _ _ _ _ _ _ _ _ _ _ _ _ _ _ _ _ _ _ _ _]
      timeout: _ -> [_ _ _ _ _ _ _ _ _ _ _ _ _ _ _ _ _ _ _ _ _ _ _ _ _ _ _ _]
      tunnel: w3686 -> [w3690 w3696 w3700 w3710 w3714 w3720 w3725 w3730 w3735 w3740 w3745 w3750 w3755 w3760 w3765 w3770 w3774 w3779 w3784 w3789 w3794 w3799 w3804 w3809 w3814 w3819 w3824 w3829]
      tunnel: w3685 -> [w3689 w3694 w3699 w3709 w3712 w3719 w3724 w3729 w3734 w3739 w3744 w3749 w3754 w3759 w3764 w3769 w3772 w3777 w3782 w3787 w3792 w3797 w3802 w3807 w3812 w3817 w3822 w3827]
      tunnel: [_ _ w3698 _ w3713 w3717 w3722 w3727 w3732 w3737 w3742 w3747 w3752 w3757 w3762 w3767 w3773 w3778 w3783 w3788 w3793 w3798 w3803 w3808 w3813 w3818 w3823 w3828] -> w3684
      tunnel: [w3688 w3693 w3697 w3708 w3711 w3716 w3721 w3726 w3731 w3736 w3741 w3746 w3751 w3756 w3761 w3766 w3771 w3776 w3781 w3786 w3791 w3796 w3801 w3806 w3811 w3816 w3821 w3826] -> w3683
      tunnel: [TRUE TRUE _ _ _ _ _ _ _ _ _ _ _ _ _ _ _ _ _ _ _ _ _ _ _ _ _ _] -> w3682
      event "登録ボタン": Value Change {
        # "設定項目画面の登録ボタンが押された時に動作"
        n1347 = event-data() -> ()  [unwired: 1 in, 1 out]
        n1348 = Enqueue Element(queue=w3690, element="登録", error in (no error)=w3689) -> (error out=w3688:errorcluster)  [unwired: 1 in, 2 out]
      }
      event "キャンセルして戻るボタン": Value Change {
        # "設定画面のキャンセルボタンが押された時に動作"
        # "trueになったら停止"
        n1349 = event-data() -> ()  [unwired: 1 in, 1 out]
        n1350 = Enqueue Element(queue=w3696, element="キャンセルして戻る", error in (no error)=w3694) -> (error out=w3693:errorcluster)  [unwired: 1 in, 2 out]
      }
      event "初期化ボタン": Value Change {
        n1351 = event-data() -> ()  [unwired: 1 in, 1 out]
        n1352 = Enqueue Element(queue=w3700, element="初期化", error in (no error)=w3699) -> (queue out=w3698:refnum<queue>, error out=w3697:errorcluster)  [unwired: 1 in, 1 out]
      }
      event "ゲージ確認ボタン": Value Change {
        n1353 = event-data() -> ("OldVal"=w3706:bool)  [unwired: 1 in, 5 out]
        n1354 = Enqueue Element(queue=w3710, element="ゲージ確認", error in (no error)=w3709) -> (error out=w3708:errorcluster)  [unwired: 1 in, 2 out]
        n1355 = Select(t=TRUE, s=w3706, f=FALSE) -> (s? t:f=w3703:bool)
        n1356 = local write "ゲージ確認ボタンBOOL"("ゲージ確認ボタン") -> ()
        n1357 = global write "VISA停止_G.vi" "VISA停止_\nグローバル"(w3703) -> ()
      }
      event "CSV保存先フォルダ": Value Change {
        # "このケースは複製不可"
        # "品番・品名・CSVパスの値が変更された時に動作"
        n1358 = event-data() -> ()  [unwired: 1 in, 1 out]
        n1359 = Enqueue Element(queue=w3714, element="設定変更1", error in (no error)=w3712) -> (queue out=w3713:refnum<queue>, error out=w3711:errorcluster)  [unwired: 1 in, 1 out]
      }
      event Value Change {
        # "①"
        # "複製時の変更項目\n①キューの設定"
        n1360 = event-data() -> ()  [unwired: 1 in, 1 out]
        n1361 = Enqueue Element(queue=w3720, element="設定変更2", error in (no error)=w3719) -> (queue out=w3717:refnum<queue>, error out=w3716:errorcluster)  [unwired: 1 in, 1 out]
      }
      event Value Change {
        n1362 = event-data() -> ()  [unwired: 1 in, 1 out]
        n1363 = Enqueue Element(queue=w3725, element="設定変更3", error in (no error)=w3724) -> (queue out=w3722:refnum<queue>, error out=w3721:errorcluster)  [unwired: 1 in, 1 out]
      }
      event Value Change {
        # "①"
        # "複製時の変更項目\n①キューの設定"
        n1364 = event-data() -> ()  [unwired: 1 in, 1 out]
        n1365 = Enqueue Element(queue=w3730, element="設定変更4", error in (no error)=w3729) -> (queue out=w3727:refnum<queue>, error out=w3726:errorcluster)  [unwired: 1 in, 1 out]
      }
      event Value Change {
        # "①"
        # "複製時の変更項目\n①キューの設定"
        n1366 = event-data() -> ()  [unwired: 1 in, 1 out]
        n1367 = Enqueue Element(queue=w3735, element="設定変更5", error in (no error)=w3734) -> (queue out=w3732:refnum<queue>, error out=w3731:errorcluster)  [unwired: 1 in, 1 out]
      }
      event Value Change {
        # "①"
        # "複製時の変更項目\n①キューの設定"
        n1368 = event-data() -> ()  [unwired: 1 in, 1 out]
        n1369 = Enqueue Element(queue=w3740, element="設定変更6", error in (no error)=w3739) -> (queue out=w3737:refnum<queue>, error out=w3736:errorcluster)  [unwired: 1 in, 1 out]
      }
      event Value Change {
        # "①"
        # "複製時の変更項目\n①キューの設定"
        n1370 = event-data() -> ()  [unwired: 1 in, 1 out]
        n1371 = Enqueue Element(queue=w3745, element="設定変更7", error in (no error)=w3744) -> (queue out=w3742:refnum<queue>, error out=w3741:errorcluster)  [unwired: 1 in, 1 out]
      }
      event Value Change {
        # "①"
        # "複製時の変更項目\n①キューの設定"
        n1372 = event-data() -> ()  [unwired: 1 in, 1 out]
        n1373 = Enqueue Element(queue=w3750, element="設定変更8", error in (no error)=w3749) -> (queue out=w3747:refnum<queue>, error out=w3746:errorcluster)  [unwired: 1 in, 1 out]
      }
      event Value Change {
        # "①"
        # "複製時の変更項目\n①キューの設定"
        n1374 = event-data() -> ()  [unwired: 1 in, 1 out]
        n1375 = Enqueue Element(queue=w3755, element="設定変更9", error in (no error)=w3754) -> (queue out=w3752:refnum<queue>, error out=w3751:errorcluster)  [unwired: 1 in, 1 out]
      }
      event Value Change {
        # "①"
        # "複製時の変更項目\n①キューの設定"
        n1376 = event-data() -> ()  [unwired: 1 in, 1 out]
        n1377 = Enqueue Element(queue=w3760, element="設定変更10", error in (no error)=w3759) -> (queue out=w3757:refnum<queue>, error out=w3756:errorcluster)  [unwired: 1 in, 1 out]
      }
      event Value Change {
        # "①"
        # "複製時の変更項目\n①キューの設定"
        n1378 = event-data() -> ()  [unwired: 1 in, 1 out]
        n1379 = Enqueue Element(queue=w3765, element="設定変更11", error in (no error)=w3764) -> (queue out=w3762:refnum<queue>, error out=w3761:errorcluster)  [unwired: 1 in, 1 out]
      }
      event Value Change {
        # "①"
        # "複製時の変更項目\n①キューの設定"
        n1380 = event-data() -> ()  [unwired: 1 in, 1 out]
        n1381 = Enqueue Element(queue=w3770, element="設定変更12", error in (no error)=w3769) -> (queue out=w3767:refnum<queue>, error out=w3766:errorcluster)  [unwired: 1 in, 1 out]
      }
      event Value Change {
        n1382 = event-data() -> ()  [unwired: 1 in, 1 out]
        n1383 = Enqueue Element(queue=w3774, element="キャンセル1", error in (no error)=w3772) -> (queue out=w3773:refnum<queue>, error out=w3771:errorcluster)  [unwired: 1 in, 1 out]
      }
      event Value Change {
        n1384 = event-data() -> ()  [unwired: 1 in, 1 out]
        n1385 = Enqueue Element(queue=w3779, element="キャンセル2", error in (no error)=w3777) -> (queue out=w3778:refnum<queue>, error out=w3776:errorcluster)  [unwired: 1 in, 1 out]
      }
      event Value Change {
        n1386 = event-data() -> ()  [unwired: 1 in, 1 out]
        n1387 = Enqueue Element(queue=w3784, element="キャンセル3", error in (no error)=w3782) -> (queue out=w3783:refnum<queue>, error out=w3781:errorcluster)  [unwired: 1 in, 1 out]
      }
      event Value Change {
        n1388 = event-data() -> ()  [unwired: 1 in, 1 out]
        n1389 = Enqueue Element(queue=w3789, element="キャンセル4", error in (no error)=w3787) -> (queue out=w3788:refnum<queue>, error out=w3786:errorcluster)  [unwired: 1 in, 1 out]
      }
      event Value Change {
        n1390 = event-data() -> ()  [unwired: 1 in, 1 out]
        n1391 = Enqueue Element(queue=w3794, element="キャンセル5", error in (no error)=w3792) -> (queue out=w3793:refnum<queue>, error out=w3791:errorcluster)  [unwired: 1 in, 1 out]
      }
      event Value Change {
        n1392 = event-data() -> ()  [unwired: 1 in, 1 out]
        n1393 = Enqueue Element(queue=w3799, element="キャンセル6", error in (no error)=w3797) -> (queue out=w3798:refnum<queue>, error out=w3796:errorcluster)  [unwired: 1 in, 1 out]
      }
      event Value Change {
        n1394 = event-data() -> ()  [unwired: 1 in, 1 out]
        n1395 = Enqueue Element(queue=w3804, element="キャンセル7", error in (no error)=w3802) -> (queue out=w3803:refnum<queue>, error out=w3801:errorcluster)  [unwired: 1 in, 1 out]
      }
      event Value Change {
        n1396 = event-data() -> ()  [unwired: 1 in, 1 out]
        n1397 = Enqueue Element(queue=w3809, element="キャンセル8", error in (no error)=w3807) -> (queue out=w3808:refnum<queue>, error out=w3806:errorcluster)  [unwired: 1 in, 1 out]
      }
      event Value Change {
        n1398 = event-data() -> ()  [unwired: 1 in, 1 out]
        n1399 = Enqueue Element(queue=w3814, element="キャンセル9", error in (no error)=w3812) -> (queue out=w3813:refnum<queue>, error out=w3811:errorcluster)  [unwired: 1 in, 1 out]
      }
      event Value Change {
        n1400 = event-data() -> ()  [unwired: 1 in, 1 out]
        n1401 = Enqueue Element(queue=w3819, element="キャンセル10", error in (no error)=w3817) -> (queue out=w3818:refnum<queue>, error out=w3816:errorcluster)  [unwired: 1 in, 1 out]
      }
      event Value Change {
        n1402 = event-data() -> ()  [unwired: 1 in, 1 out]
        n1403 = Enqueue Element(queue=w3824, element="キャンセル11", error in (no error)=w3822) -> (queue out=w3823:refnum<queue>, error out=w3821:errorcluster)  [unwired: 1 in, 1 out]
      }
      event Value Change {
        n1404 = event-data() -> ()  [unwired: 1 in, 1 out]
        n1405 = Enqueue Element(queue=w3829, element="キャンセル12", error in (no error)=w3827) -> (queue out=w3828:refnum<queue>, error out=w3826:errorcluster)  [unwired: 1 in, 1 out]
      }
    }
  }
  n1406 = Release Queue(queue=w11, error in (no error)=w10) -> (error out=→"キューのエラー":errorcluster)  [unwired: 1 in, 2 out]
  n1407 = while {
    i -> [w3831]
    stop <- w3832 stop-if-true
    n1408 = case shown="1" w3831 {
      tunnel: [TRUE _] -> w3832
      frame 1 {
      }
      frame 0, Default {
        n1409 = while {
          stop <- w3834 stop-if-true
          n1410 = flat-sequence {
            tunnel: [TRUE] -> w3834
            frame #0 {
            }
          }
        }
      }
    }
  }
